vi "H2O_DIAL_NCAR_4CH_v4.08.vi"() -> ()   [LabVIEW 2012]
uses:
  C:/Users/H2ODial/Desktop/Shared Telescope WV DIAL Code/Libraries and VIs/PowerMeterCommands.dll
  Libraries and VIs/PowerMeterCommands.dll
  <vilib>/DAQmx/write.llb/DAQmx Write (Digital 1D Bool NChan 1Samp 1Line).vi
  <vilib>/DAQmx/miscellaneous.llb/DAQmx Fill In Error Info.vi
  <vilib>/Analysis/baseanly.llb/Mean (DBL).vi
  AMCS_Data.vi
  Libraries and VIs/Scalar_Data.vi
  <vilib>/Analysis/NI_AALBase.lvlib
  Libraries and VIs/Scalar_Data_2.vi
  Libraries and VIs/Scalar_Data_4.vi
  Libraries and VIs/Scalar_Data_3.vi
  Libraries and VIs/CLDevIFace.dll
panel:
  out "FileHour":i32=20
  out "L_Count":i32=53610
  out "sigma_off_total":dbl[](array[numeric])=[5.237977287539916e-25, 5.210394736135076e-25, 5.182925586949714e-25, 5.155569869487791e-25, 5.128327607320838e-25, 5.101198818125548e-25, 5.074183513766137e-25, 5.047281700299452e-25, 5.020493378072102e-25, 4.993818541757595e-25, 4.967257180403445e-25, 4.940809277499799e-25, 4.914474811031665e-25, 4.888253753539835e-25, 4.862146072166262e-25, 4.836151728727555e-25, 4.810270679757114e-25, 4.7845028765711135e-25, 4.7588482653375005e-25, 4.733306787104272e-25, 4.707878377890851e-25, 4.682562968723741e-25, 4.657360485698113e-25, 4.632270850042273e-25, 4.607293978174461e-25, 4.582429781742665e-25, 4.557678167708119e-25, 4.533039038377526e-25, 4.508512291468661e-25, 4.484097820168311e-25, 4.459795513173839e-25, 4.435605254768827e-25, 4.411526924848054e-25, 4.387560398991586e-25, 4.363705548510036e-25, 4.339962240489646e-25, 4.3163303378483935e-25, 4.292809699388025e-25, 4.269400179831349e-25, 4.246101629883972e-25, 4.222913896270031e-25, 4.199836821781227e-25, 4.176870245324587e-25, 4.154014001969199e-25, 4.1312679229794556e-25, 4.10863183586778e-25, 4.0861055644288118e-25, 4.0636889287851403e-25, 4.041381745427012e-25, 4.019183827248936e-25, 3.997094983583401e-25, 3.9751150202537046e-25, 3.953243739588023e-25, 3.9314809404746634e-25, 3.9098264183856214e-25, 3.888279965410497e-25, 3.8668413702954256e-25, 3.845510418470829e-25, 3.8242868920787765e-25, 3.8031705700147897e-25, 3.782161227940215e-25, 3.761258638329626e-25, 3.74046257048381e-25, 3.7197727905642295e-25, 3.69918906161745e-25, 3.678711143600706e-25, 3.6583387934050425e-25, 3.638071764885887e-25, 3.617909808876586e-25, 3.59785267321608e-25, 3.577900102772319e-25, 3.558051839461918e-25, 3.538307622269321e-25, 3.5186671872697243e-25, 3.4991302676454615e-25, 3.479696593706232e-25, 3.460365892905833e-25, 3.441137889863693e-25, 3.422012306375155e-25, 3.4029888614344406e-25, 3.384067271245277e-25, 3.3652472492411824e-25, 3.346528506092826e-25, 3.3279107497319426e-25, 3.309393685355381e-25, 3.2909770154454064e-25, 3.272660439778772e-25, 3.2544436554389533e-25, 3.2363263568278233e-25, 3.2183082356811116e-25, 3.2003889810704124e-25, 3.1825682794209234e-25, 3.1648458145178674e-25, 3.1472212675167257e-25, 3.1296943169518588e-25, 3.1122646387407036e-25, 3.094931906200432e-25, 3.0776957900440946e-25, 3.060555958395204e-25, 3.043512076792759e-25, 3.026563808190885e-25, 3.009710812972571e-25, 2.9929527489462136e-25, 2.976289271354231e-25, 2.9597200328732653e-25, 2.9432446836195626e-25, 2.9268628711468796e-25, 2.910574240452457e-25, 2.8943784339725194e-25, 2.8782750915848116e-25, 2.862263850606443e-25, 2.8463443457918976e-25, 2.830516209331176e-25, 2.814779070844048e-25, 2.799132557377377e-25, 2.783576293398477e-25, 2.768109900787332e-25, 2.7527329988309794e-25, 2.7374452042136163e-25, 2.7222461310065917e-25, 2.7071353906571954e-25, 2.6921125919761984e-25, 2.677177341122853e-25, 2.662329241593387e-25, 2.647567894198339e-25, 2.632892897051999e-25, 2.618303845545271e-25, 2.60380033233239e-25, 2.589381947301631e-25, 2.575048277552024e-25, 2.5607989073700278e-25, 2.546633418200283e-25, 2.532551388614268e-25, 2.5185523942817305e-25, 2.5046360079339746e-25, 2.4908017993263377e-25, 2.477049335209051e-25, 2.4633781792772914e-25, 2.4497878921362335e-25, 2.4362780312554467e-25, 2.4228481509187937e-25, 2.4094978021817806e-25, 2.3962265328170672e-25, 2.3830338872635978e-25, 2.3699194065693153e-25, 2.356882628338278e-25, 2.3439230866617374e-25, 2.3310403120653215e-25, 2.318233831442806e-25, 2.305503167989909e-25, 2.29284784112487e-25, 2.280267366433339e-25, 2.267761255593697e-25, 2.2553290162907755e-25, 2.242970152141067e-25, 2.2306841626327338e-25, 2.21847054301743e-25, 2.206328784250053e-25, 2.1942583728887336e-25, 2.182258791026811e-25, 2.1703295161891593e-25, 2.1584700212551692e-25, 2.1466797743708636e-25, 2.1349582388520993e-25, 2.1233048731028347e-25, 2.11171913052587e-25, 2.1002004594155447e-25, 2.0887483028986794e-25, 2.077362098819431e-25, 2.0660412796644763e-25, 2.0547852724613812e-25, 2.0435934987176713e-25, 2.0324653743177702e-25, 2.0214003094407255e-25, 2.0103977084918826e-25, 1.9994569700219043e-25, 1.9885774866543093e-25, 1.977758645016903e-25, 1.9669998256711833e-25, 1.9563004030651965e-25, 1.9456597454736256e-25, 1.9350772149357237e-25, 1.9245521672543692e-25, 1.9140839518990637e-25, 1.9036719120338527e-25, 1.893315384469969e-25, 1.883013699654113e-25, 1.8727661816903515e-25, 1.8625721483087474e-25, 1.8524309109152708e-25, 1.842341774622776e-25, 1.8323040382575362e-25, 1.8223169944561692e-25, 1.812379929715831e-25, 1.8024921244357534e-25, 1.7926528530972796e-25, 1.7828613842771046e-25, 1.7731169808504013e-25, 1.763418900060532e-25, 1.753766393760346e-25, 1.7441587084910652e-25, 1.7345950857732995e-25, 1.7250747622294322e-25, 1.7155969698576046e-25, 1.7061609363195063e-25, 1.6967658851005867e-25, 1.6874110359226843e-25, 1.6780956049685245e-25, 1.6688188052514317e-25, 1.659579846970255e-25, 1.65037793787203e-25, 1.6412122836350012e-25, 1.6320820883466068e-25, 1.6229865548899808e-25, 1.6139248854231656e-25, 1.604896281851196e-25, 1.5958999464323058e-25, 1.5869350821540768e-25, 1.5780008933988883e-25, 1.5690965865250916e-25, 1.5602213703998908e-25, 1.551374457088728e-25, 1.5425550624278814e-25, 1.533762406758044e-25, 1.5249957155722975e-25, 1.5162542201789217e-25, 1.5075371585159662e-25, 1.498843775813426e-25, 1.490173325365196e-25, 1.4815250692768405e-25, 1.4728982792886032e-25, 1.4642922375724935e-25, 1.4557062374752215e-25, 1.4471395844199516e-25, 1.4385915966670965e-25, 1.4300616061440924e-25, 1.4215489593499951e-25, 1.413053018080556e-25, 1.4045731604317913e-25, 1.396108781452575e-25, 1.3876592941232874e-25, 1.3792241301169086e-25, 1.3708027406484068e-25, 1.3623945973169855e-25, 1.353999192808714e-25, 1.3456160418411176e-25, 1.3372446818099923e-25, 1.3288846735970857e-25, 1.3205356022789798e-25, 1.312197077893849e-25, 1.3038687360747626e-25, 1.295550238736152e-25, 1.2872412747034491e-25, 1.2789415602527627e-25, 1.2706508397867747e-25, 1.2623688862167277e-25, 1.2540955015928698e-25, 1.2458305174038967e-25, 1.2375737951859152e-25, 1.229325226582947e-25, 1.2210847339251814e-25, 1.2128522703422863e-25, 1.2046278200669743e-25, 1.196411398536186e-25, 1.1882030524688986e-25, 1.1800028600144816e-25, 1.1718109306926895e-25, 1.163627405308368e-25, 1.15545245599885e-25, 1.1472862858176296e-25, 1.1391291287321645e-25, 1.1309812492832123e-25, 1.1228429421236803e-25, 1.1147145318495405e-25, 1.106596372364196e-25, 1.0984888464412128e-25, 1.0903923652647968e-25]
  out "sigma_on_total":dbl[](array[numeric])=[2.0666817520319192e-23, 2.0593109014659378e-23, 2.051872195703395e-23, 2.044367039943362e-23, 2.0367968427579014e-23, 2.0291630153667858e-23, 2.0214669713004497e-23, 2.013710125383857e-23, 2.0058938935289517e-23, 1.9980196920012705e-23, 1.9900889367712726e-23, 1.982103043065158e-23, 1.974063424772205e-23, 1.9659714939377124e-23, 1.9578286601133224e-23, 1.9496363299838326e-23, 1.94139590669971e-23, 1.9331087894484655e-23, 1.9247763730742107e-23, 1.9164000472908787e-23, 1.9079811965513556e-23, 1.8995211993589887e-23, 1.891021427856131e-23, 1.8824832474616412e-23, 1.8739080164441743e-23, 1.8652970853194722e-23, 1.856651796748594e-23, 1.847973484883867e-23, 1.8392634751030097e-23, 1.8305230836795774e-23, 1.8217536172790674e-23, 1.8129563728772394e-23, 1.804132637094709e-23, 1.7952836861392256e-23, 1.7864107854248313e-23, 1.7775151892040785e-23, 1.7685981403601007e-23, 1.7596608701730099e-23, 1.750704597915161e-23, 1.741730530788138e-23, 1.732739863541907e-23, 1.7237337782890177e-23, 1.7147134443297577e-23, 1.7056800179881565e-23, 1.6966346422793058e-23, 1.6875784468765622e-23, 1.6785125478376762e-23, 1.669438047521509e-23, 1.6603560344433225e-23, 1.6512675831053983e-23, 1.6421737538036553e-23, 1.6330755927613498e-23, 1.6239741316742248e-23, 1.6148703879339332e-23, 1.60576536436924e-23, 1.596660049173217e-23, 1.5875554159429494e-23, 1.5784524235547823e-23, 1.569352016050113e-23, 1.5602551228033537e-23, 1.5511626581860282e-23, 1.5420755218867996e-23, 1.5329945986273844e-23, 1.523920758294004e-23, 1.5148548559068197e-23, 1.505797731630872e-23, 1.4967502107612878e-23, 1.4877131038805498e-23, 1.4786872066923908e-23, 1.4696733001603334e-23, 1.4606721505852176e-23, 1.4516845096236347e-23, 1.4427111143132646e-23, 1.4337526872006215e-23, 1.4248099363455505e-23, 1.415883555427735e-23, 1.4069742237945813e-23, 1.3980826066400498e-23, 1.3892093549366116e-23, 1.3803551056859226e-23, 1.371520481892078e-23, 1.36270609278781e-23, 1.3539125337562842e-23, 1.3451403866865457e-23, 1.3363902198427942e-23, 1.32766258816433e-23, 1.3189580332947156e-23, 1.3102770837058438e-23, 1.301620254824897e-23, 1.2929880492812047e-23, 1.2843809568021667e-23, 1.2757994545539253e-23, 1.2672440071893687e-23, 1.2587150670157126e-23, 1.2502130741345343e-23, 1.241738456470468e-23, 1.2332916301710505e-23, 1.224872999440041e-23, 1.2164829569109985e-23, 1.2081218837654899e-23, 1.1997901497162132e-23, 1.1914881134062081e-23, 1.1832161223390686e-23, 1.1749745131680931e-23, 1.1667636117668732e-23, 1.1585837334629664e-23, 1.1504351830839475e-23, 1.1423182552440761e-23, 1.1342332343652275e-23, 1.1261803949102824e-23, 1.1181600015104835e-23, 1.1101723091192649e-23, 1.1022175631912938e-23, 1.0942959997845036e-23, 1.086407845764062e-23, 1.0785533189291783e-23, 1.070732628140394e-23, 1.0629459735209997e-23, 1.0551935465825773e-23, 1.0474755303750616e-23, 1.0397920996360129e-23, 1.0321434209390468e-23, 1.0245296528176247e-23, 1.0169509459831485e-23, 1.0094074433518565e-23, 1.0018992803312205e-23, 9.944265848224308e-24, 9.869894775025579e-24, 9.795880718494269e-24, 9.72222474305659e-24, 9.648927844628867e-24, 9.575990951759402e-24, 9.50341492676679e-24, 9.431200567532366e-24, 9.359348608388352e-24, 9.287859721227397e-24, 9.216734517894411e-24, 9.14597355017344e-24, 9.075577311930703e-24, 9.005546240155555e-24, 8.935880715787577e-24, 8.86658106558043e-24, 8.797647562896506e-24, 8.729080429115388e-24, 8.660879834613277e-24, 8.593045900337285e-24, 8.525578698151898e-24, 8.458478252785328e-24, 8.391744542743954e-24, 8.325377501414138e-24, 8.259377017376947e-24, 8.193742936655974e-24, 8.128475063566239e-24, 8.063573160991183e-24, 7.99903695161361e-24, 7.934866120048426e-24, 7.87106031214778e-24, 7.807619137288812e-24, 7.744542168412114e-24, 7.681828943883436e-24, 7.619478967515311e-24, 7.557491710029518e-24, 7.495866609952388e-24, 7.434603074147054e-24, 7.373700479036967e-24, 7.313158171455071e-24, 7.252975468799607e-24, 7.193151661058425e-24, 7.133686010591324e-24, 7.074577753436494e-24, 7.015826099592955e-24, 6.95743023461463e-24, 6.89938931969699e-24, 6.841702492422132e-24, 6.784368867806759e-24, 6.727387538848196e-24, 6.67075757722047e-24, 6.61447803395679e-24, 6.558547939965e-24, 6.502966306993674e-24, 6.447732128116975e-24, 6.392844378064806e-24, 6.33830201474097e-24, 6.28410397847858e-24, 6.23024919382799e-24, 6.1767365695383454e-24, 6.123564999129965e-24, 6.070733361880125e-24, 6.0182405226492204e-24, 5.966085332987157e-24, 5.914266631645723e-24, 5.8627832445313994e-24, 5.811633985898412e-24, 5.7608176585519654e-24, 5.710333053788294e-24, 5.66017895307138e-24, 5.610354127145003e-24, 5.560857337543025e-24, 5.5116873361021744e-24, 5.4628428664272046e-24, 5.4143226631411985e-24, 5.3661254534434446e-24, 5.318249956485201e-24, 5.27069488426681e-24, 5.223458942376564e-24, 5.176540829250344e-24, 5.129939237757062e-24, 5.083652854692084e-24, 5.037680361483587e-24, 4.99202043452124e-24, 4.946671745361136e-24, 4.9016329609288464e-24, 4.8569027442871215e-24, 4.812479754472342e-24, 4.768362646904479e-24, 4.724550073562594e-24, 4.6810406839229e-24, 4.637833124122778e-24, 4.594926037999457e-24, 4.552318067336052e-24, 4.510007851680585e-24, 4.467994029014724e-24, 4.426275235567218e-24, 4.384850106461307e-24, 4.3437172757252515e-24, 4.302875376308277e-24, 4.262323040796395e-24, 4.222058901208864e-24, 4.182081589298348e-24, 4.142389736646627e-24, 4.102981975046665e-24, 4.063856936678659e-24, 4.0250132539999516e-24, 3.986449560294931e-24, 3.948164489555187e-24, 3.910156676643546e-24, 3.872424757723072e-24, 3.834967369951946e-24, 3.797783152259275e-24, 3.760870744768346e-24, 3.724228789468588e-24, 3.687855930080657e-24, 3.651750812271991e-24, 3.615912083862758e-24, 3.580338394607038e-24, 3.545028396812783e-24, 3.509980745031705e-24, 3.475194096334501e-24, 3.440667110332911e-24, 3.40639844943986e-24, 3.3723867788033646e-24, 3.33863076647876e-24, 3.305129083516007e-24, 3.271880403891816e-24, 3.238883404898292e-24, 3.2061367668408557e-24, 3.173639173491545e-24, 3.1413893117883693e-24, 3.1093858724187726e-24, 3.0776275491566985e-24, 3.0461130395819077e-24, 3.0148410447789974e-24, 2.983810269608433e-24, 2.9530194226199734e-24, 2.9224672160398477e-24, 2.8921523660272985e-24, 2.8620735925846947e-24, 2.8322296195392698e-24, 2.8026191749155588e-24, 2.773240990450988e-24, 2.744093802094081e-24, 2.7151763499066755e-24, 2.6864873778481257e-24, 2.6580256342491748e-24, 2.6297898714658192e-24, 2.601778846035958e-24, 2.5739913188856307e-24]
  out "background start":u32=269
  in  "Tab Control 2":enum32{"WV ND far", "WV ND near"}(tab)
  out "Water Vapor Number Density":dbl[][](graph)=[[1.726093583785998, 1.5693328403021882, 1.492935828673154, 1.447945915792696, 1.4070653390472017, 1.3254550070570101, 1.2804967879324003, 1.2804658654967171, 1.1579952104203475, 0.9405002139474755, 0.8165160638391011, 0.7588336527077482, 0.7354590874335223, 0.7949133332346723, 0.934908558804581, 1.2546910246889589, 1.7625302263189773, 2.0654043072611956, 1.7505301065732377, 1.188350440813126, 0.9885074031875984, 1.101505088269768, 1.2336330855194724, 1.3310674253591945, 1.505107272437263, 1.8254736972087702, 2.225603030680858, 2.067084599300453, 0.8832035531037339, 0.09437092170191938, 0.5395557458682886, 1.2140813710589395, 1.531090454107329, 1.5864605833339975, 1.5242315918950318, 1.3208543677687434, 1.1426796573454, 1.0502932702090415, 1.053417044203025, 1.1120228404679369, 0.8980388027038368, 0.8252375109823104, 0.7459206585905861, 0.6947605707599939, 0.5975172515547873, 0.4760902556721864, 0.4151454819859171, 0.39114402110892216, 0.37598278988553024, 0.34134053721693014, 0.29078994347279413, 0.27415101735234926, 0.3077369235432359, 0.3546026534730858, 0.46199415649911274, 0.5308578319039414, 0.5880944648414834, 0.8235212196286621, 1.2285880343893505, 2.882707728529924, 21.655039035254283, -1.2950791268227064, -15.65393062619791, -8.993125447341491, -5.175372303539384, -3.3856480323932954, -6.29508550326919, -7.154473265737363, -6.483534196194922, -9.265253216386386, -27.54820579914408, -4.723304671265731, 12.404282083102887, 2.1871104315302006, -2.728312257847411, -2.37955818251216, -0.8921430715770072, 0.0602736205824744, -0.33680772359773153, -1.5016597305177382, -3.146854610737365, 5.147107349586582, 2.5981969564643483, 1.927078112036158, -0.2019670065149347, -2.7680462725589408, -0.8640403008156559, -0.3802637288627016, -0.30703778771168194, 3.78203982209544, 6.186195002061386, -1.7005858912590297, -4.265240893190755, -3.1735701916943326, 0.5020833614372952, 3.237847342695031, 3.4070293883563316, 2.220676402431187, -0.36304323573622177, -2.50058383327132, -4.668332258495944, -6.411554489859993, -3.6540172117701606, 1.1929008673292896, 6.604569777453038, 9.439096094131198, -0.37592110290192393, -1.1973823785952542, -1.48647731353954, -4.840730889441363, -3.3418602691261685, -0.6598739403508244, 0.669104742362441, -0.6893546278444684, -10.4814271416847, -11.440111754869928, -0.3632022671713595, 0.6227468083328052, 13.218505806822774, 8.015075479380561, 4.061945777588537, -0.04892863519373536, -6.238185623258318, 18.53116155726855, 15.923168701202894, -3.9495930624327413, -5.7591651615962505, -2.835335920357439, -15.615692769445864, -8.050161480731097, -6.2988354876816945, 3.427472591088481, 9.602428466947865, -24.99205539862618, -21.730434892627393, 2.0254153667718473, 5.319236625213819, -4.231429520416637, 5.960092104774531, 9.175230031410537, 5.788798488819853, 1.2095983409811533, -4.077619187880176, 2.2911716100459993, 8.947839474381412, 1.5428868263761497, 1.1797809535068915, 6.502768356706267, -5.016648532788809, -8.952003568032467, -0.620404792879008, 24.678168336180246, 56.15693255842815, 15.239179864782777, 11.41921009773234, 9.58559110034771, -1.8378094145353232, -8.922747471661737, -10.47837694939924, 0.3826205789632058, 18.765420881082978, -27.679590849047152, -97.04153207449242, -10.013514694974337, 6.267103457434482, 5.2850126899119845, 14.69530339344026, 2.3301310125680486, 22.67928054652624, -4.859966072588231, -27.611523100524643, -5.388011297923277, 42.80888421591542, -10.55670454003978, -29.387589282014147, -13.771657285473296, -10.230767774708267, -15.406236525942628, -17.934779899787376, 7.866413980735036, -16.61338646328196, -33.72812563272742, -31.126096535992467, -6.559728776164742, 47.49568241841293, 13.927413516339834, -1.9103285022235699, 30.194286473319444, 21.421181182090656, 8.458291065822397, 64.4520154677842, 51.90400411679242, 36.48500116306378, 20.23053272363266, -21.8380131234608, 9.733997218213648, 17.755970175135474, 24.978768220528003, -16.798275313105552, -40.83054382894082, -72.77210575173487, -23.204625740736503, -12.922468776734748, 10.063889955334702, -12.711982906467439, -20.40456545648094, -13.878406439439372, -29.749691947295048, -4.076124591492557, 29.788213178427508, 6.248079314213002, -20.245927416281017, -13.548384416231665, -13.091969559034965, -12.979461901579612, -27.404428517975767, -28.82133765520021, -34.93474155125817, -17.456376797105253, -21.723899533014873, 8.609611112888343, 31.6981010680414, 21.03013721810904, -20.578242782300084, 33.02437661787703, 0.05405579004919296, 0.5355916211190656, 36.99850340913583, 14.120107902899404, 19.11249102647391, -23.861285040548577, -37.522374332023944, -28.734364047495777, 24.270546317192423, -42.885420861437105, 7.644261246136678, -10.35463621262086, -4.297514158130115, 7.187709131614377, -4.734831899416053, 48.535485170482076, 109.9250199786216, 19.771496935630168, -21.29480194803723, 7.10371336563834, -7.3594100417697, 28.30301499602303, -6.173312274600606, -48.473804438854806, -44.552722047320536, -16.388748920234434, -52.98268299759962, 35.83782137376554, 16.24116595319644, 9.54744614996322, 28.184236323160842, 21.73885851975668, 13.761566677706107, 58.90182142368742, 82.80959093536396, 97.24340862705938, -19.983802413261767, -110.5470598503176, -45.4894502592988, -12.240067151016795, -53.090407850417165, -6.950497574763418, -78.83310574737847, 10.93122749802334, -11.422884686238413, -159.94669283010876, -73.71618130213747, 9.079012315082618, -28.203429472131308, -56.05728304279368, -26.34758679382537, 0.0, 0.0, 0.0, 0.0]]
  out "Water Vapor Number Density 2":dbl[][](graph)=[[nan, nan, nan, nan, nan, nan, nan, nan, nan, nan, nan, nan, nan, nan, nan, nan, nan, nan, nan, nan, nan, nan, nan, nan, nan, nan, nan, nan, nan, nan, nan, nan, nan, nan, nan, nan, nan, nan, nan, nan, nan, nan, nan, nan, nan, nan, nan, nan, nan, nan, nan, nan, nan, nan, nan, nan, nan, nan, nan, nan, nan, nan, nan, nan, nan, nan, nan, nan, nan, nan, nan, nan, nan, nan, nan, nan, nan, nan, nan, nan, nan, nan, nan, nan, nan, nan, nan, nan, nan, nan, nan, nan, nan, nan, nan, nan, nan, nan, nan, nan, nan, nan, nan, nan, nan, nan, nan, nan, nan, nan, nan, nan, nan, nan, nan, nan, nan, nan, nan, nan, nan, nan, nan, nan, nan, nan, nan, nan, nan, nan, nan, nan, nan, nan, nan, nan, nan, nan, nan, nan, nan, nan, nan, nan, nan, nan, nan, nan, nan, nan, nan, nan, nan, nan, nan, nan, nan, nan, nan, nan, nan, nan, nan, nan, nan, nan, nan, nan, nan, nan, nan, nan, nan, nan, nan, nan, nan, nan, nan, nan, nan, nan, nan, nan, nan, nan, nan, nan, nan, nan, nan, nan, nan, nan, nan, nan, nan, nan, nan, nan, nan, nan, nan, nan, nan, nan, nan, nan, nan, nan, nan, nan, nan, nan, nan, nan, nan, nan, nan, nan, nan, nan, nan, nan, nan, nan, nan, nan, nan, nan, nan, nan, nan, nan, nan, nan, nan, nan, nan, nan, nan, nan, nan, nan, nan, nan, nan, nan, nan, nan, nan, nan, nan, nan, nan, nan, nan, nan, nan, nan, nan, nan, nan, nan, nan, nan, nan, nan, nan, nan, nan, nan, nan, nan, nan, nan, 0.0, 0.0, 0.0, 0.0]] caption="Water Vapor Number Density"
  out "RingBuffer offline near":dbl[][](array[numeric])
  out "RingBuffer aerosol near":dbl[][](array[numeric])
  in  "?":T1(tab)
  out "NRB":dbl[][](graph)=[[0.00038821040544486485, 0.0028581072475373126, 0.009664054878145745, 0.0218937455043181, 0.041585081911817263, 0.07907105171256666, 0.1517956195167564, 0.26417801899826343, 0.4035088182229872, 0.5650687115263837, 0.7608077401440904, 1.0057587682792892, 1.2933461609750239, 1.5966324534478469, 1.8616436253029935, 2.051331796764738, 2.160120670777728, 2.2276009194819837, 2.3041185987927006, 2.3534797914467314, 2.4144079717154505, 2.5498196394788026, 2.6670946659124346, 2.7292203147350245, 2.8081805686949957, 2.85157014135836, 2.8104801837455016, 2.52779119302893, 1.896358445357234, 1.4744417690314884, 1.9842591872797726, 3.185501611912857, 3.9632337336496595, 3.867773398872155, 3.446687058785667, 3.1391414455490154, 2.967862705818635, 2.835829374555156, 2.61630220135343, 2.2701613602887263, 1.9304871996773967, 1.7247991727133216, 1.6336047893811358, 1.5809857912833423, 1.4964246235970382, 1.3753026836922766, 1.2068633615280102, 0.9758258849560736, 0.7472068994762533, 0.5990670480551521, 0.5531735761691717, 0.5643122449388852, 0.6046034091465748, 0.6816394574095734, 0.7768790871537363, 0.8963666224831853, 1.0673032706932424, 1.1963682953128685, 1.113329958933323, 0.8104505672194267, 0.4712408220023341, 0.23636168910826832, 0.11093337571666789, 0.045649279610657616, 0.013827815106420362, 0.000595543364686196, -0.004059439261428629, -0.002311182614261961, 0.0011883714622039875, -0.0071350992474156815, -0.013583214093101, -0.009986650833171679, -0.009129851870763993, -0.007802145173723816, -0.007450071158263493, -0.005784710331142982, -0.004246214811760087, -0.0036513842538617087, -0.007639759654127067, -0.009499909569249076, -0.008196050807191971, -0.004014404234963711, -0.0025144302656745997, -0.006602038304925129, -0.006737511480302444, -0.010236280891107273, -0.018639054498064318, -0.013631519426649653, -0.00435649140769087, -0.007934433790837766, -0.008838747504431614, -0.009538302637566698, -0.0025601741269936887, -0.0008145882550386953, -0.006378604787752585, -0.006369112164930518, -0.010839258183081239, -0.006275890418726249, -0.0014874755507115693, -0.009137146169405736, -0.012711182042689725, -0.013910133853955842, -0.017011569135408258, -0.012799263424370013, -0.011249036980201734, -0.009491427382456405, -0.0003733679388180713, -0.007329445907503577, -0.008732421530258959, -0.010562733558625092, -0.017129887166000557, -0.013428203058959441, -0.007903693902916552, -0.0071477038674852365, -0.01108866845659684, -0.003265799105280196, 0.0011847288805150722, 0.00037549107141904574, -0.008054862709676584, -0.003856137038819446, -0.0002938238582222133, -0.008979477671617945, -0.013823588439693935, -0.01684551058225059, -0.021282526470720726, -0.015053701873621683, -0.002498437111966955, -0.007161630455462848, -0.009100247718271013, 0.004854268428875897, -0.005079795143177093, -0.016466890516066177, -0.005735284286529295, -0.005652942916379182, -0.007623473296299922, -0.023801251769537502, -0.01903270232093059, -0.0044428719473701955, -0.009535919044250532, -0.010042365596353318, -0.0005860062665582348, -0.001163403080465544, -0.007078999820003343, -0.0045125020394603645, -0.013409503799712511, -0.009517978818285977, -0.003415066647501558, -0.016579995519609127, -0.02926505443225014, -0.02697842152514472, -0.02926957498007797, -0.028861691487481075, -0.021902935753967165, -0.018174655782106284, -0.0031188766495679264, -0.007585198059561486, -0.016571020297115692, -0.021635854085040027, -0.029441021440962507, -0.019217103588233597, 0.0017556718697036378, 0.012229072279566435, -0.0002832635082702486, -0.003491584031915878, -0.003022079844493582, -0.028893566916345426, -0.026881714889429913, 0.0045667551264583755, 0.01850339913989443, 0.005310498553660611, -0.009572465171618721, -0.014322953367776099, 0.005030331004590102, 0.018285288530946343, 0.003322697023046563, 0.010062997059378718, -0.0016111136822627265, -0.01782335625220735, -0.01621577106262897, 0.0008737367648647722, 0.006328165945234042, -0.005754217184822082, 0.005733693099793122, -0.0006794413321474801, -0.0073406170620529555, -0.02141406486532235, -0.007280889001977234, 0.003723861056545976, -0.00161295411575233, 0.006407127430732478, -0.01731893407410713, -0.009062562045596382, 0.022963886135369878, 0.005027499489036191, -0.03653239986567297, -0.030162663971345347, -0.03667720121889417, -0.06790332618629877, -0.05716805413017849, -0.012467452431889361, 0.0029897995541221982, 0.012232140362994913, 0.003695696789507197, -0.0008351733955177691, 0.01892372231648461, 0.017245790039927242, -0.0370021118681977, -0.04902663445060557, -0.0014244986405373553, -0.006416390139489504, -0.00452319036422678, -0.020491087142077, -0.0006259625245654467, 0.017749631746947835, 0.0057399871570086676, 0.022764711172768803, 0.013968583721646131, -0.01049104015112462, 0.0006918038827279306, 0.010866731057858372, 0.033632981827137316, 0.04104733648520129, -0.0038048271117926127, -0.026023118468938237, 0.022002518883890095, 0.02556201173658669, -0.012829349484035735, 0.012649468345009815, 0.0009208650264830834, -0.022791436909489662, 0.008132040402759338, 0.05411197756684636, 0.04044899497686315, 0.002850213426684236, 0.013091767075097282, 0.029795377253195882, 0.0039805495316438755, -0.03097616920580153, -0.025505557706854635, 0.015280377374667527, 0.010126247818250977, -0.0274353172351386, -0.018589921266945548, -0.0023149273070895648, -7.528853128950785e-05, 0.008842912384514965, 0.03282895809715373, 0.01631604739672833, -0.012714802365824892, -0.01634474961766888, 0.0034769443788520075, -0.011230881393592969, 0.014571969435003957, 0.04908038439702908, -0.0021205563998292513, -0.0296739970695606, -0.03632646142994246, -0.04203632491958742, -0.02890117919329823, -0.03505984551379594, -0.016533107970480992, 0.02294574713598894, 0.008155264467048293, 0.013025488006695554, 0.018189171644197748, 0.05293991300397336, 0.08776686908236478, 0.039324200183096444, 0.020330781454769957, 0.022996810288827076, 0.000598754452566444, 0.009186959650062287, 0.013928727554680512, -0.02081063470678285, -0.01764294218755887, 0.055800776768044166, 0.0003849606095558099, 0.0, 0.0, 0.0]] caption="Water Vapor Number Density"
  out "NRB 2":dbl[][](graph) caption="Water Vapor Number Density"
  out "raw counts":dbl[][](graph)=[[1536.2, 3282.2, 5113.2, 6210.2, 6925.2, 8279.2, 12949.2, 18948.2, 23829.2, 24652.2, 24962.2, 28639.2, 33198.2, 34593.2, 33862.2, 32369.2, 30712.2, 29082.2, 28407.2, 25961.2, 24539.2, 22891.2, 20854.2, 20529.2, 19585.2, 17579.2, 16297.2, 14803.2, 11842.2, 8095.2, 8579.2, 12848.2, 17861.2, 19781.2, 17962.2, 15565.2, 13449.2, 11386.2, 9483.2, 8628.2, 7467.2, 6371.2, 5698.2, 5186.2, 4852.2, 4632.2, 3935.2, 2882.2, 2145.2, 1587.2, 1262.2, 972.2, 851.2, 1090.2, 1417.2, 1521.2, 1385.2, 1105.2, 658.2, 279.2, 133.2, 60.19999999999999, 72.19999999999999, 44.19999999999999, 8.199999999999989, -1.8000000000000114, -3.8000000000000114, -21.80000000000001, -12.800000000000011, -29.80000000000001, -16.80000000000001, -23.80000000000001, -59.80000000000001, -20.80000000000001, -39.80000000000001, -63.80000000000001, -14.800000000000011, -41.80000000000001, -40.80000000000001, -23.80000000000001, -26.80000000000001, -28.80000000000001, 6.199999999999989, -32.80000000000001, -55.80000000000001, -52.80000000000001, -34.80000000000001, -60.80000000000001, -48.80000000000001, -21.80000000000001, -17.80000000000001, -2.8000000000000114, -24.80000000000001, -20.80000000000001, -22.80000000000001, 4.199999999999989, -3.8000000000000114, -53.80000000000001, 8.199999999999989, -24.80000000000001, -20.80000000000001, 4.199999999999989, 8.199999999999989, -18.80000000000001, -10.800000000000011, -31.80000000000001, -38.80000000000001, -31.80000000000001, -21.80000000000001, 3.1999999999999886, -36.80000000000001, -38.80000000000001, -46.80000000000001, -81.80000000000001, -7.800000000000011, -16.80000000000001, 22.19999999999999, 6.199999999999989, -8.800000000000011, -24.80000000000001, -0.8000000000000114, -4.800000000000011, -6.800000000000011, -6.800000000000011, -18.80000000000001, -18.80000000000001, -5.800000000000011, 15.199999999999989, -27.80000000000001, 13.199999999999989, -71.80000000000001, -32.80000000000001, -40.80000000000001, -33.80000000000001, -2.8000000000000114, -18.80000000000001, -3.8000000000000114, -57.80000000000001, 1.1999999999999886, -21.80000000000001, -40.80000000000001, -8.800000000000011, -13.800000000000011, -25.80000000000001, -52.80000000000001, -42.80000000000001, 6.199999999999989, 13.199999999999989, -30.80000000000001, 17.19999999999999, -41.80000000000001, -1.8000000000000114, -29.80000000000001, -53.80000000000001, -16.80000000000001, -21.80000000000001, -14.800000000000011, 21.19999999999999, 11.199999999999989, -45.80000000000001, -66.80000000000001, -7.800000000000011, -7.800000000000011, -5.800000000000011, -45.80000000000001, 4.199999999999989, -20.80000000000001, -60.80000000000001, -37.80000000000001, -18.80000000000001, -60.80000000000001, -17.80000000000001, -42.80000000000001, -12.800000000000011, -42.80000000000001, 23.19999999999999, -3.8000000000000114, 6.199999999999989, -14.800000000000011, -49.80000000000001, -41.80000000000001, -45.80000000000001, -7.800000000000011, -28.80000000000001, 33.19999999999999, -24.80000000000001, -37.80000000000001, 36.19999999999999, -14.800000000000011, -18.80000000000001, -3.8000000000000114, 5.199999999999989, -24.80000000000001, -1.8000000000000114, -1.8000000000000114, -3.8000000000000114, 18.19999999999999, -34.80000000000001, -29.80000000000001, -8.800000000000011, 15.199999999999989, -48.80000000000001, -10.800000000000011, -39.80000000000001, 28.19999999999999, -21.80000000000001, -59.80000000000001, -23.80000000000001, -1.8000000000000114, 9.199999999999989, -23.80000000000001, -21.80000000000001, -28.80000000000001, -0.8000000000000114, -16.80000000000001, -21.80000000000001, 25.19999999999999, 13.199999999999989, -26.80000000000001, -7.800000000000011, 14.199999999999989, -14.800000000000011, -31.80000000000001, 9.199999999999989, -30.80000000000001, -18.80000000000001, -19.80000000000001, 6.199999999999989, -37.80000000000001, -9.800000000000011, -3.8000000000000114, 2.1999999999999886, -7.800000000000011, -41.80000000000001, 6.199999999999989, -22.80000000000001, -34.80000000000001, -9.800000000000011, -26.80000000000001, 39.19999999999999, -11.800000000000011, -19.80000000000001, -11.800000000000011, -0.8000000000000114, -34.80000000000001, -7.800000000000011, -20.80000000000001, -35.80000000000001, -35.80000000000001, -10.800000000000011, 4.199999999999989, -42.80000000000001, -40.80000000000001, 10.199999999999989, -34.80000000000001, -75.80000000000001, -52.80000000000001, -31.80000000000001, -32.80000000000001, 35.19999999999999, -27.80000000000001, -29.80000000000001, -17.80000000000001, -12.800000000000011, -22.80000000000001, -21.80000000000001, -24.80000000000001, -3.8000000000000114, -0.8000000000000114, 29.19999999999999, 43.19999999999999, -34.80000000000001, -36.80000000000001, -37.80000000000001, -13.800000000000011, 14.199999999999989, 28.19999999999999, 16.19999999999999, -7.800000000000011, 0.0]] caption="Water Vapor Number Density"
  out "raw counts near":dbl[][](graph) caption="Water Vapor Number Density"
  out "Aerosol Smoothed 2":dbl[](array[numeric])
  out "Off-Line Smoothed 2":dbl[](array[numeric])
  out "Off-Line Bin Readings 2":dbl[](array[numeric])
  out "On-Line Smoothed 2":dbl[](array[numeric])
  out "On-Line Bin Readings 2":dbl[](array[numeric])
  in  "stop":bool
  in  "Reset Average":bool=TRUE
  in  "Save Data?":bool=TRUE
  in  "Collect Data?":bool=TRUE
  in  "ILX Address":i32=6 min=0 step=1
  in  "Lambda On DBR Current":dbl=170.6899999999991
  in  "Lambda Off DBR Current":dbl=172.7499999999999
  in  "Tab Control":T2(tab)=enum."g/m^3"
  out "Water Vapor Number Density  2":cluster{"Y":dbl[], "Y":dbl[]}[](graph)=[{"Y"=array[276 elements], "Y"=array[280 elements]}, {"Y"=[nan, nan, nan, nan, nan, nan, nan, nan, nan, nan, nan, nan, nan, nan, nan, nan, nan, nan, nan, nan, nan, nan, nan, nan, nan, nan, nan, nan, nan, nan, nan, nan, nan, nan, nan, nan, nan, nan, nan, nan, nan, nan, nan, nan, nan, nan, nan, nan, nan, nan, nan, nan, nan, nan, nan, nan, nan, nan, nan, nan, nan, nan, nan, nan, nan, nan, nan, nan, nan, nan, nan, nan, nan, nan, nan, nan, nan, nan, nan, nan, nan, nan, nan, nan, nan, nan, nan, nan, nan, nan, nan, nan, nan, nan, nan, nan, nan, nan, nan, nan, nan, nan, nan, nan, nan, nan, nan, nan, nan, nan, nan, nan, nan, nan, nan, nan, nan, nan, nan, nan, nan, nan, nan, nan, nan, nan, nan, nan, nan, nan, nan, nan, nan, nan, nan, nan, nan, nan, nan, nan, nan, nan, nan, nan, nan, nan, nan, nan, nan, nan, nan, nan, nan, nan, nan, nan, nan, nan, nan, nan, nan, nan, nan, nan, nan, nan, nan, nan, nan, nan, nan, nan, nan, nan, nan, nan, nan, nan, nan, nan, nan, nan, nan, nan, nan, nan, nan, nan, nan, nan, nan, nan, nan, nan, nan, nan, nan, nan, nan, nan, nan, nan, nan, nan, nan, nan, nan, nan, nan, nan, nan, nan, nan, nan, nan, nan, nan, nan, nan, nan, nan, nan, nan, nan, nan, nan, nan, nan, nan, nan, nan, nan, nan, nan, nan, nan, nan, nan, nan, nan, nan, nan, nan, nan, nan, nan, nan, nan, nan, nan, nan, nan, nan, nan, nan, nan, nan, nan, nan, nan, nan, nan, nan, nan, nan, nan, nan, nan, nan, nan, nan, nan, nan, nan, nan, nan], "Y"=array[280 elements]}]
  out "Absolute Humidity":cluster{"Y":dbl[], "Y":dbl[]}[](graph)=[{"Y"=array[276 elements], "Y"=array[280 elements]}, {"Y"=[nan, nan, nan, nan, nan, nan, nan, nan, nan, nan, nan, nan, nan, nan, nan, nan, nan, nan, nan, nan, nan, nan, nan, nan, nan, nan, nan, nan, nan, nan, nan, nan, nan, nan, nan, nan, nan, nan, nan, nan, nan, nan, nan, nan, nan, nan, nan, nan, nan, nan, nan, nan, nan, nan, nan, nan, nan, nan, nan, nan, nan, nan, nan, nan, nan, nan, nan, nan, nan, nan, nan, nan, nan, nan, nan, nan, nan, nan, nan, nan, nan, nan, nan, nan, nan, nan, nan, nan, nan, nan, nan, nan, nan, nan, nan, nan, nan, nan, nan, nan, nan, nan, nan, nan, nan, nan, nan, nan, nan, nan, nan, nan, nan, nan, nan, nan, nan, nan, nan, nan, nan, nan, nan, nan, nan, nan, nan, nan, nan, nan, nan, nan, nan, nan, nan, nan, nan, nan, nan, nan, nan, nan, nan, nan, nan, nan, nan, nan, nan, nan, nan, nan, nan, nan, nan, nan, nan, nan, nan, nan, nan, nan, nan, nan, nan, nan, nan, nan, nan, nan, nan, nan, nan, nan, nan, nan, nan, nan, nan, nan, nan, nan, nan, nan, nan, nan, nan, nan, nan, nan, nan, nan, nan, nan, nan, nan, nan, nan, nan, nan, nan, nan, nan, nan, nan, nan, nan, nan, nan, nan, nan, nan, nan, nan, nan, nan, nan, nan, nan, nan, nan, nan, nan, nan, nan, nan, nan, nan, nan, nan, nan, nan, nan, nan, nan, nan, nan, nan, nan, nan, nan, nan, nan, nan, nan, nan, nan, nan, nan, nan, nan, nan, nan, nan, nan, nan, nan, nan, nan, nan, nan, nan, nan, nan, nan, nan, nan, nan, nan, nan, nan, nan, nan, nan, nan, nan], "Y"=array[280 elements]}]
  out "NRB plot":cluster{"Y":dbl[], "Y":dbl[]}[](graph)
  in  "background length":i32=10
  out "Correction":cluster{"Y":dbl[], "Y":dbl[]}[](graph)=[{"Y"=array[277 elements], "Y"=array[280 elements]}, {"Y"=[1.0, 1.0, 1.0, 1.0, 1.0, 1.0, 1.0, 1.0, 1.0, 1.0, 1.0, 1.0, 1.0, 1.0, 1.0, 1.0, 1.0, 1.0, 1.0, 1.0, 1.0, 1.0, 1.0, 1.0, 1.0, 1.0, 1.0, 1.0, 1.0, 1.0, 1.0, 1.0, 1.0, 1.0, 1.0, 1.0, 1.0, 1.0, 1.0, 1.0, 1.0, 1.0, 1.0, 1.0, 1.0, 1.0, 1.0, 1.0, 1.0, 1.0, 1.0, 1.0, 1.0, 1.0, 1.0, 1.0, 1.0, 1.0, 1.0, 1.0, 1.0, 1.0, 1.0, 1.0, 1.0, 1.0, 1.0, 1.0, 1.0, 1.0, 1.0, 1.0, 1.0, 1.0, 1.0, 1.0, 1.0, 1.0, 1.0, 1.0, 1.0, 1.0, 1.0, 1.0, 1.0, 1.0, 1.0, 1.0, 1.0, 1.0, 1.0, 1.0, 1.0, 1.0, 1.0, 1.0, 1.0, 1.0, 1.0, 1.0, 1.0, 1.0, 1.0, 1.0, 1.0, 1.0, 1.0, 1.0, 1.0, 1.0, 1.0, 1.0, 1.0, 1.0, 1.0, 1.0, 1.0, 1.0, 1.0, 1.0, 1.0, 1.0, 1.0, 1.0, 1.0, 1.0, 1.0, 1.0, 1.0, 1.0, 1.0, 1.0, 1.0, 1.0, 1.0, 1.0, 1.0, 1.0, 1.0, 1.0, 1.0, 1.0, 1.0, 1.0, 1.0, 1.0, 1.0, 1.0, 1.0, 1.0, 1.0, 1.0, 1.0, 1.0, 1.0, 1.0, 1.0, 1.0, 1.0, 1.0, 1.0, 1.0, 1.0, 1.0, 1.0, 1.0, 1.0, 1.0, 1.0, 1.0, 1.0, 1.0, 1.0, 1.0, 1.0, 1.0, 1.0, 1.0, 1.0, 1.0, 1.0, 1.0, 1.0, 1.0, 1.0, 1.0, 1.0, 1.0, 1.0, 1.0, 1.0, 1.0, 1.0, 1.0, 1.0, 1.0, 1.0, 1.0, 1.0, 1.0, 1.0, 1.0, 1.0, 1.0, 1.0, 1.0, 1.0, 1.0, 1.0, 1.0, 1.0, 1.0, 1.0, 1.0, 1.0, 1.0, 1.0, 1.0, 1.0, 1.0, 1.0, 1.0, 1.0, 1.0, 1.0, 1.0, 1.0, 1.0, 1.0, 1.0, 1.0, 1.0, 1.0, 1.0, 1.0, 1.0, 1.0, 1.0, 1.0, 1.0, 1.0, 1.0, 1.0, 1.0, 1.0, 1.0, 1.0, 1.0, 1.0, 1.0, 1.0, 1.0, 1.0, 1.0, 1.0, 1.0, 1.0, 1.0, 1.0, 1.0, 1.0, 1.0, 1.0, 1.0, 1.0, 1.0, 1.0, 1.0, 1.0, 1.0, 1.0, 1.0, 1.0, 1.0, 1.0, 1.0, 1.0], "Y"=array[280 elements]}]
  in  "dead time":dbl=3.7e-08
  out "Optical Depth":cluster{"Y":dbl[], "Y":dbl[]}[](graph) caption="XY Graph"
  out "RingBuffer offline far":dbl[][](array[numeric])
  out "RingBuffer aerosol far":dbl[][](array[numeric])
  in  "Weather":T3(tab)=enum."Relative Humidity"
  out "Temperature (C)":dbl(graph)=22.891788766788764
  out "Pressure (mb)":dbl(graph)=837.2115384615385
  out "Relative Humdity (%)":dbl(graph)=49.224664224664224
  out "Pulse Energy (Micro Joule)":T4(graph)={"Online Pulse Energy"=4.572061428571429, "Pulse Energy Offline"=4.567985714285714}
  out "?":cluster{"mean":dbl, "mean":dbl}(graph)={"mean"=92360.0, "mean"=0.0}
  out "Index":i32=223
  out "Aerosol Smoothed":dbl[](array[numeric])=[2032.2433333333333, 3693.6266666666666, 5475.243333333334, 6900.326666666668, 8296.510000000002, 10742.943333333333, 14671.710000000001, 18866.12666666667, 22127.309999999998, 24557.376666666663, 26775.259999999995, 29101.209999999995, 31240.44333333333, 32763.793333333328, 33151.54333333332, 32357.17666666666, 30677.859999999993, 28743.57666666666, 27098.176666666666, 25379.19333333333, 23928.976666666666, 23181.326666666668, 22350.243333333332, 21216.643333333333, 20284.293333333335, 19220.793333333335, 17785.026666666665, 15202.576666666664, 11005.543333333333, 8178.760000000001, 10147.626666666667, 14726.426666666666, 16914.043333333335, 15709.06, 13460.043333333333, 11750.81, 10614.476666666666, 9687.343333333334, 8561.410000000002, 7141.4433333333345, 5839.293333333333, 5003.893333333333, 4537.71, 4204.926666666666, 3816.4266666666667, 3368.1766666666667, 2842.56, 2214.126666666666, 1634.0266666666666, 1261.71, 1120.9933333333333, 1100.1766666666667, 1134.3766666666666, 1231.0933333333332, 1351.3266666666668, 1502.2766666666666, 1723.6766666666665, 1864.0933333333332, 1678.7433333333333, 1186.0266666666666, 669.7766666666666, 326.0266666666667, 148.39333333333335, 59.21, 17.39333333333333, 0.726666666666667, -4.806666666666667, -2.6566666666666663, 1.326666666666667, -7.739999999999999, -14.323333333333332, -10.239999999999998, -9.106666666666666, -7.573333333333333, -7.039999999999999, -5.323333333333332, -3.8066666666666666, -3.1899999999999995, -6.506666666666666, -7.89, -6.64, -3.173333333333333, -1.9399999999999995, -4.973333333333333, -4.956666666666667, -7.3566666666666665, -13.09, -9.356666666666666, -2.923333333333333, -5.206666666666666, -5.673333333333333, -5.99, -1.573333333333333, -0.48999999999999955, -3.7566666666666664, -3.673333333333333, -6.123333333333333, -3.4733333333333327, -0.8066666666666662, -4.8566666666666665, -6.623333333333333, -7.106666666666666, -8.523333333333333, -6.289999999999999, -5.423333333333333, -4.49, -0.1733333333333329, -3.3399999999999994, -3.9066666666666663, -4.64, -7.39, -5.6899999999999995, -3.2899999999999996, -2.923333333333333, -4.456666666666666, -1.2899999999999996, 0.4600000000000004, 0.1433333333333337, -3.023333333333333, -1.423333333333333, -0.10666666666666624, -3.206666666666666, -4.8566666666666665, -5.823333333333333, -7.24, -5.04, -0.8233333333333329, -2.323333333333333, -2.9066666666666663, 1.5266666666666668, -1.5733333333333333, -5.023333333333333, -1.723333333333333, -1.673333333333333, -2.2233333333333327, -6.84, -5.39, -1.2399999999999995, -2.623333333333333, -2.7233333333333327, -0.1566666666666663, -0.3066666666666662, -1.8399999999999996, -1.1566666666666663, -3.3899999999999997, -2.373333333333333, -0.8399999999999996, -4.0233333333333325, -7.006666666666666, -6.373333333333333, -6.823333333333332, -6.64, -4.973333333333333, -4.073333333333333, -0.6899999999999995, -1.656666666666666, -3.573333333333333, -4.6066666666666665, -6.1899999999999995, -3.9899999999999998, 0.3600000000000003, 2.476666666666667, -0.0566666666666662, -0.6899999999999996, -0.5899999999999997, -5.573333333333333, -5.123333333333333, 0.8600000000000004, 3.443333333333334, 0.976666666666667, -1.7399999999999998, -2.573333333333333, 0.8933333333333338, 3.2100000000000004, 0.5766666666666671, 1.726666666666667, -0.273333333333333, -2.9899999999999993, -2.6899999999999995, 0.14333333333333376, 1.026666666666667, -0.9233333333333329, 0.9100000000000004, -0.10666666666666624, -1.1399999999999995, -3.2899999999999996, -1.1066666666666665, 0.5600000000000003, -0.23999999999999955, 0.9433333333333338, -2.523333333333333, -1.3066666666666662, 3.2766666666666673, 0.7100000000000004, -5.1066666666666665, -4.173333333333333, -5.0233333333333325, -9.206666666666667, -7.673333333333333, -1.6566666666666663, 0.39333333333333376, 1.5933333333333337, 0.476666666666667, -0.10666666666666647, 2.3933333333333335, 2.1600000000000006, -4.589999999999999, -6.0233333333333325, -0.17333333333333295, -0.773333333333333, -0.5399999999999996, -2.423333333333333, -0.0733333333333328, 2.0600000000000005, 0.6600000000000004, 2.5933333333333337, 1.576666666666667, -1.173333333333333, 0.0766666666666671, 1.1933333333333338, 3.66, 4.426666666666667, -0.4066666666666663, -2.756666666666666, 2.31, 2.66, -1.323333333333333, 1.2933333333333337, 0.09333333333333371, -2.2899999999999996, 0.8100000000000005, 5.343333333333334, 3.9600000000000004, 0.27666666666666706, 1.2600000000000002, 2.8433333333333337, 0.37666666666666704, -2.9066666666666663, -2.373333333333333, 1.4100000000000004, 0.9266666666666671, -2.4899999999999998, -1.673333333333333, -0.2066666666666663, -0.006666666666666293, 0.7766666666666671, 2.8600000000000003, 1.4100000000000006, -1.0899999999999996, -1.3899999999999997, 0.29333333333333367, -0.9399999999999995, 1.2100000000000004, 4.043333333333334, -0.17333333333333295, -2.4066666666666663, -2.923333333333333, -3.3566666666666665, -2.2899999999999996, -2.7566666666666664, -1.2899999999999998, 1.776666666666667, 0.626666666666667, 0.9933333333333336, 1.376666666666667, 3.9766666666666675, 6.543333333333334, 2.91, 1.4933333333333336, 1.676666666666667, 0.04333333333333371, 0.6600000000000004, 0.9933333333333337, -1.4733333333333332, -1.2399999999999998, 3.8933333333333335, 0.02666666666666684]
  out "Off-Line  Bin Readings":dbl[](array[numeric])=[1998.0, 3744.0, 5575.0, 6672.0, 7387.0, 8741.0, 13411.0, 19410.0, 24291.0, 25114.0, 25424.0, 29101.0, 33660.0, 35055.0, 34324.0, 32831.0, 31174.0, 29544.0, 28869.0, 26423.0, 25001.0, 23353.0, 21316.0, 20991.0, 20047.0, 18041.0, 16759.0, 15265.0, 12304.0, 8557.0, 9041.0, 13310.0, 18323.0, 20243.0, 18424.0, 16027.0, 13911.0, 11848.0, 9945.0, 9090.0, 7929.0, 6833.0, 6160.0, 5648.0, 5314.0, 5094.0, 4397.0, 3344.0, 2607.0, 2049.0, 1724.0, 1434.0, 1313.0, 1552.0, 1879.0, 1983.0, 1847.0, 1567.0, 1120.0, 741.0, 595.0, 522.0, 534.0, 506.0, 470.0, 460.0, 458.0, 440.0, 449.0, 432.0, 445.0, 438.0, 402.0, 441.0, 422.0, 398.0, 447.0, 420.0, 421.0, 438.0, 435.0, 433.0, 468.0, 429.0, 406.0, 409.0, 427.0, 401.0, 413.0, 440.0, 444.0, 459.0, 437.0, 441.0, 439.0, 466.0, 458.0, 408.0, 470.0, 437.0, 441.0, 466.0, 470.0, 443.0, 451.0, 430.0, 423.0, 430.0, 440.0, 465.0, 425.0, 423.0, 415.0, 380.0, 454.0, 445.0, 484.0, 468.0, 453.0, 437.0, 461.0, 457.0, 455.0, 455.0, 443.0, 443.0, 456.0, 477.0, 434.0, 475.0, 390.0, 429.0, 421.0, 428.0, 459.0, 443.0, 458.0, 404.0, 463.0, 440.0, 421.0, 453.0, 448.0, 436.0, 409.0, 419.0, 468.0, 475.0, 431.0, 479.0, 420.0, 460.0, 432.0, 408.0, 445.0, 440.0, 447.0, 483.0, 473.0, 416.0, 395.0, 454.0, 454.0, 456.0, 416.0, 466.0, 441.0, 401.0, 424.0, 443.0, 401.0, 444.0, 419.0, 449.0, 419.0, 485.0, 458.0, 468.0, 447.0, 412.0, 420.0, 416.0, 454.0, 433.0, 495.0, 437.0, 424.0, 498.0, 447.0, 443.0, 458.0, 467.0, 437.0, 460.0, 460.0, 458.0, 480.0, 427.0, 432.0, 453.0, 477.0, 413.0, 451.0, 422.0, 490.0, 440.0, 402.0, 438.0, 460.0, 471.0, 438.0, 440.0, 433.0, 461.0, 445.0, 440.0, 487.0, 475.0, 435.0, 454.0, 476.0, 447.0, 430.0, 471.0, 431.0, 443.0, 442.0, 468.0, 424.0, 452.0, 458.0, 464.0, 454.0, 420.0, 468.0, 439.0, 427.0, 452.0, 435.0, 501.0, 450.0, 442.0, 450.0, 461.0, 427.0, 454.0, 441.0, 426.0, 426.0, 451.0, 466.0, 419.0, 421.0, 472.0, 427.0, 386.0, 409.0, 430.0, 429.0, 497.0, 434.0, 432.0, 444.0, 449.0, 439.0, 440.0, 437.0, 458.0, 461.0, 491.0, 505.0, 427.0, 425.0, 424.0, 448.0, 476.0, 490.0, 478.0, 454.0]
  out "Off-Line Smoothed":dbl[](array[numeric])=[1774.0638888888886, 2759.9888888888895, 3742.380555555557, 4620.87777777778, 5481.713888888891, 6608.194444444443, 8249.824999999995, 10225.033333333327, 12141.319444444434, 14214.611111111102, 17107.011111111107, 21053.188888888886, 25479.483333333323, 29462.90277777778, 32277.230555555565, 33703.15555555556, 33768.99722222223, 32081.90277777779, 28804.75555555556, 25609.93888888888, 24150.713888888873, 23988.202777777762, 23836.286111111098, 23395.447222222218, 22714.922222222216, 21673.788888888885, 20065.147222222215, 17133.09166666666, 12905.680555555551, 10232.030555555553, 11455.022222222218, 14167.174999999996, 14892.638888888883, 13627.563888888883, 11818.41666666666, 9976.42222222222, 8209.752777777778, 6803.591666666667, 5814.583333333334, 5065.3277777777785, 4416.53888888889, 3807.0222222222237, 3239.4777777777795, 2732.694444444446, 2283.5138888888896, 1951.7444444444452, 1765.4555555555562, 1658.4694444444442, 1574.5666666666662, 1547.6249999999993, 1611.341666666666, 1731.7611111111105, 1871.3861111111105, 2031.0611111111111, 2195.636111111112, 2309.233333333334, 2327.166666666667, 2219.2666666666673, 1990.5694444444453, 1654.6944444444448, 1251.286111111111, 851.7249999999999, 521.175, 290.18055555555566, 145.77222222222224, 66.94166666666665, 26.849999999999994, 6.56388888888889, 0.7361111111111129, -3.8499999999999965, -8.108333333333327, -8.43055555555555, -7.43055555555555, -6.95833333333333, -6.872222222222222, -6.105555555555555, -6.0249999999999995, -6.58333333333333, -5.963888888888885, -4.708333333333331, -5.819444444444441, -7.202777777777774, -6.158333333333331, -6.474999999999996, -7.424999999999996, -5.638888888888887, -3.6194444444444427, -5.522222222222219, -7.830555555555549, -6.09444444444444, -4.958333333333332, -5.352777777777776, -3.463888888888887, -3.924999999999999, -5.830555555555556, -5.858333333333333, -7.81944444444444, -6.08055555555555, -3.6249999999999982, -5.027777777777775, -4.99722222222222, -5.1916666666666655, -6.802777777777775, -7.144444444444442, -5.463888888888889, -4.352777777777776, -4.374999999999998, -3.9833333333333316, -4.524999999999998, -4.994444444444442, -4.02222222222222, -3.82222222222222, -4.066666666666665, -4.47222222222222, -3.302777777777776, -2.9055555555555537, -2.7472222222222205, -1.9194444444444425, -3.830555555555554, -5.063888888888886, -3.2194444444444423, -3.9972222222222213, -5.0249999999999995, -3.9083333333333314, -3.944444444444443, -3.777777777777776, -3.9527777777777757, -4.0027777777777755, -1.6499999999999981, -2.0555555555555536, -4.166666666666664, -2.4333333333333313, -2.899999999999998, -4.894444444444442, -2.891666666666665, -2.3805555555555538, -2.2083333333333317, -2.3972222222222204, -4.033333333333331, -2.6694444444444425, -1.8083333333333313, -3.5555555555555536, -4.47222222222222, -2.627777777777776, -4.644444444444441, -6.036111111111108, -4.1388888888888875, -4.78611111111111, -3.6972222222222206, -2.024999999999998, -2.9722222222222205, -3.674999999999998, -4.055555555555554, -4.002777777777776, -2.7333333333333316, -2.477777777777776, -3.3805555555555538, -4.413888888888887, -5.077777777777776, -4.469444444444442, -2.97222222222222, -2.9527777777777757, -3.549999999999998, -2.5972222222222205, -1.7861111111111092, -3.74722222222222, -3.758333333333331, -0.6499999999999981, 0.03333333333333521, -2.858333333333331, -4.019444444444442, -3.7333333333333307, -3.5944444444444423, -2.1111111111111094, -1.7333333333333316, -1.4194444444444425, -1.6194444444444427, -2.6833333333333313, -3.7444444444444422, -0.6722222222222201, 0.8194444444444464, -3.0833333333333313, -3.213888888888887, -0.29999999999999805, -1.4083333333333314, -2.424999999999998, -0.29444444444444257, -0.12222222222222029, 0.2944444444444464, -0.6138888888888869, -3.161111111111109, -1.2666666666666648, -0.46388888888888696, -1.9361111111111091, -2.716666666666665, -3.366666666666665, -4.269444444444443, -3.627777777777776, -2.7805555555555537, -1.8944444444444424, -0.963888888888887, -1.6833333333333313, -3.713888888888888, -3.6416666666666657, -1.3083333333333313, 0.23611111111111305, -0.288888888888887, -2.0944444444444423, -2.652777777777776, -2.186111111111109, -1.824999999999998, -3.7444444444444427, -2.049999999999998, 0.8305555555555575, -0.48611111111110916, -1.0416666666666647, 0.5500000000000018, 0.23888888888889076, -0.2666666666666647, -0.5527777777777759, -0.5583333333333315, -0.688888888888887, -0.7277777777777759, -0.8083333333333315, -1.1249999999999982, -0.8722222222222203, -0.877777777777776, -1.3861111111111093, -1.5444444444444425, -0.4583333333333314, -0.6694444444444425, -0.48888888888888693, 0.7305555555555575, 0.5500000000000019, 0.8666666666666686, 1.2944444444444463, -0.20833333333333143, 0.38611111111111307, -0.33611111111110925, -1.377777777777776, -0.7361111111111093, -1.3194444444444424, -0.3083333333333314, 1.061111111111113, 1.1194444444444462, 1.1888888888888909, 2.1666666666666687, 2.8222222222222237, 0.44166666666666854, -1.1611111111111092, -0.9722222222222203, -0.3944444444444425, 1.1277777777777795, 1.0500000000000018, 0.09166666666666856, -0.06111111111110923, -0.3416666666666648, -1.7333333333333314, -1.1861111111111091, -0.7583333333333314, -0.638888888888887, -0.7249999999999981, -2.9166666666666647, -1.8055555555555538, 1.1777777777777796, 2.2527777777777795, 2.533333333333335, 1.511111111111113, 0.08611111111111303, -0.1749999999999981, -0.6722222222222203, -0.4194444444444425, 0.4722222222222241, 0.13888888888889078, 0.7472222222222241, 1.9833333333333352, 0.03611111111111298]
  out "On-Line  Smoothed":dbl[](array[numeric])=[1682.1116666666662, 2475.3311111111107, 3197.483888888889, 3771.214444444444, 4282.942222222222, 4946.675555555556, 5928.397777777777, 7076.133888888888, 8089.895, 9123.811666666668, 10651.153333333335, 12791.753333333336, 15129.006111111114, 17132.328333333335, 18370.003333333334, 18724.050555555557, 18219.17, 16595.33388888889, 14063.856111111114, 11789.956111111114, 10686.395, 10332.70888888889, 9982.222777777779, 9480.32277777778, 8886.350555555557, 8163.164444444446, 7229.356111111112, 5842.467222222222, 4121.503333333333, 3120.817222222222, 3488.4144444444446, 4299.336666666666, 4407.208888888888, 3878.317222222222, 3226.492222222222, 2612.692222222222, 2070.0172222222222, 1663.7033333333334, 1382.092222222222, 1173.5727777777777, 994.7672222222221, 833.5505555555555, 696.183888888889, 580.5727777777778, 478.0588888888889, 398.5866666666666, 354.4783333333333, 329.2894444444444, 310.2838888888889, 301.3838888888889, 312.76722222222224, 336.9338888888889, 362.97277777777776, 391.9144444444445, 419.31166666666667, 434.28944444444437, 435.81166666666655, 412.81999999999994, 364.8088888888889, 296.6672222222222, 218.2311111111111, 146.5672222222222, 88.27555555555554, 46.39500000000001, 21.08666666666667, 6.6144444444444455, 0.04222222222222266, -1.5633333333333328, -3.9383333333333326, -4.774444444444444, -4.310555555555555, -3.0188888888888883, -4.8633333333333315, -5.171666666666665, -4.038333333333332, -4.477222222222221, -3.977222222222222, -4.432777777777778, -2.2494444444444444, -3.588333333333329, -5.402222222222218, -4.30222222222222, -4.816111111111109, -4.724444444444444, -4.699444444444444, -5.516111111111112, -4.416111111111112, -1.3855555555555554, -1.860555555555555, -3.1799999999999997, -4.655000000000001, -5.385555555555556, -3.1438888888888883, -3.0522222222222215, -3.9161111111111104, -2.799444444444444, -2.9688888888888885, -2.1827777777777775, -1.9577777777777774, -4.663333333333332, -4.191111111111109, -2.874444444444444, -3.3216666666666663, -3.7077777777777774, -3.8549999999999995, -3.2188888888888885, -3.7688888888888883, -4.366111111111111, -4.58, -3.7466666666666666, -1.1272222222222221, -0.4577777777777773, -2.1299999999999994, -2.829999999999999, -2.913333333333333, -4.560555555555554, -3.9244444444444437, -2.255, -3.399444444444444, -4.193888888888888, -4.777222222222221, -3.1133333333333333, -2.902222222222222, -2.3216666666666663, -0.49111111111111067, -1.7299999999999995, -2.9577777777777774, -4.538333333333332, -3.518888888888888, -0.11888888888888849, -0.5994444444444441, -3.166111111111111, -3.682777777777777, -4.252222222222222, -3.4299999999999997, -3.357777777777777, -3.871666666666666, -1.6688888888888886, -2.2105555555555547, -5.066111111111111, -5.196666666666665, -3.5411111111111104, -2.8438888888888885, -4.007777777777777, -2.5799999999999996, -2.6216666666666666, -3.3605555555555555, -2.924444444444444, -3.4772222222222218, -2.7522222222222217, -2.64111111111111, -2.993888888888888, -2.2799999999999994, -2.6855555555555553, -2.796666666666667, -3.1966666666666663, -2.963333333333333, -0.1633333333333329, -0.007777777777777328, -0.974444444444444, -0.6716666666666663, -0.7549999999999996, -2.2688888888888887, -4.235555555555555, -5.085555555555555, -4.113333333333332, -0.4077777777777776, 0.5172222222222225, -2.024444444444444, -1.9716666666666662, -0.5355555555555551, -0.6161111111111107, 0.5311111111111114, 2.556111111111112, 0.46166666666666734, -2.3883333333333328, -3.0133333333333328, -3.6022222222222218, -2.6077777777777778, -1.2466666666666661, -1.9938888888888884, -2.110555555555555, -1.4299999999999995, -1.4827777777777773, -2.1855555555555553, -1.9716666666666662, -2.3661111111111106, -3.3411111111111107, -3.505, -2.0911111111111107, -0.1272222222222218, -0.2855555555555551, -0.2716666666666662, 0.6838888888888894, 0.6922222222222227, -1.391111111111111, -0.1438888888888885, 1.0422222222222228, -1.2966666666666662, -1.0327777777777774, -0.25499999999999956, -0.17999999999999955, 0.5088888888888894, -0.1799999999999995, -1.1716666666666662, -2.032777777777777, -2.774444444444444, -3.5605555555555553, -3.288333333333333, -0.5827777777777773, -1.3077777777777775, -2.038333333333333, -0.8799999999999997, -0.4299999999999996, 0.5894444444444449, -0.9577777777777772, -2.7994444444444437, -1.5133333333333328, -0.8077777777777773, 0.400555555555556, -0.9883333333333331, -2.4355555555555553, -2.271666666666666, -4.4272222222222215, -4.407777777777778, -3.474444444444444, -2.507777777777777, -1.1633333333333329, -1.2716666666666663, -1.274444444444444, -0.16888888888888848, -1.635555555555555, -2.121666666666666, -0.31888888888888844, -1.3855555555555552, -1.5799999999999996, -2.132777777777777, -2.7938888888888886, -1.4688888888888885, -0.9911111111111107, -2.3077777777777775, -2.8438888888888885, -1.5244444444444438, -0.8855555555555552, -1.285555555555555, -1.9799999999999993, -1.6216666666666661, -0.06888888888888844, -0.6272222222222218, -2.474444444444444, -1.9438888888888886, -1.135555555555555, -1.235555555555555, -1.1911111111111108, 1.0200000000000005, 0.7922222222222226, -0.5855555555555554, 0.7200000000000004, -0.34666666666666623, -0.7688888888888885, 0.8227777777777782, 0.5727777777777782, 1.2755555555555562, 1.1477777777777785, -0.8605555555555551, -0.6911111111111106, -0.06888888888888844, 1.4311111111111117, 2.378333333333334, 1.075555555555556, -1.3605555555555549, -2.7411111111111106, -0.29944444444444396, 1.9783333333333337, -0.3911111111111105, -1.107777777777777, 0.5894444444444449]
  out "On-Line Bin Readings":dbl[](array[numeric])=[2055.0, 3379.0, 4978.0, 5667.0, 6154.0, 6843.0, 9602.0, 13217.0, 15478.0, 15468.0, 16495.0, 18458.0, 19963.0, 20115.0, 19570.0, 17992.0, 16507.0, 15054.0, 13926.0, 12004.0, 11142.0, 10025.0, 8666.0, 7984.0, 7294.0, 6482.0, 6162.0, 5658.0, 4477.0, 2881.0, 2735.0, 4049.0, 5541.0, 6238.0, 5396.0, 4639.0, 3941.0, 3129.0, 2750.0, 2443.0, 2187.0, 1797.0, 1646.0, 1492.0, 1512.0, 1383.0, 1301.0, 1053.0, 974.0, 740.0, 648.0, 599.0, 597.0, 650.0, 724.0, 692.0, 649.0, 645.0, 569.0, 458.0, 441.0, 438.0, 433.0, 446.0, 411.0, 432.0, 431.0, 430.0, 404.0, 395.0, 417.0, 426.0, 415.0, 418.0, 442.0, 398.0, 434.0, 424.0, 447.0, 432.0, 417.0, 397.0, 392.0, 414.0, 446.0, 424.0, 401.0, 400.0, 398.0, 428.0, 433.0, 405.0, 436.0, 429.0, 411.0, 407.0, 423.0, 416.0, 437.0, 408.0, 443.0, 423.0, 431.0, 446.0, 429.0, 404.0, 461.0, 458.0, 426.0, 452.0, 426.0, 405.0, 419.0, 463.0, 449.0, 483.0, 422.0, 456.0, 419.0, 420.0, 385.0, 416.0, 418.0, 403.0, 454.0, 443.0, 437.0, 403.0, 434.0, 468.0, 465.0, 414.0, 414.0, 429.0, 439.0, 397.0, 445.0, 443.0, 416.0, 420.0, 434.0, 440.0, 453.0, 442.0, 416.0, 420.0, 393.0, 422.0, 434.0, 442.0, 392.0, 402.0, 422.0, 455.0, 434.0, 448.0, 451.0, 454.0, 436.0, 417.0, 391.0, 388.0, 424.0, 447.0, 412.0, 408.0, 395.0, 416.0, 423.0, 428.0, 436.0, 434.0, 416.0, 414.0, 425.0, 409.0, 433.0, 480.0, 454.0, 418.0, 418.0, 443.0, 404.0, 419.0, 415.0, 428.0, 473.0, 417.0, 429.0, 426.0, 385.0, 440.0, 401.0, 437.0, 451.0, 455.0, 440.0, 436.0, 413.0, 464.0, 439.0, 438.0, 453.0, 444.0, 445.0, 459.0, 402.0, 431.0, 427.0, 433.0, 420.0, 433.0, 436.0, 412.0, 394.0, 427.0, 433.0, 423.0, 418.0, 414.0, 465.0, 450.0, 399.0, 394.0, 439.0, 423.0, 426.0, 446.0, 451.0, 372.0, 420.0, 418.0, 437.0, 416.0, 481.0, 418.0, 447.0, 421.0, 459.0, 418.0, 389.0, 425.0, 436.0, 384.0, 453.0, 455.0, 431.0, 429.0, 402.0, 407.0, 421.0, 432.0, 434.0, 431.0, 416.0, 452.0, 431.0, 423.0, 465.0, 435.0, 445.0, 437.0, 427.0, 438.0, 419.0, 440.0, 421.0, 460.0, 436.0, 434.0, 427.0, 425.0, 458.0, 400.0, 416.0, 424.0, 400.0, 420.0, 411.0]
  out "Range Corrected Altitude Array":dbl[](array[numeric])=[5625.0, 22500.0, 50625.0, 90000.0, 140625.0, 202500.0, 275625.0, 360000.0, 455625.0, 562500.0, 680625.0, 810000.0, 950625.0, 1102500.0, 1265625.0, 1440000.0, 1625625.0, 1822500.0, 2030625.0, 2250000.0, 2480625.0, 2722500.0, 2975625.0, 3240000.0, 3515625.0, 3802500.0, 4100625.0, 4410000.0, 4730625.0, 5062500.0, 5405625.0, 5760000.0, 6125625.0, 6502500.0, 6890625.0, 7290000.0, 7700625.0, 8122500.0, 8555625.0, 9000000.0, 9455625.0, 9922500.0, 10400625.0, 10890000.0, 11390625.0, 11902500.0, 12425625.0, 12960000.0, 13505625.0, 14062500.0, 14630625.0, 15210000.0, 15800625.0, 16402500.0, 17015625.0, 17640000.0, 18275625.0, 18922500.0, 19580625.0, 20250000.0, 20930625.0, 21622500.0, 22325625.0, 23040000.0, 23765625.0, 24502500.0, 25250625.0, 26010000.0, 26780625.0, 27562500.0, 28355625.0, 29160000.0, 29975625.0, 30802500.0, 31640625.0, 32490000.0, 33350625.0, 34222500.0, 35105625.0, 36000000.0, 36905625.0, 37822500.0, 38750625.0, 39690000.0, 40640625.0, 41602500.0, 42575625.0, 43560000.0, 44555625.0, 45562500.0, 46580625.0, 47610000.0, 48650625.0, 49702500.0, 50765625.0, 51840000.0, 52925625.0, 54022500.0, 55130625.0, 56250000.0, 57380625.0, 58522500.0, 59675625.0, 60840000.0, 62015625.0, 63202500.0, 64400625.0, 65610000.0, 66830625.0, 68062500.0, 69305625.0, 70560000.0, 71825625.0, 73102500.0, 74390625.0, 75690000.0, 77000625.0, 78322500.0, 79655625.0, 81000000.0, 82355625.0, 83722500.0, 85100625.0, 86490000.0, 87890625.0, 89302500.0, 90725625.0, 92160000.0, 93605625.0, 95062500.0, 96530625.0, 98010000.0, 99500625.0, 101002500.0, 102515625.0, 104040000.0, 105575625.0, 107122500.0, 108680625.0, 110250000.0, 111830625.0, 113422500.0, 115025625.0, 116640000.0, 118265625.0, 119902500.0, 121550625.0, 123210000.0, 124880625.0, 126562500.0, 128255625.0, 129960000.0, 131675625.0, 133402500.0, 135140625.0, 136890000.0, 138650625.0, 140422500.0, 142205625.0, 144000000.0, 145805625.0, 147622500.0, 149450625.0, 151290000.0, 153140625.0, 155002500.0, 156875625.0, 158760000.0, 160655625.0, 162562500.0, 164480625.0, 166410000.0, 168350625.0, 170302500.0, 172265625.0, 174240000.0, 176225625.0, 178222500.0, 180230625.0, 182250000.0, 184280625.0, 186322500.0, 188375625.0, 190440000.0, 192515625.0, 194602500.0, 196700625.0, 198810000.0, 200930625.0, 203062500.0, 205205625.0, 207360000.0, 209525625.0, 211702500.0, 213890625.0, 216090000.0, 218300625.0, 220522500.0, 222755625.0, 225000000.0, 227255625.0, 229522500.0, 231800625.0, 234090000.0, 236390625.0, 238702500.0, 241025625.0, 243360000.0, 245705625.0, 248062500.0, 250430625.0, 252810000.0, 255200625.0, 257602500.0, 260015625.0, 262440000.0, 264875625.0, 267322500.0, 269780625.0, 272250000.0, 274730625.0, 277222500.0, 279725625.0, 282240000.0, 284765625.0, 287302500.0, 289850625.0, 292410000.0, 294980625.0, 297562500.0, 300155625.0, 302760000.0, 305375625.0, 308002500.0, 310640625.0, 313290000.0, 315950625.0, 318622500.0, 321305625.0, 324000000.0, 326705625.0, 329422500.0, 332150625.0, 334890000.0, 337640625.0, 340402500.0, 343175625.0, 345960000.0, 348755625.0, 351562500.0, 354380625.0, 357210000.0, 360050625.0, 362902500.0, 365765625.0, 368640000.0, 371525625.0, 374422500.0, 377330625.0, 380250000.0, 383180625.0, 386122500.0, 389075625.0, 392040000.0, 395015625.0, 398002500.0, 401000625.0, 404010000.0, 407030625.0, 410062500.0, 413105625.0, 416160000.0, 419225625.0, 422302500.0, 425390625.0, 428490000.0, 431600625.0, 434722500.0, 437855625.0, 441000000.0]
  out "Altitude Array (km)":dbl[](array[numeric])=[0.075, 0.15, 0.22499999999999998, 0.3, 0.375, 0.45, 0.5249999999999999, 0.6, 0.6749999999999999, 0.7499999999999999, 0.825, 0.8999999999999999, 0.9749999999999999, 1.05, 1.125, 1.2, 1.275, 1.3499999999999999, 1.4249999999999998, 1.5, 1.575, 1.65, 1.7249999999999999, 1.7999999999999998, 1.8749999999999998, 1.95, 2.025, 2.1, 2.1750000000000003, 2.25, 2.325, 2.4, 2.475, 2.5500000000000003, 2.625, 2.7, 2.775, 2.85, 2.9250000000000003, 3.0, 3.075, 3.15, 3.225, 3.3000000000000003, 3.375, 3.45, 3.525, 3.6, 3.675, 3.75, 3.825, 3.9, 3.975, 4.05, 4.125, 4.2, 4.275, 4.35, 4.425, 4.5, 4.575, 4.65, 4.725, 4.8, 4.875, 4.95, 5.025, 5.1, 5.175, 5.25, 5.325, 5.4, 5.475, 5.55, 5.625, 5.7, 5.775, 5.85, 5.925, 6.0, 6.075, 6.15, 6.225, 6.3, 6.375, 6.45, 6.525, 6.6, 6.675, 6.75, 6.825, 6.9, 6.975, 7.05, 7.125, 7.2, 7.2749999999999995, 7.35, 7.425, 7.5, 7.575, 7.6499999999999995, 7.725, 7.8, 7.875, 7.95, 8.024999999999999, 8.1, 8.174999999999999, 8.249999999999998, 8.325, 8.399999999999999, 8.475, 8.549999999999999, 8.624999999999998, 8.7, 8.774999999999999, 8.85, 8.924999999999999, 8.999999999999998, 9.075, 9.149999999999999, 9.225, 9.299999999999999, 9.374999999999998, 9.45, 9.524999999999999, 9.6, 9.674999999999999, 9.749999999999998, 9.825, 9.899999999999999, 9.975, 10.049999999999999, 10.124999999999998, 10.2, 10.274999999999999, 10.35, 10.424999999999999, 10.499999999999998, 10.575, 10.649999999999999, 10.725, 10.799999999999999, 10.874999999999998, 10.95, 11.024999999999999, 11.1, 11.174999999999999, 11.249999999999998, 11.325, 11.399999999999999, 11.475, 11.549999999999999, 11.624999999999998, 11.7, 11.774999999999999, 11.85, 11.924999999999999, 11.999999999999998, 12.075, 12.149999999999999, 12.225, 12.299999999999999, 12.374999999999998, 12.45, 12.524999999999999, 12.6, 12.674999999999999, 12.749999999999998, 12.825, 12.899999999999999, 12.975, 13.049999999999999, 13.124999999999998, 13.2, 13.274999999999999, 13.35, 13.424999999999999, 13.499999999999998, 13.575, 13.649999999999999, 13.725, 13.799999999999999, 13.874999999999998, 13.95, 14.024999999999999, 14.1, 14.174999999999999, 14.249999999999998, 14.325, 14.399999999999999, 14.474999999999998, 14.549999999999999, 14.624999999999998, 14.7, 14.774999999999999, 14.849999999999998, 14.924999999999999, 14.999999999999998, 15.075, 15.149999999999999, 15.224999999999998, 15.299999999999999, 15.374999999999998, 15.45, 15.524999999999999, 15.599999999999998, 15.674999999999999, 15.749999999999998, 15.825, 15.899999999999999, 15.974999999999998, 16.05, 16.125, 16.2, 16.275, 16.349999999999998, 16.424999999999997, 16.5, 16.575, 16.65, 16.724999999999998, 16.799999999999997, 16.875, 16.95, 17.025, 17.099999999999998, 17.174999999999997, 17.25, 17.325, 17.4, 17.474999999999998, 17.549999999999997, 17.625, 17.7, 17.775, 17.849999999999998, 17.924999999999997, 18.0, 18.075, 18.15, 18.224999999999998, 18.299999999999997, 18.375, 18.45, 18.525, 18.599999999999998, 18.674999999999997, 18.75, 18.825, 18.9, 18.974999999999998, 19.049999999999997, 19.125, 19.2, 19.275, 19.349999999999998, 19.424999999999997, 19.5, 19.575, 19.65, 19.724999999999998, 19.799999999999997, 19.875, 19.95, 20.025, 20.099999999999998, 20.174999999999997, 20.25, 20.325, 20.4, 20.474999999999998, 20.549999999999997, 20.625, 20.7, 20.775, 20.849999999999998, 20.924999999999997, 21.0]
  out "Offline Pulse Energy":dbl=4.587235714285714
  out "Online Pulse Energy":dbl=4.572061428571429
  in  "Instrument Control":T5(tab)=enum."Wavemeter"
  in  "ILX Address On":dbl=1.0 min=0.0 step=1.0
  in  "ILX Address Off":dbl=2.0 min=0.0 step=1.0
  in  "OnLineLD":dbl=169.7
  in  "OffLineLD":dbl=172.62
  in  "Pulse B Polarity":enum32{"Low", "High"}(ring)=enum."High"
  in  "Pulse A Delay(ns)":u32=1040 min=80 max=327600
  in  "Pulse B Delay(ns)":u32=170000 min=80 max=327600 step=1
  in  "Accumulation Delay(ns)":u32=10 min=10 max=1270 step=1
  in  "Sync Pulse Polarity":enum32{"Low", "High"}(ring)=enum."High"
  in  "Pulse A Polarity":enum32{"Low", "High"}(ring)=enum."High"
  in  "Number of Bins":u32=280 min=2 max=4095 step=1
  in  "Number of Accumulates":u32=10000 min=1 max=32767 step=1
  in  "Time Resolution Per Bin(ns)":u32=500 min=5 max=1063 step=1
  out "AMCS_Profile":i32=69514
  in  "Lambda On Set (nm)":dbl=828.198 format="%.5f"
  out "Lambda On Read (nm)":dbl=828.197984591025 format="%.5f"
  out "Lambda Off Read (nm)":dbl=828.2976619556888 format="%.5f"
  in  "Lambda Off Set (nm)":dbl=828.29765 format="%#.5f"
  in  "Bristol In":i32=5
  out "Bristol Out":i32
  out "WL_Difference":dbl=-1.5408974945785303e-05 format="%#_3e"
  out "WL Difference off":dbl=1.1955688819398347e-05 format="%#_3e"
  out "Wavelength Lock Online":bool=TRUE
  out "Wavelength Lock Offline":bool=TRUE
  in  "calculate absorption cross sections":bool
  in  "Online_Tol":dbl=5e-05 format="%#_15g"
  in  "Cancel online":bool
  in  "Offline_Tol":dbl=5e-05 format="%#_15g"
  in  "Cancel Offline":bool
  in  "Smoothing Range":dbl=150.0
  in  "Total DIAL Integration Time (Minutes)":i32=3
  in  "Data Reads (number of loops)":i32=1
  in  "Total Aerosol Integration Time (Minutes)":dbl=0.5
  in  "Scalar Wait Time":u32
  out "Smoothed Bins":dbl=2.0
  in  "NewportIn":string
  in  "logging":bool
  out "Newport Device Key":string="1918-R 15120"
  in  "SampleSize":i32=2
  out "NewportRef":refnum<k24>
  in  "Switch Comm Port":refnum<visa-resource-name>="COM3"
  out "FF_On_Ref":refnum<file>
  out "FF_On_Ptr":i64=1228656 format="%.2p"
  out "FF_Off_Ref":refnum<file>
  out "FF_Off_Ptr":i64=1228656 format="%.2p"
  out "NF_On_Ref":refnum<file>
  out "NF_On_Ptr":i64=1228656 format="%.2p"
  out "NF_Off_Ref":refnum<file>
  out "NF_Off_Ptr":i64=1228656 format="%.2p"
  out "DataOpen":bool=TRUE
  out "File Path_Far Field (out)":string="C:\\Users\\H2ODial\\Desktop\\SharedTeleWVData\\160819FF\\20"
  out "File Path_Near Field (out)":string="C:\\Users\\H2ODial\\Desktop\\SharedTeleWVData\\160819NF\\20"
  in  "Data File DIR (in)":string="C:\\Users\\H2ODial\\Desktop\\SharedTeleWVData\\"
  out "TRHP":T6={"Temp C"=22.891788766788764, "RelH %"=49.224664224664224, "Press hPa"=837.2115384615385, "AbH g/m^3"=10.11904761904762}
  in  "WS visa":refnum<visa-resource-name>="LuftWS"
  in  "WS_On/Off":bool=TRUE
  in  "bins":u32=280 min=2 max=4095 step=1
  out "y offset":u32=10
  in  "ns scale":u32=500
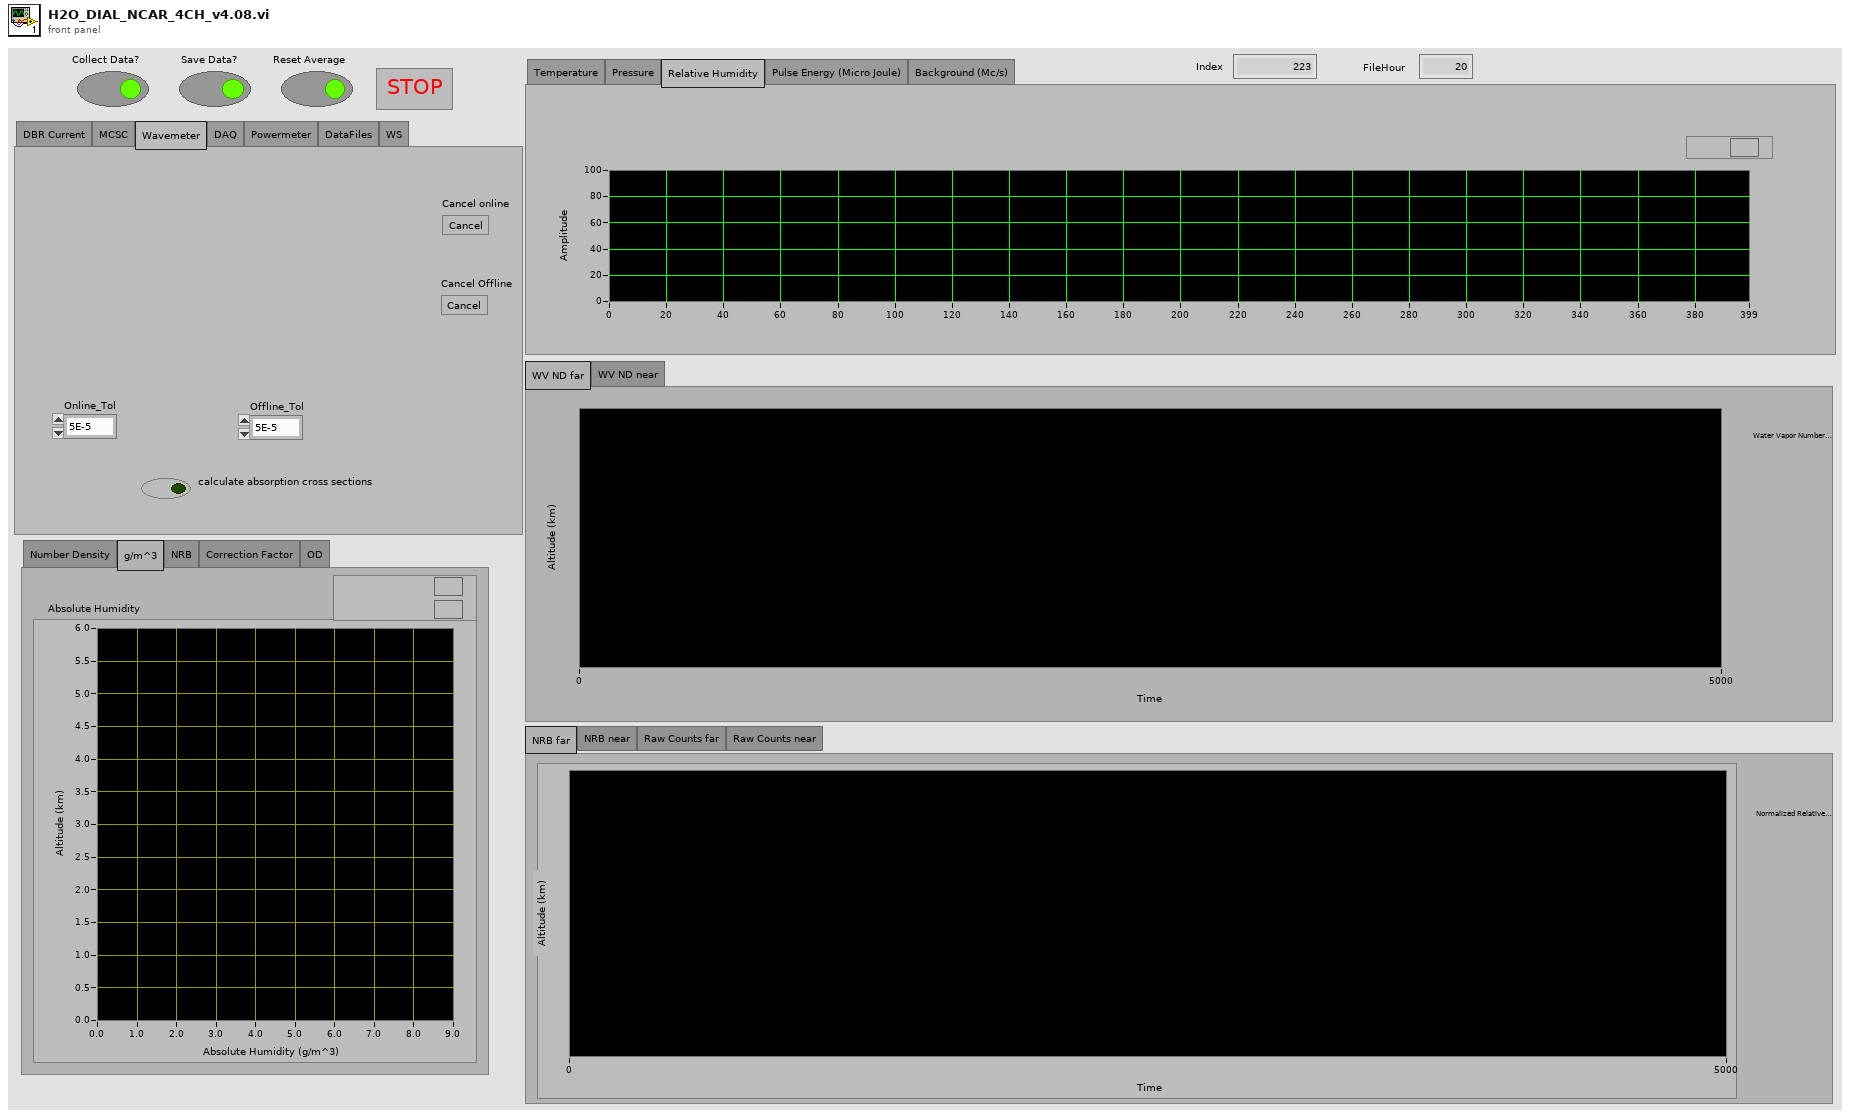
[diagram p1: front panel]
types:
  T1 = enum32{"NRB far", "NRB near", "Raw Counts far", "Raw Counts near"}
  T2 = enum32{"Number Density", "g/m^3", "NRB", "Correction Factor", "OD"}
  T3 = enum32{"Temperature", "Pressure", "Relative Humidity", "Pulse Energy (Micro Joule)", "Background (Mc/s)"}
  T4 = cluster{"Online Pulse Energy":dbl, "Pulse Energy Offline":dbl}
  T5 = enum32{"DBR Current", "MCSC", "Wavemeter", "DAQ", "Powermeter", "DataFiles", "WS"}
  T6 = cluster{"Temp C":dbl, "RelH %":dbl, "Press hPa":dbl, "AbH g/m^3":dbl}
  T7 = enum16{"Initialize ILX", "Set ON T", "Set Off T", "Set ON I", "Set Off I", "Set On Lim", "Set Off Lim", "Read ILX", "TEC ON/OFF", "LASER ON/OFF", "Status?", "ILX OFF"}
  T8 = enum16{"open", "replace", "create", "open or create", "replace or create", "replace or create with confirmation"}
  T9 = cluster{"Temp":dbl, "RelH":dbl, "Press":dbl, "AbH":dbl}
  T10 = typedef "LVDateTimeRec.ctl" = cluster{"fractional second":dbl, "second":i32, "minute":i32, "hour":i32, "day of month":i32, "month":i32, "year":i32, "day of week":i32, "day of year":i32, "DST":i32}
  T11 = cluster{"Online Pulse Energy":dbl, "Offline Pulse Energy":dbl}
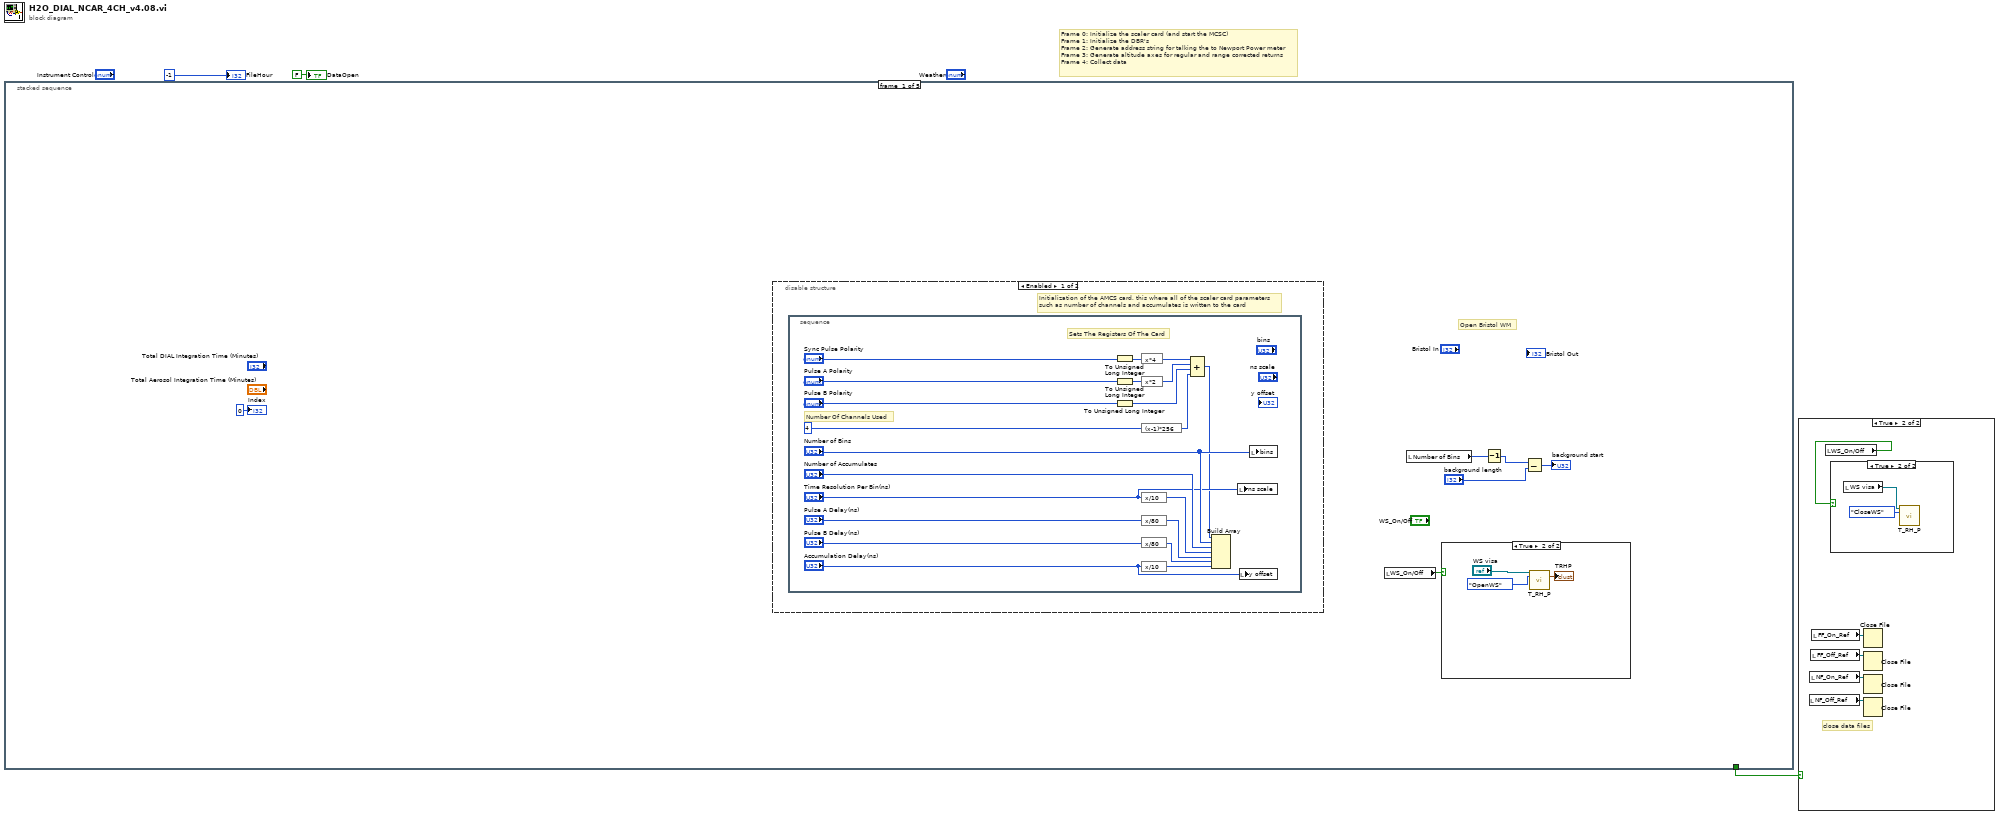
[diagram p0: block diagram]
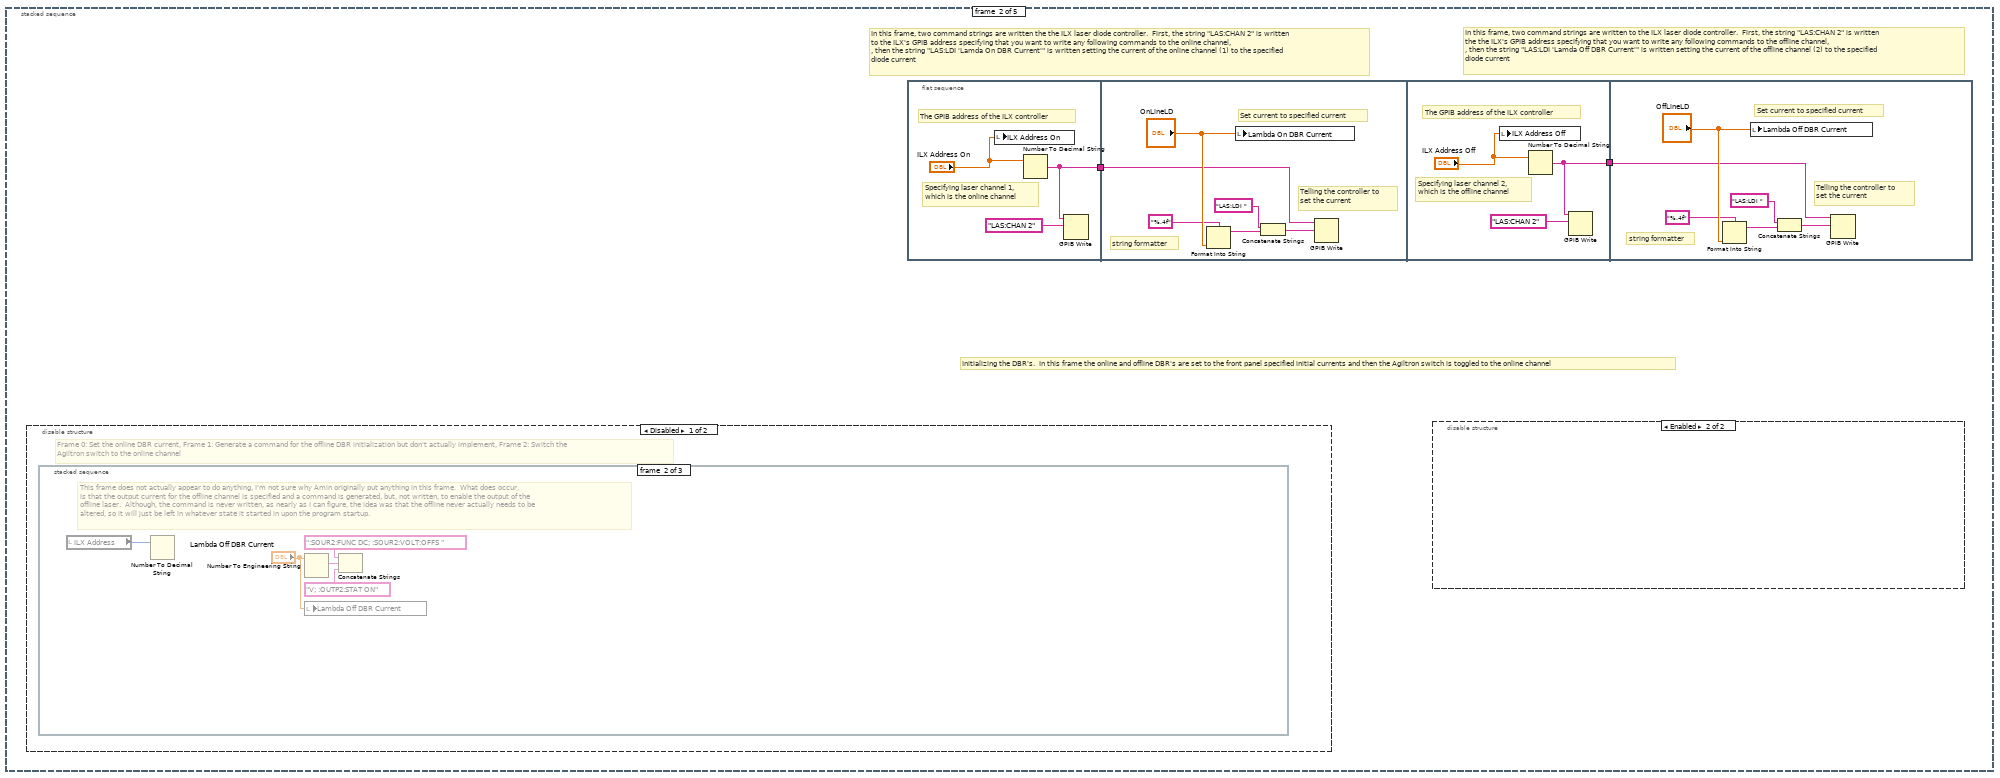
[diagram p6: hidden frame]
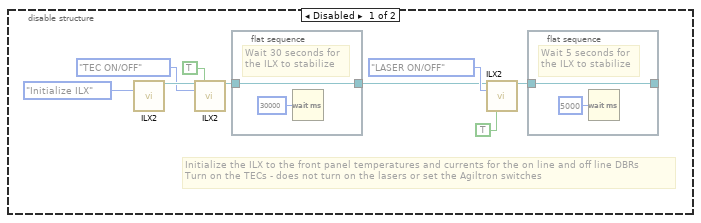
[diagram p7: hidden frame]
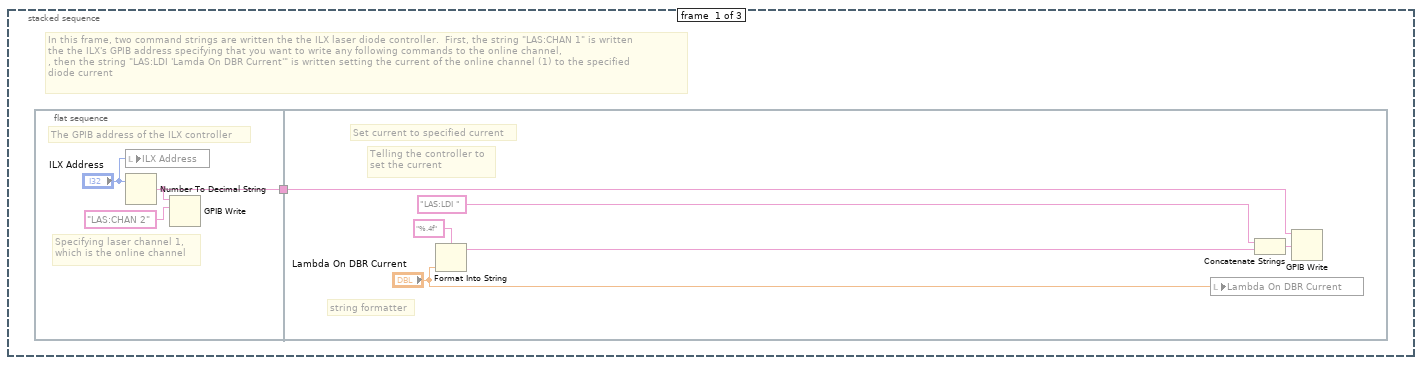
[diagram p8: hidden frame]
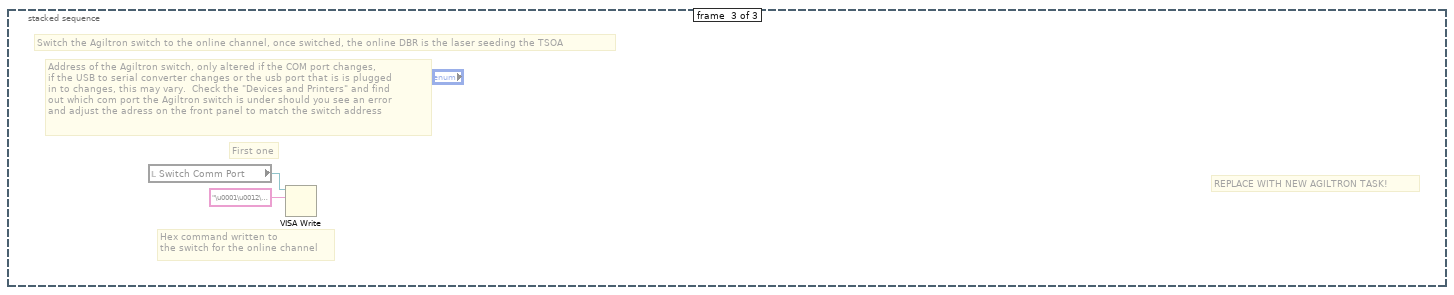
[diagram p9: hidden frame]
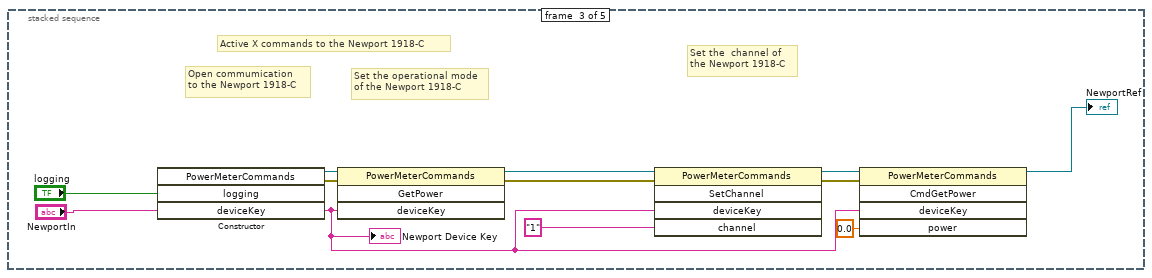
[diagram p11: hidden frame]
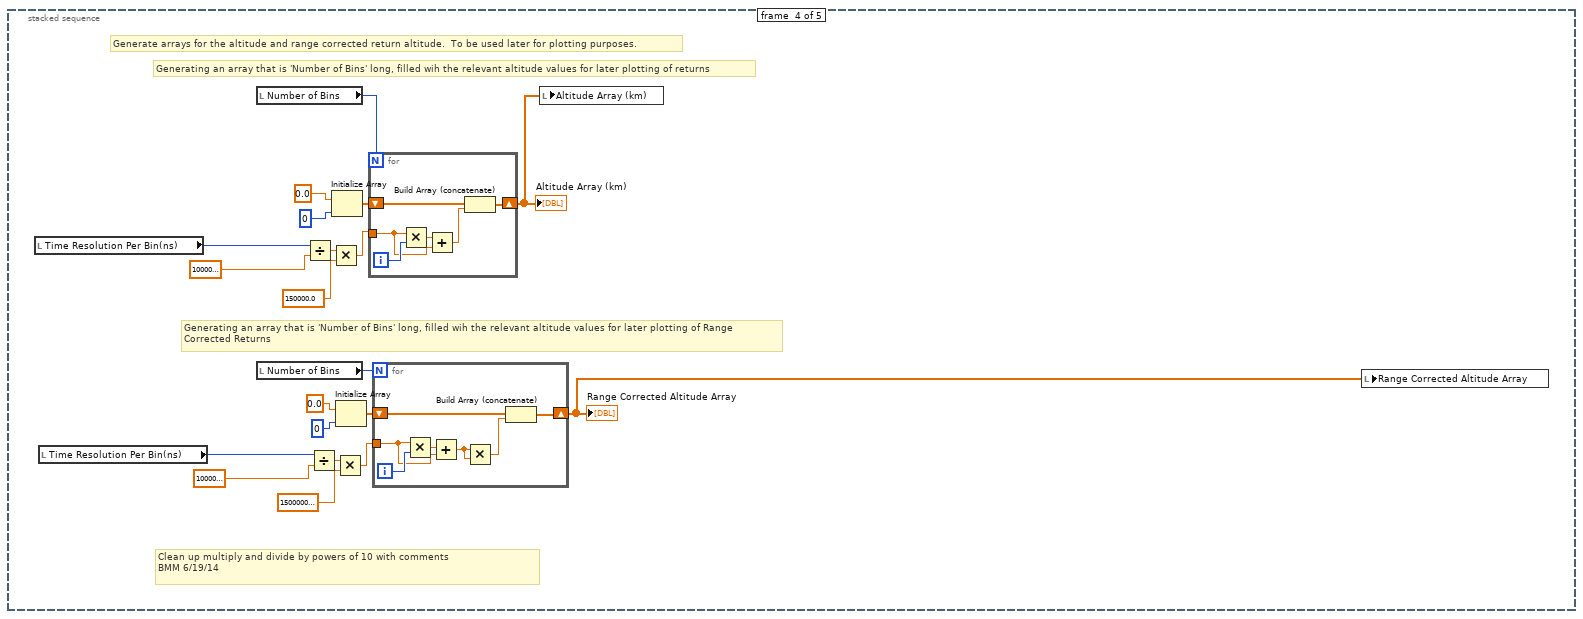
[diagram p12: hidden frame]
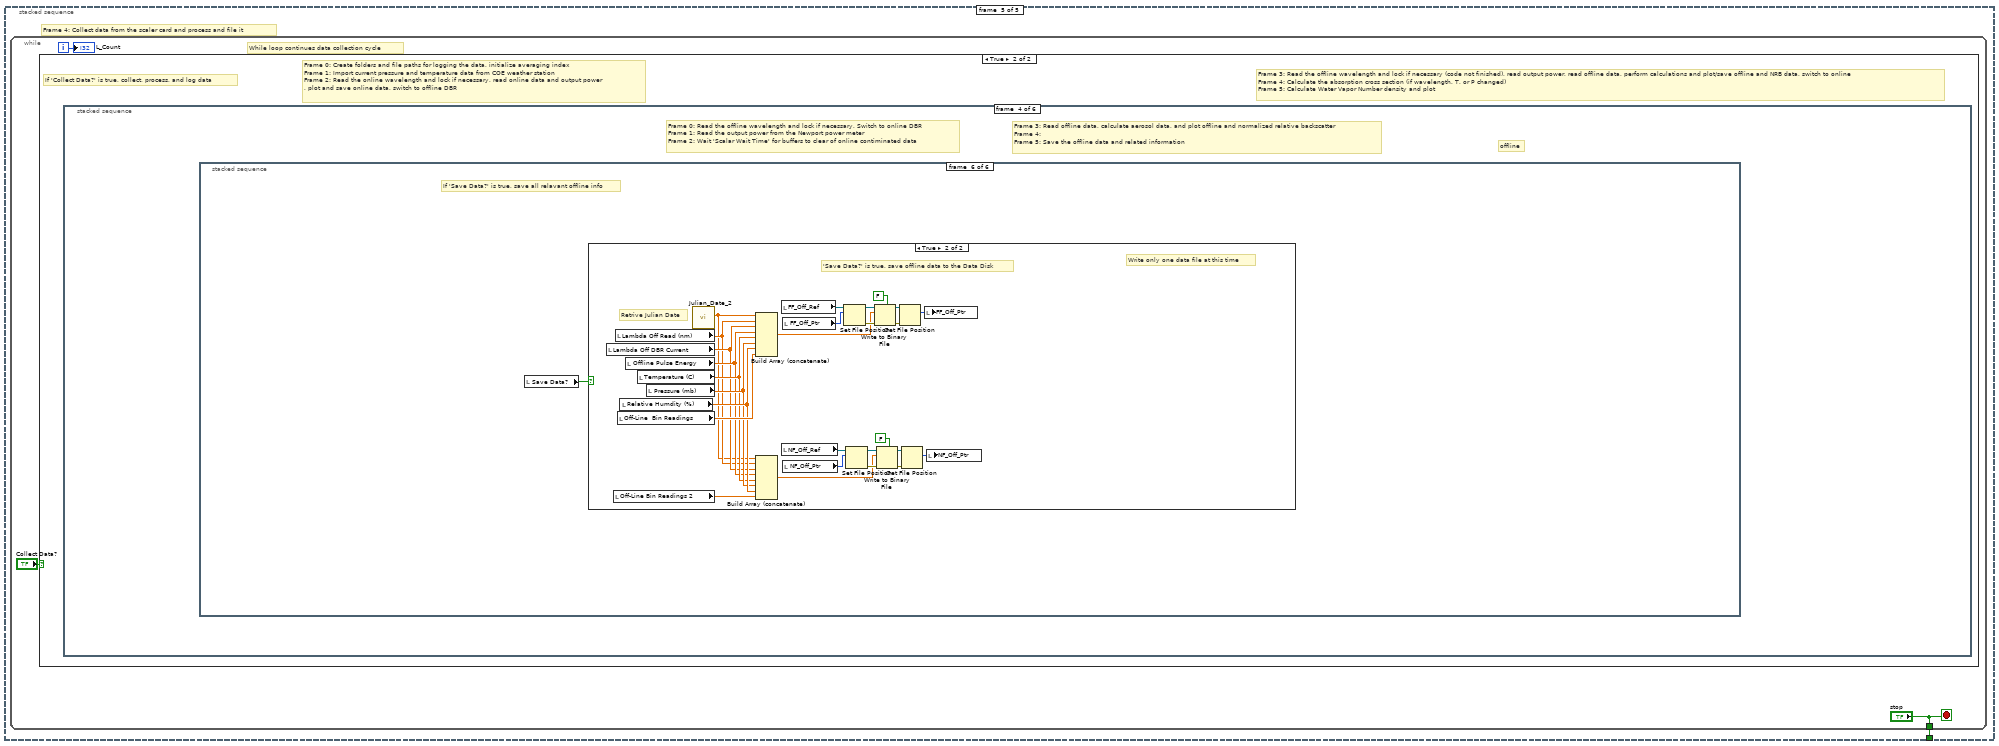
[diagram p13: hidden frame]
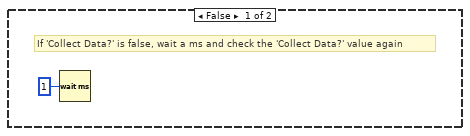
[diagram p14: hidden frame]
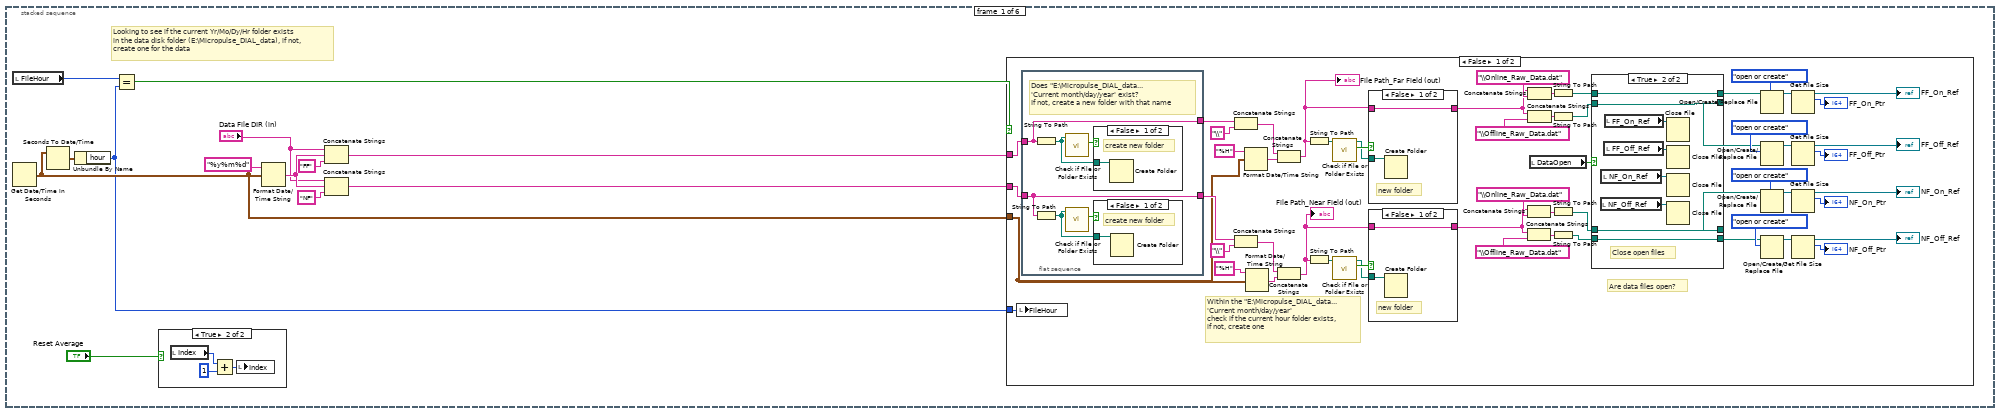
[diagram p15: hidden frame]
diagram:
  # "Frame 0: Initialize the scaler card (and start the MCSC)\nFrame 1: Initialize the DBR's\nFrame 2: Generate address string for talking the to Newport Power meter\nFrame 3: Generate altitude axes for regular and range corrected returns\nFrame 4: Collect data"
  n1 = stacked-sequence {
    tunnel: [_ _ _ _ w129] -> w3
    frame #0 {
      # "Open Bristol WM"
      n2 = disable-structure shown="Enabled" {
        frame Enabled {
          # "Initialization of the AMCS card, this where all of the scaler card parameters\nsuch as number of channels and accumulates is written to the card"
          n3 = stacked-sequence {
            frame #0 {
              # "Sets The Registers Of The Card"
              # "Number Of Channels Used"
              n4 = To Unsigned Long Integer(number="Sync Pulse Polarity") -> (unsigned 32bit integer=w13:u32)
              n5 = To Unsigned Long Integer(number="Pulse A Polarity") -> (unsigned 32bit integer=w17:u32)
              n6 = To Unsigned Long Integer(number="Pulse B Polarity") -> (unsigned 32bit integer=w15:u32)
              n7 = expression code="x*4"(w13) -> (w22:u32)
              n8 = expression code="x*2"(w17) -> (w21:u32)
              n9 = expression code="(x-1)*256"(u32 4 ("Number of Channels Used")) -> (w20:u32)
              n10 = expression code="x/10"("Time Resolution Per Bin(ns)") -> (w24:u32)
              n11 = expression code="x/80"("Pulse A Delay(ns)") -> (w31:u32)
              n12 = expression code="x/80"("Pulse B Delay(ns)") -> (w33:u32)
              n13 = expression code="x/10"("Accumulation Delay(ns)") -> (w32:u32)
              n14 = Compound Arithmetic op=ADD(w22, w21, w15, w20) -> (w19:u32)
              n15 = Build Array(w19, "Number of Bins", "Number of Accumulates", w24, w31, w33, w32) -> ()  [unwired: 1 out]
              n16 = local write "ns scale"("Time Resolution Per Bin(ns)") -> ()
              n17 = local write "y offset"("Accumulation Delay(ns)") -> ()
              n18 = local write "bins"("Number of Bins") -> ()
            }
          }
        }
        frame Disabled {
        }
      }
      n19 = local read "WS_On/Off"() -> (w4:bool)
      n20 = local read "Number of Bins"() -> (w8:u32)
      n21 = case shown="True" w4 {
        frame False {
        }
        frame True {
          n22 = call "T_RH_P.vi"("VISA in"="WS visa", "WS_Commands"=enum16{"OpenWS", "ReadTRHP", "CloseWS"}."OpenWS") -> ("TRHP"=→"TRHP":T9)  [unwired: 11 in, 2 out]
        }
      }
      n23 = Decrement(x=w8) -> (x-1=w7:u32)
      n24 = Subtract(x=w7, y="background length") -> (x-y=→"background start":u32)
      "Index" <- 0 ("Index")
    }
    frame #1 {
      # "In this frame, two command strings are written to the ILX laser diode controller.  First, the string \"LAS:CHAN 2\" is written\nthe the ILX's GPIB address specifying that you want to write any following commands to the offline channel,\n, then the string \"LAS:LDI 'Lamda Off DBR Current'\" is written setting the current of the offline channel (2) to the specified \ndiode current"
      # "In this frame, two command strings are written the the ILX laser diode controller.  First, the string \"LAS:CHAN 2\" is written\nto the ILX's GPIB address specifying that you want to write any following commands to the online channel,\n, then the string \"LAS:LDI 'Lamda On DBR Current'\" is written setting the current of the online channel (1) to the specified \ndiode current"
      # "Initializing the DBR's.  In this frame the online and offline DBR's are set to the front panel specified initial currents and then the Agiltron switch is toggled to the online channel"
      n25 = disable-structure shown="Disabled" {
        frame Disabled {
          # "Frame 0: Set the online DBR current, Frame 1: Generate a command for the offline DBR initialization but don't actually implement, Frame 2: Switch the \nAgiltron switch to the online channel"
          n26 = stacked-sequence {
            frame #0 {
              # "In this frame, two command strings are written the the ILX laser diode controller.  First, the string \"LAS:CHAN 1\" is written\nthe the ILX's GPIB address specifying that you want to write any following commands to the online channel,\n, then the string \"LAS:LDI 'Lamda On DBR Current'\" is written setting the current of the online channel (1) to the specified \ndiode current"
              n27 = flat-sequence {
                tunnel: [w69] -> w67
                tunnel: w67 -> [w71]
                frame #0 {
                  # "The GPIB address of the ILX controller"
                  # "Specifying laser channel 1,\nwhich is the online channel"
                  n28 = local write "ILX Address"("ILX Address") -> ()
                  n29 = Number To Decimal String(number="ILX Address") -> (decimal integer string=w69:string)  [unwired: 1 in]
                  n30 = GPIB Write(0:w69, 1:"LAS:CHAN 2") -> ()  [unwired: 3 in, 2 out]
                }
                frame #1 {
                  # "Telling the controller to\nset the current"
                  # "string formatter"
                  # "Set current to specified current"
                  n31 = Format Into String(format string="%.4f" ("Format String"), "Lambda On DBR Current") -> (resulting string=w74:string)  [unwired: 2 in, 1 out]
                  n32 = local write "Lambda On DBR Current"("Lambda On DBR Current") -> ()
                  n33 = Concatenate Strings("LAS:LDI ", w74) -> (w75:string)
                  n34 = GPIB Write(0:w71, 1:w75) -> ()  [unwired: 3 in, 2 out]
                }
              }
            }
            frame #1 {
              # "This frame does not actually appear to do anything, I'm not sure why Amin originally put anything in this frame.  What does occur, \nis that the output current for the offline channel is specified and a command is generated, but, not written, to enable the output of the\noffline laser.  Although, the command is never written, as nearly as I can figure, the idea was that the offline never actually needs to be \naltered, so it will just be left in whatever state it started in upon the program startup."
              n35 = local read "ILX Address"() -> (w77:i32)
              n36 = Number To Decimal String(number=w77) -> ()  [unwired: 1 in, 1 out]
              n37 = Number To Engineering String(4:"Lambda Off DBR Current") -> (0:w81:string)  [unwired: 3 in]
              n38 = local write "Lambda Off DBR Current"("Lambda Off DBR Current") -> ()
              n39 = Concatenate Strings(":SOUR2:FUNC DC; :SOUR2:VOLT:OFFS ", w81, "V; :OUTP2:STAT ON") -> ()  [unwired: 1 out]
            }
            frame #2 {
              # "REPLACE WITH NEW AGILTRON TASK!"
              # "First one"
              # "Address of the Agiltron switch, only altered if the COM port changes,\nif the USB to serial converter changes or the usb port that is is plugged\nin to changes, this may vary.  Check the \"Devices and Printers\" and find \nout which com port the Agiltron switch is under should you see an error \nand adjust the adress on the front panel to match the switch address"
              # "Hex command written to \nthe switch for the online channel"
              # "Switch the Agiltron switch to the online channel, once switched, the online DBR is the laser seeding the TSOA"
              n40 = local read "Switch Comm Port"() -> (w82:refnum<visa-resource-name>)
              n41 = VISA Write(VISA resource name=w82, write buffer="\u0001\u0012\u0000\u0002") -> ()  [unwired: 1 in, 3 out]
            }
          }
        }
        frame Enabled {
        }
      }
      n42 = flat-sequence {
        tunnel: [w37] -> w35
        tunnel: w35 -> [w39]
        tunnel: [w45] -> w34
        tunnel: w34 -> [w48]
        frame #0 {
          # "The GPIB address of the ILX controller"
          # "Specifying laser channel 1,\nwhich is the online channel"
          n43 = local write "ILX Address On"("ILX Address On") -> ()
          n44 = Number To Decimal String(number="ILX Address On") -> (decimal integer string=w37:string)  [unwired: 1 in]
          n45 = GPIB Write(0:w37, 1:"LAS:CHAN 2") -> ()  [unwired: 3 in, 2 out]
        }
        frame #1 {
          # "Telling the controller to\nset the current"
          # "string formatter"
          # "Set current to specified current"
          n46 = Format Into String(format string="%.4f" ("Format String"), "OnLineLD") -> (resulting string=w42:string)  [unwired: 2 in, 1 out]
          n47 = local write "Lambda On DBR Current"("OnLineLD") -> ()
          n48 = Concatenate Strings("LAS:LDI ", w42) -> (w43:string)
          n49 = GPIB Write(0:w39, 1:w43) -> ()  [unwired: 3 in, 2 out]
        }
        frame #2 {
          # "The GPIB address of the ILX controller"
          # "Specifying laser channel 2,\nwhich is the offline channel"
          n50 = local write "ILX Address Off"("ILX Address Off") -> ()
          n51 = Number To Decimal String(number="ILX Address Off") -> (decimal integer string=w45:string)  [unwired: 1 in]
          n52 = GPIB Write(0:w45, 1:"LAS:CHAN 2") -> ()  [unwired: 3 in, 2 out]
        }
        frame #3 {
          # "Telling the controller to\nset the current"
          # "string formatter"
          # "Set current to specified current"
          n53 = Format Into String(format string="%.4f" ("Format String"), "OffLineLD") -> (resulting string=w51:string)  [unwired: 2 in, 1 out]
          n54 = local write "Lambda Off DBR Current"("OffLineLD") -> ()
          n55 = Concatenate Strings("LAS:LDI ", w51) -> (w52:string)
          n56 = GPIB Write(0:w48, 1:w52) -> ()  [unwired: 3 in, 2 out]
        }
      }
      n57 = disable-structure shown="Enabled" {
        frame Disabled {
          # "Initialize the ILX to the front panel temperatures and currents for the on line and off line DBRs\nTurn on the TECs - does not turn on the lasers or set the Agiltron switches"
          n58 = call "ILX2.vi"("ILX Command"=T7."Initialize ILX") -> ("Device Out"=w61:refnum<visa-resource-name>)  [unwired: 10 in, 4 out]
          n59 = call "ILX2.vi"("Device In"=w61, "TEC Control"=TRUE, "ILX Command"=T7."TEC ON/OFF") -> ("Device Out"=w58:refnum<visa-resource-name>)  [unwired: 8 in, 4 out]
          n60 = flat-sequence {
            tunnel: w58 -> [w65]
            tunnel: [w65] -> w55
            frame #0 {
              # "Wait 30 seconds for\nthe ILX to stabilize"
              n61 = Wait (ms)(milliseconds to wait=u32 30000) -> ()  [unwired: 1 out]
            }
          }
          n62 = call "ILX2.vi"("Device In"=w55, "ILX Command"=T7."LASER ON/OFF", "Laser Control"=TRUE ("TEC Control")) -> ("Device Out"=w54:refnum<visa-resource-name>)  [unwired: 8 in, 4 out]
          n63 = flat-sequence {
            tunnel: w54 -> [w63]
            tunnel: [w63] -> _
            frame #0 {
              # "Wait 5 seconds for\nthe ILX to stabilize"
              n64 = Wait (ms)(milliseconds to wait=u32 5000) -> ()  [unwired: 1 out]
            }
          }
        }
        frame Enabled {
        }
      }
    }
    frame #2 {
      # "Active X commands to the Newport 1918-C"
      # "Set the  channel of\nthe Newport 1918-C"
      # "Set the operational mode\nof the Newport 1918-C"
      # "Open commumication\nto the Newport 1918-C"
      n65 = constructor class="PowerMeterCommands"("logging"="logging", "deviceKey"="NewportIn") -> (reference out=w95:refnum<k24>, error out=w92:errorcluster, "deviceKey"=w87:string)  [unwired: 3 in, 2 out]
      "Newport Device Key" <- w87
      n66 = invoke class="PowerMeterCommands" method="GetPower"(reference=w95, error in=w92, "deviceKey"=w87) -> (reference out=w94:refnum<k24>, error out=w91:errorcluster)  [unwired: 1 in, 2 out]
      n67 = invoke class="PowerMeterCommands" method="SetChannel"(reference=w94, error in=w91, "deviceKey"=w87, "channel"="1") -> (reference out=w88:refnum<k24>, error out=w90:errorcluster)  [unwired: 1 in, 3 out]
      n68 = invoke class="PowerMeterCommands" method="CmdGetPower"(reference=w88, error in=w90, "deviceKey"=w87, "power"=sgl 0.0) -> (reference out=→"NewportRef":refnum<k24>)  [unwired: 1 in, 4 out]
    }
    frame #3 {
      # "Clean up multiply and divide by powers of 10 with comments\nBMM 6/19/14"
      # "Generating an array that is 'Number of Bins' long, filled wih the relevant altitude values for later plotting of Range \nCorrected Returns"
      # "Generating an array that is 'Number of Bins' long, filled wih the relevant altitude values for later plotting of returns"
      # "Generate arrays for the altitude and range corrected return altitude.  To be used later for plotting purposes."
      n69 = local read "Time Resolution Per Bin(ns)"() -> (w108:u32)
      n70 = local read "Time Resolution Per Bin(ns)"() -> (w98:u32)
      n71 = local read "Number of Bins"() -> (w111:u32)
      n72 = local read "Number of Bins"() -> (w101:u32)
      n73 = Divide(x=w108, y=1000000000.0) -> (x/y=w106:dbl)
      n74 = Divide(x=w98, y=1000000000.0) -> (x/y=w96:dbl)
      n75 = Multiply(x=w106, y=150000.0) -> (x*y=w109:dbl)
      n76 = Initialize Array(0.0, 0) -> (w114:dbl[])
      n77 = Multiply(x=w96, y=150000000.0) -> (x*y=w99:dbl)
      n78 = Initialize Array(0.0, 0) -> (w104:dbl[])
      n79 = for {
        N: w111 -> [_]
        shift-right: [w127] -> w112
        shift-left: w114 -> [w128]
        tunnel: w109 -> [w124]
        i -> [w126]
        n80 = Multiply(x=w124, y=w126) -> (x*y=w125:dbl)
        n81 = Add(x=w125, y=w124) -> (x+y=w123:dbl)
        n82 = Build Array (concatenate)(w128, w123) -> (w127:dbl[])
      }
      "Altitude Array (km)" <- w112
      n83 = for {
        N: w101 -> [_]
        shift-right: [w121] -> w102
        shift-left: w104 -> [w122]
        tunnel: w99 -> [w117]
        i -> [w120]
        n84 = Multiply(x=w117, y=w120) -> (x*y=w118:dbl)
        n85 = Add(x=w118, y=w117) -> (x+y=w116:dbl)
        n86 = Multiply(x=w116, y=w116) -> (x*y=w119:dbl)
        n87 = Build Array (concatenate)(w122, w119) -> (w121:dbl[])
      }
      "Range Corrected Altitude Array" <- w102
      n88 = local write "Altitude Array (km)"(w112) -> ()
      n89 = local write "Range Corrected Altitude Array"(w102) -> ()
    }
    frame #4 {
      # "Frame 4: Collect data from the scaler card and process and file it"
      n90 = while {
        tunnel: ["stop"] -> w129
        i -> [w130]
        stop <- "stop" stop-if-true
        # "While loop continues data collection cycle"
        n91 = case shown="True" "Collect Data?" {
          frame False {
            # "If 'Collect Data?' is false, wait a ms and check the 'Collect Data?' value again"
            n92 = Wait (ms)(milliseconds to wait=u32 1) -> ()  [unwired: 1 out]
          }
          frame True {
            # "Frame 3: Read the offline wavelength and lock if necessary (code not finished), read output power, read offline data, perform calculations and plot/save offline and NRB data, switch to online\nFrame 4: Calculate the absorption cross section (if wavelength, T, or P changed)\nFrame 5: Calculate Water Vapor Number density and plot"
            # "Frame 0: Create folders and file paths for logging the data, initialize averaging index\nFrame 1: Import current pressure and temperature data from COE weather station\nFrame 2: Read the online wavelength and lock if necessary, read online data and output power\n, plot and save online data, switch to offline DBR"
            # "If 'Collect Data?' is true, collect, process, and log data"
            n93 = stacked-sequence {
              frame #0 {
                # "Looking to see if the current Yr/Mo/Dy/Hr folder exists\nin the data disk folder (E:\\Micropulse_DIAL_data), if not,\ncreate one for the data"
                n94 = local read "FileHour"() -> (w143:i32)
                n95 = Get Date/Time In Seconds() -> (seconds since 1Jan1904=w135:timestamp)
                n96 = Seconds To Date/Time(time stamp (now)=w135) -> (date time rec=w145:T10)  [unwired: 1 in]
                n97 = Unbundle By Name(w145) -> ("hour"=w134:i32)
                n98 = Equal?(x=w143, y=w134) -> (x = y?=w144:bool)
                n99 = case shown="True" "Reset Average" {
                  frame False {
                    n100 = local write "Index"(0 ("Index")) -> ()
                  }
                  frame True {
                    n101 = local read "Index"() -> (w233:i32)
                    n102 = Add(x=w233, y=1) -> (x+y=w232:i32)
                    n103 = local write "Index"(w232) -> ()
                  }
                }
                n104 = Format Date/Time String(time format string (%c)="%y%m%d", seconds (now)=w135) -> (date/time string=w139:string)  [unwired: 1 in]
                n105 = Concatenate Strings("Data File DIR (in)", w139, "FF" ("string")) -> (w141:string)
                n106 = Concatenate Strings("Data File DIR (in)", w139, "NF" ("string")) -> (w136:string)
                n107 = case shown="False" w144 {
                  tunnel: w141 -> [w203 _]
                  tunnel: w136 -> [w202 _]
                  tunnel: w135 -> [w189 _]
                  tunnel: w134 -> [w165 _]
                  frame False {
                    # "Are data files open?"
                    # "Within the \"E:\\Micropulse_DIAL_data...\n'Current month/day/year' \ncheck if the current hour folder exists,\nif not, create one"
                    n108 = local write "FileHour"(w165) -> ()
                    n109 = flat-sequence {
                      tunnel: [w223] -> w190
                      tunnel: w203 -> [w222]
                      tunnel: w202 -> [w223]
                      tunnel: [w222] -> w191
                      frame #0 {
                        # "Does \"E:\\Micropulse_DIAL_data...\n'Current month/day/year' exist?\nIf not, create a new folder with that name"
                        n110 = String To Path(string=w222) -> (path=w227:path)
                        n111 = String To Path(string=w223) -> (path=w225:path)
                        n112 = call <vilib>:"Check if File or Folder Exists.vi"("path"=w227) -> ("file or folder exists?"=w226:bool)  [unwired: 8 in, 2 out]
                        n113 = call <vilib>:"Check if File or Folder Exists.vi"("path"=w225) -> ("file or folder exists?"=w224:bool)  [unwired: 8 in, 2 out]
                        n114 = case shown="False" w226 {
                          tunnel: w227 -> [w229 _]
                          frame False {
                            # "create new folder"
                            n115 = Create Folder(path (use dialog)=w229) -> ()  [unwired: 2 in, 3 out]
                          }
                          frame True {
                            # "Folder exists\ndo nothing"
                          }
                        }
                        n116 = case shown="False" w224 {
                          tunnel: w225 -> [w228 _]
                          frame False {
                            # "create new folder"
                            n117 = Create Folder(path (use dialog)=w228) -> ()  [unwired: 2 in, 3 out]
                          }
                          frame True {
                            # "Folder exists\ndo nothing"
                          }
                        }
                      }
                    }
                    n118 = Concatenate Strings(w191, "\\" ("string")) -> (w198:string)
                    n119 = Concatenate Strings(w190, "\\" ("string")) -> (w193:string)
                    n120 = Format Date/Time String(time format string (%c)="%H", seconds (now)=w189) -> (date/time string=w201:string)  [unwired: 1 in]
                    n121 = Format Date/Time String(time format string (%c)="%H", seconds (now)=w189) -> (date/time string=w196:string)  [unwired: 1 in]
                    n122 = Concatenate Strings(w198, w201) -> (w161:string)
                    "File Path_Far Field (out)" <- w161
                    n123 = Concatenate Strings(w193, w196) -> (w162:string)
                    "File Path_Near Field (out)" <- w162
                    n124 = String To Path(string=w161) -> (path=w199:path)
                    n125 = String To Path(string=w162) -> (path=w194:path)
                    n126 = call <vilib>:"Check if File or Folder Exists.vi"("path"=w199) -> ("file or folder exists?"=w188:bool, "dup path"=w186:path)  [unwired: 8 in, 1 out]
                    n127 = call <vilib>:"Check if File or Folder Exists.vi"("path"=w194) -> ("file or folder exists?"=w187:bool, "dup path"=w185:path)  [unwired: 8 in, 1 out]
                    n128 = case shown="False" w188 {
                      tunnel: w186 -> [w220 _]
                      tunnel: w161 -> [w219 w221]
                      tunnel: [w219 w221] -> w159
                      frame False {
                        # "new folder"
                        n129 = Create Folder(path (use dialog)=w220) -> ()  [unwired: 2 in, 3 out]
                      }
                      frame True {
                        # "Folder exists\ndo nothing"
                      }
                    }
                    n130 = case shown="False" w187 {
                      tunnel: w185 -> [w217 _]
                      tunnel: w162 -> [w216 w218]
                      tunnel: [w216 w218] -> w160
                      frame False {
                        # "new folder"
                        n131 = Create Folder(path (use dialog)=w217) -> ()  [unwired: 2 in, 3 out]
                      }
                      frame True {
                        # "Folder exists\ndo nothing"
                      }
                    }
                    n132 = Concatenate Strings(w160, "\\Online_Raw_Data.dat" ("string")) -> (w179:string)
                    n133 = Concatenate Strings(w160, "\\Offline_Raw_Data.dat" ("string")) -> (w178:string)
                    n134 = Concatenate Strings(w159, "\\Online_Raw_Data.dat" ("string")) -> (w184:string)
                    n135 = Concatenate Strings(w159, "\\Offline_Raw_Data.dat" ("string")) -> (w183:string)
                    n136 = local read "DataOpen"() -> (w176:bool)
                    n137 = String To Path(string=w184) -> (path=w175:path)
                    n138 = String To Path(string=w183) -> (path=w174:path)
                    n139 = String To Path(string=w179) -> (path=w173:path)
                    n140 = String To Path(string=w178) -> (path=w172:path)
                    n141 = case shown="True" w176 {
                      tunnel: w175 -> [w207 w211]
                      tunnel: [w207 w211] -> w169
                      tunnel: w174 -> [w206 w210]
                      tunnel: [w206 w210] -> w168
                      tunnel: w173 -> [w205 w209]
                      tunnel: [w205 w209] -> w167
                      tunnel: [w204 w208] -> w166
                      tunnel: w172 -> [w204 w208]
                      frame False {
                        # "No files open\ndo nothing"
                      }
                      frame True {
                        # "Close open files"
                        n142 = local read "NF_Off_Ref"() -> (w213:refnum<file>)
                        n143 = local read "NF_On_Ref"() -> (w212:refnum<file>)
                        n144 = local read "FF_Off_Ref"() -> (w215:refnum<file>)
                        n145 = local read "FF_On_Ref"() -> (w214:refnum<file>)
                        n146 = Close File(refnum=w214) -> ()  [unwired: 1 in, 2 out]
                        n147 = Close File(refnum=w215) -> ()  [unwired: 1 in, 2 out]
                        n148 = Close File(refnum=w212) -> ()  [unwired: 1 in, 2 out]
                        n149 = Close File(refnum=w213) -> ()  [unwired: 1 in, 2 out]
                      }
                    }
                    n150 = Open/Create/Replace File(file path (use dialog)=w169, operation (0:open)=T8."open or create") -> (refnum out=w155:refnum<file>)  [unwired: 4 in, 2 out]
                    n151 = Open/Create/Replace File(file path (use dialog)=w168, operation (0:open)=T8."open or create") -> (refnum out=w156:refnum<file>)  [unwired: 4 in, 2 out]
                    n152 = Open/Create/Replace File(file path (use dialog)=w167, operation (0:open)=T8."open or create") -> (refnum out=w157:refnum<file>)  [unwired: 4 in, 2 out]
                    n153 = Open/Create/Replace File(file path (use dialog)=w166, operation (0:open)=T8."open or create") -> (refnum out=w158:refnum<file>)  [unwired: 4 in, 2 out]
                    n154 = Get File Size(file=w155) -> (refnum out=→"FF_On_Ref":refnum<file>, size (in bytes)=→"FF_On_Ptr":i64)  [unwired: 1 in, 1 out]
                    n155 = Get File Size(file=w156) -> (refnum out=→"FF_Off_Ref":refnum<file>, size (in bytes)=→"FF_Off_Ptr":i64)  [unwired: 1 in, 1 out]
                    n156 = Get File Size(file=w157) -> (refnum out=→"NF_On_Ref":refnum<file>, size (in bytes)=→"NF_On_Ptr":i64)  [unwired: 1 in, 1 out]
                    n157 = Get File Size(file=w158) -> (refnum out=→"NF_Off_Ref":refnum<file>, size (in bytes)=→"NF_Off_Ptr":i64)  [unwired: 1 in, 1 out]
                  }
                  frame True {
                    # "Don't need to do anything!"
                  }
                }
              }
              frame #1 {
                # "Writing and plotting retrieved\nweather parameters"
                # "Matlab script goes online and retrieves most recent press, temp, and relative humidity data \nfrom the weather station on the roof of Cobleigh"
                # "Importing the current weather conditions from the COE weather station"
                n158 = disable-structure shown="Disabled" {
                  frame Disabled {
                    n159 = script code="%try\n%s=urlread('http://www.coe.montana.edu/ee/weather/mostCurrentCSV.php');\n%amin=textscan(s,'%s %s %s %s %s %s %s %s %s %s %s %s %s');\n%data=amin{1}{2};\n%[test remain]=strtok(data,',');\n%remain=str2num(remain);\n%press=remain(3)./1000;\n%temp=remain(5);\n%RH=remain(7);\n%catch\npress=.850;\ntemp=20;\nRH=40;\n%end"() -> ()  [unwired: 1 in, 4 out]
                  }
                  frame Enabled {
                  }
                }
                n160 = local read "WS_On/Off"() -> (w234:bool)
                n161 = case shown="True" w234 {
                  frame False {
                  }
                  frame True {
                    n162 = local read "WS visa"() -> (w239:refnum<visa-resource-name>)
                    n163 = call "T_RH_P.vi"("VISA in"=w239, "WS_Commands"=enum16{"OpenWS", "ReadTRHP", "CloseWS"}."ReadTRHP") -> ("TRHP"=w235:T9)  [unwired: 11 in, 2 out]
                    n164 = local write "TRHP"(w235) -> ()
                    n165 = Unbundle By Name(w235) -> ("Temp"=→"Temperature (C)":dbl, "RelH"=→"Relative Humdity (%)":dbl, "Press"=→"Pressure (mb)":dbl)
                  }
                }
              }
              frame #2 {
                # "Frame 3: Read, process, and plot online data\nFrame 4:\nFrame 5: Write the data to the folders from Frame 0 of outter sequence"
                # "Frame 0: Read the online wavelength and adjust to locking tolerance if out of range, Switch to offline DBR\nFrame 1: Read the output power from the Newport meter, calculate and plot the output pulse energy\nFrame 2: Wait 'Scalar Wait Time' for buffer to clear other wavelength data"
                # "Online"
                n166 = stacked-sequence {
                  frame #0 {
                    # "Read the online wavelength and continue adjusting the online DBR if outside the wavelength tolerance\nuntil it is within tolerance"
                    n167 = while {
                      i -> [w244]
                      stop <- w241 stop-if-true
                      # "Frame 2: Decrement DBR current if above tolerance\nFrame 3: Increment DBR current if below tolerance"
                      # "Frame 0: Read the current wavelength from the wavemeter\nFrame 1: Calculate the difference between desired and actual wavelength"
                      # "Continue reading and adjusting online DBR current until within locking tolerance"
                      n168 = local read "ILX Address On"() -> (w245:dbl)
                      n169 = stacked-sequence {
                        tunnel: w245 -> [_ _ _ w270 w289]
                        tunnel: w244 -> [w247 _ _ _ _]
                        tunnel: [_ _ w260 _ _] -> w242
                        frame #0 {
                          n170 = Equal To 0?(x=w247) -> (x = 0?=w246:bool)
                          n171 = case shown="True" w246 {
                            frame False {
                            }
                            frame True {
                              # "Set the TSOA switch to\namplify the ABSORBING\nwavelength"
                              n172 = Build Array(FALSE ("Boolean")) -> (w248:bool[])
                              n173 = call-poly <vilib>:"DAQmx Write.vi"("task/channels in"=refnum<k21> "BristolWM", "data"=w248) -> ()  [unwired: 11 in, 3 out]
                            }
                          }
                        }
                        frame #1 {
                          # "Reading the wavelength from the wavemeter"
                          n174 = flat-sequence {
                            tunnel: [w253] -> w252
                            tunnel: w252 -> [w256]
                            tunnel: [w255] -> w251
                            tunnel: w251 -> [w259]
                            frame #0 {
                              n175 = local read "Bristol In"() -> (w254:i32)
                              n176 = dll-call lib="C:/Users/H2ODial/Desktop/Shared Telescope WV DIAL Code/Libraries and VIs/CLDevIface.dll" fn="CLOpenUSBSerialDevice"("commPort"=w254) -> ("return type"=w253:i32)  [unwired: 4 in, 2 out]
                            }
                            frame #1 {
                              n177 = dll-call lib="C:/Users/H2ODial/Desktop/Shared Telescope WV DIAL Code/Libraries and VIs/CLDevIface.dll" fn="CLGetLambdaReading"("devHandle"=w256) -> ("return type"=→"Lambda On Read (nm)":dbl, "devHandle"=w255:i32)  [unwired: 3 in, 2 out]
                            }
                            frame #2 {
                              n178 = dll-call lib="C:/Users/H2ODial/Desktop/Shared Telescope WV DIAL Code/Libraries and VIs/CLDevIface.dll" fn="CLCloseDevice"("commPort"=w259) -> ("return type"=w258:i32)  [unwired: 4 in, 2 out]
                              n179 = local write "Bristol Out"(w258) -> ()
                            }
                          }
                        }
                        frame #2 {
                          # "If WL difference is within tolerance, stop looping, and illuminate 'Wavelength Lock Online' indicator"
                          # "Calculating the difference between the actual and desired online wavelength"
                          n180 = local read "Lambda On Read (nm)"() -> (w268:dbl)
                          n181 = local read "Online_Tol"() -> (w265:dbl)
                          n182 = Multiply(x=-1.0, y=w265) -> (x*y=w266:dbl)
                          n183 = Subtract(x=w268, y="Lambda On Set (nm)") -> (x-y=w261:dbl)
                          "WL_Difference" <- w261
                          n184 = Greater?(x=w261, y=w266) -> (0:w262:bool)
                          n185 = Less?(x=w261, y=w265) -> (x < y?=w263:bool)
                          n186 = And(x=w262, y=w263) -> (x .and. y?=w260:bool)
                          "Wavelength Lock Online" <- w260
                        }
                        frame #3 {
                          # "If the wavelength difference is greater that 0.0002 nm, decrement the \nDBR current by 0.01 mA"
                          n187 = local read "WL_Difference"() -> (w272:dbl)
                          n188 = Greater Or Equal?(x=w272, y="Online_Tol") -> (x >= y?=w271:bool)
                          n189 = case shown="True" w271 {
                            tunnel: w270 -> [_ w273]
                            frame False {
                              # "Wavelength difference is not greater than 0.0002 nm, do nothing"
                            }
                            frame True {
                              n190 = stacked-sequence {
                                tunnel: w273 -> [w274 w277]
                                frame #0 {
                                # "Specifying laser channel 1,\nwhich is the online channel"
                                n191 = Number To Decimal String(number=w274) -> (decimal integer string=w275:string)  [unwired: 1 in]
                                n192 = GPIB Write(0:w275, 1:"LAS:CHAN 2") -> ()  [unwired: 3 in, 2 out]
                                }
                                frame #1 {
                                # "issuing the command"
                                # "Generating a command string\nto decrement the current"
                                # "WL difference is greater than 0.0002 nm,\ndecrement the DBR current by 0.01 mA"
                                n193 = local read "Lambda On DBR Current"() -> (w284:dbl)
                                n194 = Subtract(x=w284, y=0.01) -> (x-y=w278:dbl)
                                n195 = local write "Lambda On DBR Current"(w278) -> ()
                                n196 = Format Into String(format string="%.4f" ("Format String"), w278) -> (resulting string=w281:string)  [unwired: 2 in, 1 out]
                                n197 = Concatenate Strings("LAS:LDI ", w281) -> (w280:string)
                                n198 = Number To Decimal String(number=w277) -> (decimal integer string=w279:string)  [unwired: 1 in]
                                n199 = GPIB Write(0:w279, 1:w280) -> ()  [unwired: 3 in, 2 out]
                                }
                              }
                            }
                          }
                        }
                        frame #4 {
                          # "If WL difference is < 0.0002 nm, increment the DBR current"
                          n200 = local read "Online_Tol"() -> (w287:dbl)
                          n201 = local read "WL_Difference"() -> (w291:dbl)
                          n202 = Multiply(x=-1.0, y=w287) -> (x*y=w286:dbl)
                          n203 = Less Or Equal?(x=w291, y=w286) -> (x <= y?=w290:bool)
                          n204 = case shown="True" w290 {
                            tunnel: w289 -> [_ w292]
                            frame False {
                              # "WL difference is no <= to -0.0002 nm, do nothing"
                            }
                            frame True {
                              n205 = stacked-sequence {
                                tunnel: w292 -> [w294 w296]
                                frame #0 {
                                # "Specifying laser channel 1,\nwhich is the online channel"
                                n206 = Number To Decimal String(number=w294) -> (decimal integer string=w293:string)  [unwired: 1 in]
                                n207 = GPIB Write(0:w293, 1:"LAS:CHAN 2") -> ()  [unwired: 3 in, 2 out]
                                }
                                frame #1 {
                                # "issuing the command"
                                # "Generating a command \nstring to increment the current"
                                # "WL difference is < -0.0002,\nincrement the DBR current by 0.01 mA"
                                n208 = local read "Lambda On DBR Current"() -> (w303:dbl)
                                n209 = Add(x=w303, y=0.01) -> (x+y=w298:dbl)
                                n210 = local write "Lambda On DBR Current"(w298) -> ()
                                n211 = Format Into String(format string="%.4f" ("Format String"), w298) -> (resulting string=w300:string)  [unwired: 2 in, 1 out]
                                n212 = Concatenate Strings("LAS:LDI ", w300) -> (w299:string)
                                n213 = Number To Decimal String(number=w296) -> (decimal integer string=w297:string)  [unwired: 1 in]
                                n214 = GPIB Write(0:w297, 1:w299) -> ()  [unwired: 3 in, 2 out]
                                }
                              }
                            }
                          }
                        }
                      }
                      n215 = Or(x=w242, y="Cancel online") -> (x .or. y?=w241:bool)
                    }
                  }
                  frame #1 {
                    # "Converting to pulse energy, assumes 5 percent pickoff"
                    # "Reading the Newport Power meter"
                    # "Reading the output power of the laser transmitter from the Newport power meter, once read, convert to corresponding pulse energy and plot"
                    n216 = local read "Newport Device Key"() -> (w309:string)
                    n217 = local read "NewportRef"() -> (w305:refnum<k24>)
                    n218 = disable-structure shown="Disabled" {
                      frame Disabled {
                        # "Plotting the online and offling pulse energies"
                        n219 = local read "Online Pulse Energy"() -> (w320:dbl)
                        n220 = local read "Offline Pulse Energy"() -> (w319:dbl)
                        n221 = Bundle("Online Pulse Energy"=w320, "Offline Pulse Energy"=w319) -> (→"Pulse Energy (Micro Joule)":T11)  [unwired: 1 in]
                      }
                      frame Enabled {
                      }
                    }
                    n222 = Number To Decimal String(number="SampleSize") -> (decimal integer string=w307:string)  [unwired: 1 in]
                    n223 = invoke class="PowerMeterCommands" method="PerformDAQ"(reference=w305, "deviceKey"=w309, "interval"="1", "sampleSize"=w307) -> ("PerformDAQ"=w310:dbl[])  [unwired: 2 in, 5 out]
                    n224 = call-poly <vilib>:"Mean.vi"("X"=w310) -> ("mean"=w308:dbl)  [unwired: 1 out]
                    n225 = Multiply(x=w308, y=1000.0) -> (x*y=w316:dbl)
                    n226 = Divide(x=w316, y=0.05) -> (x/y=w314:dbl)
                    n227 = Divide(x=w314, y=7.0) -> (x/y=→"Online Pulse Energy":dbl)
                  }
                  frame #2 {
                    # "Wait 'Scalar Wait Time' for the next available batch of scalar card data"
                    n228 = local read "AMCS_Profile"() -> (w321:i32)
                    n229 = disable-structure shown="Disabled" {
                      frame Disabled {
                        # "Waiting 'Scalar Wait Time'"
                        n230 = Wait (ms)(milliseconds to wait="Scalar Wait Time") -> ()  [unwired: 1 out]
                      }
                      frame Enabled {
                      }
                    }
                    n231 = while {
                      tunnel: [w328] -> w322
                      tunnel: [w324] -> _
                      tunnel: w321 -> [w324]
                      stop <- w326 stop-if-true
                      n232 = global read "AMCS_Data.vi" "AMCS_Profile"() -> (w328:i32)
                      n233 = Wait (ms)(milliseconds to wait=u32 10) -> ()  [unwired: 1 out]
                      n234 = Equal?(x=w328, y=w324) -> (x = y?=w327:bool)
                      n235 = case shown="False" w327 {
                        tunnel: [TRUE FALSE] -> w326
                        frame False {
                        }
                        frame True {
                        }
                      }
                    }
                    "AMCS_Profile" <- w322
                  }
                  frame #3 {
                    # "convert time per range bin to meters\nand calculate smoothed bins using\nsmoothing range"
                    # "Plotting online cross section and smoothed online data"
                    # "Calculate the bin by bin mean of the data"
                    # "Collect 'Integration Period (Seconds)' number\nof scalar data"
                    # "Reading, processing, and plotting the online data"
                    n236 = local read "Data Reads (number of loops)"() -> (w356:i32)
                    n237 = for {
                      N: w356 -> [_]
                      tunnel: [w377] -> w368 mode=indexing
                      tunnel: [w376] -> w331 mode=indexing
                      # "Scalar Data is retrieved from Global \nVariable that scaler.vi is writing to,"
                      n238 = global read "AMCS_Data.vi" "AMCS_Data"() -> (w380:u16[][])
                      n239 = disable-structure shown="Disabled" {
                        frame Disabled {
                          n240 = global read "Scalar_Data_3.vi" "Scalar Data 3"() -> ()  [unwired: 1 out]
                          n241 = global read "Scalar_Data.vi" "Scalar Data"() -> ()  [unwired: 1 out]
                        }
                        frame Enabled {
                        }
                      }
                      n242 = Index Array(array=w380, index (row) #1=0 ("index (row)"), index (row) #2=2 ("index (row)")) -> (element #1=w377:u16[], element #2=w376:u16[])  [unwired: 2 in]
                    }
                    n243 = Transpose 2D Array(2D array=w368) -> (transposed array=w372:u16[][])
                    n244 = Transpose 2D Array(2D array=w331) -> (transposed array=w354:u16[][])
                    n245 = for {
                      tunnel: w372 -> [w382] mode=indexing
                      tunnel: [w381] -> w373 mode=indexing
                      n246 = call-poly <vilib>:"Mean.vi"("X"=w382) -> ("mean"=w381:dbl)  [unwired: 1 out]
                    }
                    n247 = for {
                      tunnel: w354 -> [w375] mode=indexing
                      tunnel: [w374] -> w355 mode=indexing
                      n248 = call-poly <vilib>:"Mean.vi"("X"=w375) -> ("mean"=w374:dbl)  [unwired: 1 out]
                    }
                    n249 = local read "bins"() -> (w348:u32)
                    n250 = Array Subset(array=w373, index=1 ("dimension size"), length=w348) -> (w360:dbl[])
                    n251 = Array Subset(array=w355, index=1 ("dimension size"), length=w348) -> (w352:dbl[])
                    n252 = local read "background length"() -> (w338:i32)
                    n253 = local read "background start"() -> (w339:u32)
                    n254 = Array Size(array=w360) -> (size(s)=w357:i32)
                    n255 = Array Size(array=w352) -> (size(s)=w349:i32)
                    n256 = Initialize Array(1.0 ("element"), w357) -> (w359:dbl[])
                    n257 = Initialize Array(1.0 ("element"), w349) -> (w351:dbl[])
                    n258 = Multiply(x=w360, y=w359) -> (x*y=w361:dbl[])
                    "On-Line Bin Readings" <- w361
                    n259 = Multiply(x=w352, y=w351) -> (x*y=w342:dbl[])
                    "On-Line Bin Readings 2" <- w342
                    n260 = local read "Total DIAL Integration Time (Minutes)"() -> (w364:i32)
                    n261 = local read "Time Resolution Per Bin(ns)"() -> (w334:u32)
                    n262 = Array Subset(array=w361, index=w339, length=w338) -> (w370:dbl[])
                    n263 = Array Subset(array=w342, index=w339, length=w338) -> (w344:dbl[])
                    n264 = call-poly <vilib>:"Mean.vi"("X"=w370) -> ("mean"=w369:dbl)  [unwired: 1 out]
                    n265 = call-poly <vilib>:"Mean.vi"("X"=w344) -> ("mean"=w345:dbl)  [unwired: 1 out]
                    n266 = Divide(x=w364, y=w356) -> (x/y=w362:dbl)
                    n267 = local read "Index"() -> (w343:i32)
                    n268 = Subtract(x=w361, y=w369) -> (x-y=w366:dbl[])
                    n269 = Subtract(x=w342, y=w345) -> (x-y=w346:dbl[])
                    n270 = To Double Precision Float(number=w334) -> (double precision float=w335:dbl)
                    n271 = Multiply(x=w362, y=60.0) -> (x*y=w340:dbl)
                    n272 = Multiply(x=w335, y=0.15) -> (x*y=w337:dbl)
                    n273 = call "Ring Buffer Online Far.vi"("Index"=w343, "Profiles to Average"=w340, "Input Array"=w366) -> ("AvgArray"=w365:dbl[])  [unwired: 7 in, 1 out]
                    n274 = call "Ring Buffer Online Near.vi"("Index"=w343, "Profiles to Average"=w340, "Input Array"=w346) -> ("AvgArray"=w347:dbl[])  [unwired: 7 in, 1 out]
                    n275 = Divide(x="Smoothing Range", y=w337) -> (x/y=w332:dbl)
                    "Smoothed Bins" <- w332
                    n276 = call "Smooth Arrray.vi"("smooth size"=w332, "Raw Array"=w365) -> ("Smoothed Array"=→"On-Line  Smoothed":dbl[])  [unwired: 9 in]
                    n277 = call "Smooth Arrray.vi"("smooth size"=w332, "Raw Array"=w347) -> ("Smoothed Array"=→"On-Line Smoothed 2":dbl[])  [unwired: 9 in]
                    n278 = disable-structure shown="Disabled" {
                      frame Disabled {
                        n279 = script code="format long;\ncounts=sum(Online);\nif counts >=0.5e6\ntime=time;\nelse\ntime=time\nend"() -> ()  [unwired: 3 in, 2 out]
                      }
                      frame Enabled {
                      }
                    }
                  }
                  frame #4 {
                    # "Toggling the Agiltron switch to the offline DBR seed laser"
                    n280 = disable-structure shown="Disabled" {
                      frame Disabled {
                        n281 = flat-sequence {
                          frame #0 {
                            # "Second one"
                            # "Command the switch to switch to position 2\ncorresponding to the offline DBR"
                            # "Hex string command \ncorrespond to offline"
                            n282 = VISA Write(VISA resource name="Switch Comm Port", write buffer="\u0001\u0012\u0000\u0001") -> ()  [unwired: 1 in, 3 out]
                          }
                        }
                      }
                      frame Enabled {
                      }
                    }
                  }
                  frame #5 {
                    # "Save the recently collected online data if 'Save Data?' is true"
                    n283 = case shown="True" "Save Data?" {
                      frame False {
                        # "'Save Data?' is false, do nothing"
                      }
                      frame True {
                        # "'Save Data?' is true, save onfline data to the Data Disk"
                        # "Write only one copy of data at this time"
                        # "Retrieve Julian Date"
                        n284 = local read "Time Resolution Per Bin(ns)"() -> (w391:u32)
                        n285 = local read "Number of Accumulates"() -> (w389:u32)
                        n286 = local read "Number of Bins"() -> (w390:u32)
                        n287 = local read "Lambda On DBR Current"() -> (w413:dbl)
                        n288 = local read "Lambda On Read (nm)"() -> (w414:dbl)
                        n289 = local read "On-Line Bin Readings 2"() -> (w411:dbl[])
                        n290 = local read "On-Line Bin Readings"() -> (w416:dbl[])
                        n291 = local read "Online Pulse Energy"() -> (w412:dbl)
                        n292 = To Double Precision Float(number=w391) -> (double precision float=w386:dbl)
                        n293 = To Double Precision Float(number=w390) -> (double precision float=w387:dbl)
                        n294 = To Double Precision Float(number=w389) -> (double precision float=w388:dbl)
                        n295 = call "Julian_Date_2.vi"() -> ("Julian Date"=w415:dbl)  [unwired: 11 in]
                        n296 = Build Array (concatenate)(w415, w414, w413, w412, w386, w387, w388, w416) -> (w406:dbl[])
                        n297 = Build Array (concatenate)(w415, w414, w413, w412, w386, w387, w388, w411) -> (w396:dbl[])
                        n298 = local write "DataOpen"(TRUE ("DataOpen")) -> ()
                        n299 = local read "NF_On_Ref"() -> (w394:refnum<file>)
                        n300 = local read "FF_On_Ref"() -> (w410:refnum<file>)
                        n301 = local read "NF_On_Ptr"() -> (w395:i64)
                        n302 = local read "FF_On_Ptr"() -> (w409:i64)
                        n303 = Set File Position(offset (in bytes) (0)=w409, refnum=w410) -> (refnum out=w407:refnum<file>, error out=w404:errorcluster)  [unwired: 2 in]
                        n304 = Set File Position(offset (in bytes) (0)=w395, refnum=w394) -> (refnum out=w400:refnum<file>, error out=w398:errorcluster)  [unwired: 2 in]
                        n305 = Write to Binary File(file (use dialog)=w400, data=w396, error in=w398, 5:FALSE ("prepend array or string size? (T)")) -> (refnum out=w399:refnum<file>, error out=w397:errorcluster)  [unwired: 2 in, 1 out]
                        n306 = Write to Binary File(file (use dialog)=w407, data=w406, error in=w404, 5:FALSE ("prepend array or string size? (T)")) -> (refnum out=w405:refnum<file>, error out=w403:errorcluster)  [unwired: 2 in, 1 out]
                        n307 = Get File Position(4:w397, 7:w399) -> (2:w393:i64)  [unwired: 2 out]
                        n308 = Get File Position(4:w403, 7:w405) -> (2:w402:i64)  [unwired: 2 out]
                        n309 = local write "NF_On_Ptr"(w393) -> ()
                        n310 = local write "FF_On_Ptr"(w402) -> ()
                      }
                    }
                  }
                }
              }
              frame #3 {
                # "Frame 3: Read offline data, calculate aerosol data, and plot offline and normalized relative backscatter\nFrame 4:\nFrame 5: Save the offline data and related information"
                # "Frame 0: Read the offline wavelength and lock if necessary, Switch to online DBR\nFrame 1: Read the output power from the Newport power meter\nFrame 2: Wait 'Scalar Wait Time' for buffers to clear of online contiminated data"
                # "offline"
                n311 = stacked-sequence {
                  frame #0 {
                    # "Every 60 data collection cycles, read the offline DBR wavelength, and if outside of wavelength tolerance, adjust DBR current until within tolerance"
                    n312 = local read "L_Count"() -> (w418:i32)
                    n313 = Quotient & Remainder(x=w418, y=60.0) -> (x-y*floor(x/y)=w419:dbl)  [unwired: 1 out]
                    n314 = Equal To 0?(x=w419) -> (x = 0?=w417:bool)
                    n315 = case shown="True" w417 {
                      frame False {
                      }
                      frame True {
                        n316 = while {
                          i -> [w424]
                          stop <- w422 stop-if-true
                          # "If WL difference is within tolerance, stop looping, and illuminate 'Wavelength Lock Offline' indicator"
                          # "Frame 2: Decrement DBR current if above tolerance\nFrame 3: Increment DBR current if below tolerance"
                          # "Frame 0: Read the current wavelength from the wavemeter\nFrame 1: Calculate the difference between desired and actual wavelength"
                          # "Continue reading and adjusting offline DBR current until within locking tolerance"
                          n317 = local read "ILX Address Off"() -> (w425:dbl)
                          n318 = stacked-sequence {
                            tunnel: w425 -> [_ _ _ w455 w471]
                            tunnel: w424 -> [w427 _ _ _ _]
                            tunnel: [_ _ w441 _ _] -> w421
                            frame #0 {
                              n319 = Equal To 0?(x=w427) -> (x = 0?=w426:bool)
                              n320 = case shown="True" w426 {
                                frame False {
                                }
                                frame True {
                                # "Set the TSOA switch to\namplify the non ABSORBING\nwavelength"
                                n321 = Build Array(TRUE ("Boolean")) -> (w429:bool[])
                                n322 = call-poly <vilib>:"DAQmx Write.vi"("task/channels in"=refnum<k21> "BristolWM", "data"=w429) -> ()  [unwired: 11 in, 3 out]
                                n323 = Wait (ms)(milliseconds to wait=u32 3200) -> ()  [unwired: 1 out]
                                }
                              }
                            }
                            frame #1 {
                              # "Reading the wavelength from the wavemeter"
                              n324 = flat-sequence {
                                tunnel: [w434] -> w433
                                tunnel: w433 -> [w437]
                                tunnel: [w436] -> w432
                                tunnel: w432 -> [w440]
                                frame #0 {
                                n325 = local read "Bristol In"() -> (w435:i32)
                                n326 = dll-call lib="C:/Users/H2ODial/Desktop/Shared Telescope WV DIAL Code/Libraries and VIs/CLDevIface.dll" fn="CLOpenUSBSerialDevice"("commPort"=w435) -> ("return type"=w434:i32)  [unwired: 4 in, 2 out]
                                }
                                frame #1 {
                                n327 = dll-call lib="C:/Users/H2ODial/Desktop/Shared Telescope WV DIAL Code/Libraries and VIs/CLDevIface.dll" fn="CLGetLambdaReading"("devHandle"=w437) -> ("return type"=→"Lambda Off Read (nm)":dbl, "devHandle"=w436:i32)  [unwired: 3 in, 2 out]
                                }
                                frame #2 {
                                n328 = dll-call lib="C:/Users/H2ODial/Desktop/Shared Telescope WV DIAL Code/Libraries and VIs/CLDevIface.dll" fn="CLCloseDevice"("commPort"=w440) -> ("return type"=w439:i32)  [unwired: 4 in, 2 out]
                                n329 = local write "Bristol Out"(w439) -> ()
                                }
                              }
                            }
                            frame #2 {
                              # "Calculating the difference between the actual and desired online wavelength"
                              n330 = local read "Offline_Tol"() -> (w443:dbl)
                              n331 = local read "Lambda Off Read (nm)"() -> (w449:dbl)
                              n332 = Multiply(x=-1.0, y=w443) -> (x*y=w442:dbl)
                              n333 = Subtract(x=w449, y="Lambda Off Set (nm)") -> (x-y=w445:dbl)
                              "WL Difference off" <- w445
                              n334 = Greater?(x=w445, y=w442) -> (0:w446:bool)
                              n335 = Less?(x=w445, y=w443) -> (x < y?=w447:bool)
                              n336 = And(x=w446, y=w447) -> (x .and. y?=w441:bool)
                              "Wavelength Lock Offline" <- w441
                              n337 = case shown="True" w441 {
                                frame False {
                                }
                                frame True {
                                # "Set the TSOA switch to\namplify the ABSORBING\nwavelength"
                                n338 = Build Array(FALSE ("Boolean")) -> (w451:bool[])
                                n339 = call-poly <vilib>:"DAQmx Write.vi"("task/channels in"=refnum<k21> "BristolWM", "data"=w451) -> ()  [unwired: 11 in, 3 out]
                                n340 = Wait (ms)(milliseconds to wait=u32 3200) -> ()  [unwired: 1 out]
                                }
                              }
                            }
                            frame #3 {
                              # "If the wavelength difference is greater that 0.0002 nm, decrement the \nDBR current by 0.01 mA"
                              n341 = local read "WL Difference off"() -> (w457:dbl)
                              n342 = Greater Or Equal?(x=w457, y="Offline_Tol") -> (x >= y?=w456:bool)
                              n343 = case shown="True" w456 {
                                tunnel: w455 -> [_ w458]
                                frame False {
                                # "Wavelength difference is not greater than 0.0002 nm, do nothing"
                                }
                                frame True {
                                n344 = stacked-sequence {
                                tunnel: w458 -> [w459 w462]
                                frame #0 {
                                # "Specifying laser channel 1,\nwhich is the online channel"
                                n345 = Number To Decimal String(number=w459) -> (decimal integer string=w460:string)  [unwired: 1 in]
                                n346 = GPIB Write(0:w460, 1:"LAS:CHAN 2") -> ()  [unwired: 3 in, 2 out]
                                }
                                frame #1 {
                                # "issuing the command"
                                # "Generating a command string\nto decrement the current"
                                # "WL difference is greater than 0.0002 nm,\ndecrement the DBR current by 0.01 mA"
                                n347 = local read "Lambda Off DBR Current"() -> (w469:dbl)
                                n348 = Subtract(x=w469, y=0.01) -> (x-y=w463:dbl)
                                n349 = local write "Lambda Off DBR Current"(w463) -> ()
                                n350 = Format Into String(format string="%.4f" ("Format String"), w463) -> (resulting string=w466:string)  [unwired: 2 in, 1 out]
                                n351 = Concatenate Strings("LAS:LDI ", w466) -> (w465:string)
                                n352 = Number To Decimal String(number=w462) -> (decimal integer string=w464:string)  [unwired: 1 in]
                                n353 = GPIB Write(0:w464, 1:w465) -> ()  [unwired: 3 in, 2 out]
                                }
                                }
                                }
                              }
                            }
                            frame #4 {
                              # "If WL difference is < 0.0002 nm, increment the DBR current"
                              n354 = local read "WL Difference off"() -> (w474:dbl)
                              n355 = Less Or Equal?(x=w474, y=-0.0001) -> (x <= y?=w472:bool)
                              n356 = case shown="True" w472 {
                                tunnel: w471 -> [_ w475]
                                frame False {
                                # "WL difference is no <= to -0.0002 nm, do nothing"
                                }
                                frame True {
                                n357 = stacked-sequence {
                                tunnel: w475 -> [w477 w479]
                                frame #0 {
                                # "Specifying laser channel 1,\nwhich is the online channel"
                                n358 = Number To Decimal String(number=w477) -> (decimal integer string=w476:string)  [unwired: 1 in]
                                n359 = GPIB Write(0:w476, 1:"LAS:CHAN 2") -> ()  [unwired: 3 in, 2 out]
                                }
                                frame #1 {
                                # "issuing the command"
                                # "Generating a command \nstring to increment the current"
                                # "WL difference is < -0.0002,\nincrement the DBR current by 0.01 mA"
                                n360 = local read "Lambda Off DBR Current"() -> (w486:dbl)
                                n361 = Add(x=w486, y=0.01) -> (x+y=w481:dbl)
                                n362 = local write "Lambda Off DBR Current"(w481) -> ()
                                n363 = Format Into String(format string="%.4f" ("Format String"), w481) -> (resulting string=w483:string)  [unwired: 2 in, 1 out]
                                n364 = Concatenate Strings("LAS:LDI ", w483) -> (w482:string)
                                n365 = Number To Decimal String(number=w479) -> (decimal integer string=w480:string)  [unwired: 1 in]
                                n366 = GPIB Write(0:w480, 1:w482) -> ()  [unwired: 3 in, 2 out]
                                }
                                }
                                }
                              }
                            }
                          }
                          n367 = Or(x=w421, y="Cancel Offline") -> (x .or. y?=w422:bool)
                        }
                      }
                    }
                  }
                  frame #1 {
                    # "Reading the power meter"
                    # "Updating the pulse energy plot"
                    # "Converting to pulse energy"
                    # "Reading the offline output power, converting to pulse energy,  and updating the Pulse energy plot"
                    n368 = local read "SampleSize"() -> (w490:i32)
                    n369 = local read "Newport Device Key"() -> (w491:string)
                    n370 = local read "Online Pulse Energy"() -> (w497:dbl)
                    n371 = local read "Offline Pulse Energy"() -> (w496:dbl)
                    n372 = local read "NewportRef"() -> (w488:refnum<k24>)
                    n373 = Number To Decimal String(number=w490) -> (decimal integer string=w492:string)  [unwired: 1 in]
                    n374 = invoke class="PowerMeterCommands" method="PerformDAQ"(reference=w488, "deviceKey"=w491, "interval"="1", "sampleSize"=w492) -> ("PerformDAQ"=w493:dbl[])  [unwired: 2 in, 5 out]
                    n375 = Bundle("Online Pulse Energy"=w497, "Offline Pulse Energy"=w496) -> (w495:T11)  [unwired: 1 in]
                    n376 = local write "Pulse Energy (Micro Joule)"(w495) -> ()
                    n377 = call-poly <vilib>:"Mean.vi"("X"=w493) -> ("mean"=w489:dbl)  [unwired: 1 out]
                    n378 = Multiply(x=w489, y=1000.0) -> (x*y=w502:dbl)
                    n379 = Divide(x=w502, y=0.05) -> (x/y=w500:dbl)
                    n380 = Divide(x=w500, y=7.0) -> (x/y=→"Offline Pulse Energy":dbl)
                  }
                  frame #2 {
                    # "Wait 'Scalar Wait Time' for buffers to clear of online contiminated offline data"
                    n381 = disable-structure shown="Disabled" {
                      frame Disabled {
                        # "Wait 'Scalar Wait Time'"
                        n382 = local read "Scalar Wait Time"() -> (w504:u32)
                        n383 = Wait (ms)(milliseconds to wait=w504) -> ()  [unwired: 1 out]
                      }
                      frame Enabled {
                      }
                    }
                  }
                  frame #3 {
                    w538 = 1 ("dimension size")
                    w542 = 1
                    # "Read in latest scalar card data from \n'Scalar Data' global variable that \nscaler.vi is writing to, then wait 1 sec\nfor next batch of data"
                    # "Plotting the normalized relative \nbackscatter"
                    # "Calculating the normalized relative backscatter"
                    # "Calculating/Plotting smoothed data,\ncross sections etc."
                    # "Pick off data with\nout header"
                    # "Calculate mean bin by bin mean"
                    # "Reading in 'Integration Period (Seconds)' of data"
                    # "Read the offline data from the scalar card, perform smoothing, calculate normalized relative backscatter, and plot"
                    # "File path in MATLAB script is of old dial is:\nF:\\Micropulse DIAL\\Micropulse DIAL Matlab\\\nFinal Overlap Function.mat')];"
                    # "Collects Data From Card,\nSends It To The Chart,\nAnd Saves A Copy As A\nFile If Option Selected On\nFront Panel"
                    n384 = for {
                      N: "Data Reads (number of loops)" -> [_]
                      tunnel: [w574] -> w506 mode=indexing
                      tunnel: [w573] -> w505 mode=indexing
                      n385 = global read "AMCS_Data.vi" "AMCS_Data"() -> (w575:u16[][])
                      n386 = disable-structure shown="Disabled" {
                        frame Disabled {
                          n387 = global read "Scalar_Data_4.vi" "Scalar Data 4"() -> ()  [unwired: 1 out]
                          n388 = global read "Scalar_Data_2.vi" "Scalar Data 2"() -> ()  [unwired: 1 out]
                        }
                        frame Enabled {
                        }
                      }
                      n389 = Index Array(array=w575, index (row) #1=1 ("index (row)"), index (row) #2=3 ("index (row)")) -> (element #1=w574:u16[], element #2=w573:u16[])  [unwired: 2 in]
                    }
                    n390 = local read "Total DIAL Integration Time (Minutes)"() -> (w563:i32)
                    n391 = Divide(x=w563, y="Data Reads (number of loops)") -> (x/y=w561:dbl)
                    n392 = local read "Total Aerosol Integration Time (Minutes)"() -> (w565:dbl)
                    n393 = local read "background length"() -> (w510:i32)
                    n394 = Multiply(x=w561, y=60.0) -> (x*y=w548:dbl)
                    n395 = local read "background start"() -> (w511:u32)
                    n396 = Transpose 2D Array(2D array=w506) -> (transposed array=w571:u16[][])
                    n397 = Transpose 2D Array(2D array=w505) -> (transposed array=w554:u16[][])
                    n398 = Divide(x=w565, y="Data Reads (number of loops)") -> (x/y=w566:dbl)
                    n399 = for {
                      tunnel: w571 -> [w581] mode=indexing
                      tunnel: [w580] -> w572 mode=indexing
                      tunnel: w554 -> [w579] mode=indexing
                      tunnel: [w578] -> _ mode=indexing
                      tunnel: [w578] -> w551 mode=indexing
                      n400 = call-poly <vilib>:"Mean.vi"("X"=w581) -> ("mean"=w580:dbl)  [unwired: 1 out]
                      n401 = call-poly <vilib>:"Mean.vi"("X"=w579) -> ("mean"=w578:dbl)  [unwired: 1 out]
                    }
                    n402 = local read "bins"() -> (w539:u32)
                    n403 = Multiply(x=w566, y=60.0) -> (x*y=w529:dbl)
                    n404 = Array Subset(array=w551, index=w538, length=w539) -> (w552:dbl[])
                    "Off-Line Bin Readings 2" <- w552
                    n405 = Array Subset(array=w572, index=w538, length=w539) -> (w550:dbl[])
                    "Off-Line  Bin Readings" <- w550
                    n406 = Array Subset(array=w552, index=w511, length=w510) -> (w553:dbl[])
                    n407 = Array Subset(array=w550, index=w511, length=w510) -> (w570:dbl[])
                    n408 = local read "Smoothed Bins"() -> (w507:dbl)
                    n409 = call-poly <vilib>:"Mean.vi"("X"=w553) -> ("mean"=w517:dbl)  [unwired: 1 out]
                    n410 = call-poly <vilib>:"Mean.vi"("X"=w570) -> ("mean"=w518:dbl)  [unwired: 1 out]
                    n411 = local read "Index"() -> (w528:i32)
                    n412 = Subtract(x=w552, y=w517) -> (x-y=w530:dbl[])
                    n413 = Subtract(x=w550, y=w518) -> (x-y=w546:dbl[])
                    n414 = call "Ring Buffer Offline Far.vi"("Index"=w528, "Profiles to Average"=w548, "Input Array"=w546) -> ("AvgArray"=w568:dbl[], "RingBufferOut"=→"RingBuffer offline far":dbl[][])  [unwired: 7 in]
                    n415 = call "Ring Buffer Aerosol Far.vi"("Index"=w528, "Profiles to Average"=w529, "Input Array"=w546) -> ("AvgArray"=w564:dbl[], "RingBufferOut"=→"RingBuffer aerosol far":dbl[][])  [unwired: 7 in]
                    n416 = call "Ring Buffer Offline Near.vi"("Index"=w528, "Profiles to Average"=w548, "Input Array"=w530) -> ("AvgArray"=w549:dbl[], "RingBufferOut"=→"RingBuffer offline near":dbl[][])  [unwired: 7 in]
                    n417 = call "Ring Buffer Aerosol Near.vi"("Index"=w528, "Profiles to Average"=w529, "Input Array"=w530) -> ("AvgArray"=w526:dbl[], "RingBufferOut"=→"RingBuffer aerosol near":dbl[][])  [unwired: 7 in]
                    n418 = Reshape Array(w546, w538, w539) -> (→"raw counts":dbl[][])
                    n419 = Reshape Array(w530, w538, w539) -> (→"raw counts near":dbl[][])
                    n420 = call "Smooth Arrray.vi"("smooth size"=w507, "Raw Array"=w568) -> ("Smoothed Array"=→"Off-Line Smoothed":dbl[])  [unwired: 9 in]
                    n421 = call "Smooth Arrray.vi"("smooth size"=w507, "Raw Array"=w564) -> ("Smoothed Array"=w537:dbl[])  [unwired: 9 in]
                    "Aerosol Smoothed" <- w537
                    n422 = call "Smooth Arrray.vi"("smooth size"=w507, "Raw Array"=w549) -> ("Smoothed Array"=→"Off-Line Smoothed 2":dbl[])  [unwired: 9 in]
                    n423 = call "Smooth Arrray.vi"("smooth size"=w507, "Raw Array"=w526) -> ("Smoothed Array"=w509:dbl[])  [unwired: 9 in]
                    "Aerosol Smoothed 2" <- w509
                    n424 = local read "Number of Accumulates"() -> (w513:u32)
                    n425 = local read "Temperature (C)"() -> (w560:dbl)
                    n426 = local read "Pressure (mb)"() -> (w559:dbl)
                    n427 = script code="%accum_num=10000;     % scaler card setting number of accumulations\nt_bin = 500e-9                 % scaler card setting time per bin\n%t_d = 37.3e-9;                % APD dead time from spec sheet\n\n% conversion from accumulated counts to count rate  (c/s)\nc_convert = 1./t_bin./accum_num;\nCR_far = p_raw_far.*c_convert;\nCR_near = p_raw_near.*c_convert;\nCR_total_far = (p_raw_far+b_far).*c_convert;\nCR_total_near = (p_raw_near+b_near).*c_convert;\nb_CR_far =b_far.*c_convert;\nb_CR_near =b_near.*c_convert;\n\n% create a range array\nsize_p =  size(p_raw_far,2);\nr = (75:75:size_p*75)./1e3; \n    \n%APD correction factor\n D_far = 1./(1-(t_d*CR_total_far));\n D_near = 1./(1-(t_d*CR_total_near));\n\n %Calculating normalize relative backscatter profile\n nrb_far = CR_far.*D_far.*r.^2./E.*1e-6;\n nrb_near = CR_near.*D_near.*r.^2./E.*1e-6;"("E"=6.0 ("Real"), "temp"=w560, "press"=w559, "p_raw_far"=w537, "b_far"=w518, "b_near"=w517, "p_raw_near"=w509, "accum_num"=w513, "t_d"="dead time") -> ("nrb_far"=w532:cdb[], "D_far"=w523:dbl[], "nrb_near"=w531:cdb[], "D_near"=w522:dbl[], "b_CR_far"=w515:dbl, "b_CR_near"=w514:dbl)  [unwired: 1 in, 1 out]
                    n428 = local read "bins"() -> (w541:u32)
                    n429 = local read "Altitude Array (km)"() -> (w534:dbl[])
                    n430 = Bundle(w515, w514) -> (→"?":cluster{dbl, dbl})  [unwired: 1 in]
                    n431 = Build Array(w532, w531) -> (w536:cdb[][])
                    n432 = Build Array(w523, w522) -> (w521:dbl[][])
                    n433 = Reshape Array(w531, w542, w541) -> (→"NRB 2":cdb[][])
                    n434 = Reshape Array(w532, w542, w541) -> (→"NRB":cdb[][])
                    n435 = Build Array(w534, w534) -> (w533:dbl[][])
                    n436 = call "Convert to Dynamic Data7"("2D Array"=w521) -> ("Dynamic Data Type"=w520:dynamicdata)  [unwired: 3 in]
                    n437 = call "Convert to Dynamic Data3"("2D Array"=w536) -> ("Dynamic Data Type"=w535:dynamicdata)  [unwired: 3 in]
                    n438 = call "Convert to Dynamic Data4"("2D Array"=w533) -> ("Dynamic Data Type"=w524:dynamicdata)  [unwired: 3 in]
                    n439 = call "Build XY Graph2"("Y Input"=w524, "X Input"=w535) -> ("XY Graph"=→"NRB plot":cluster{"Y":dbl[], "Y":dbl[]}[])  [unwired: 3 in, 6 out]
                    n440 = call "Build XY Graph4"("Y Input"=w524, "X Input"=w520) -> ("XY Graph"=→"Correction":cluster{"Y":dbl[], "Y":dbl[]}[])  [unwired: 3 in, 6 out]
                  }
                  frame #4 {
                    # "REPLACE WITH NEW AGILTRON TASK!"
                    # "Toggle Agiltron switch to online DBR"
                    n441 = disable-structure shown="Disabled" {
                      frame Disabled {
                        # "ABSORBING"
                        n442 = flat-sequence {
                          frame #0 {
                            # "Third one"
                            # "Command the switch to switch to position 1\ncorresponding to the online DBR"
                            # "Hex string command \ncorrespond to online"
                            n443 = local read "Switch Comm Port"() -> (w585:refnum<visa-resource-name>)
                            n444 = VISA Write(VISA resource name=w585, write buffer="\u0001\u0012\u0000\u0002") -> ()  [unwired: 1 in, 3 out]
                          }
                        }
                        n445 = Build Array(FALSE ("Boolean")) -> (w584:bool[])
                        n446 = call-poly <vilib>:"DAQmx Write.vi"("task/channels in"=refnum<k21> "AgiltronSwitch", "data"=w584) -> ()  [unwired: 11 in, 3 out]
                      }
                      frame Enabled {
                      }
                    }
                  }
                  frame #5 {
                    # "If 'Save Data?' is true, save all relavant offline info"
                    n447 = local read "Save Data?"() -> (w587:bool)
                    n448 = case shown="True" w587 {
                      frame False {
                        # "'Save Data?' is false, do nothing"
                      }
                      frame True {
                        # "Write only one data file at this time"
                        # "Retrive Julian Date"
                        # "'Save Data?' is true, save offline data to the Data Disk"
                        n449 = local read "Lambda Off DBR Current"() -> (w609:dbl)
                        n450 = local read "Off-Line Bin Readings 2"() -> (w606:dbl[])
                        n451 = local read "Lambda Off Read (nm)"() -> (w608:dbl)
                        n452 = local read "Off-Line  Bin Readings"() -> (w614:dbl[])
                        n453 = local read "Relative Humdity (%)"() -> (w613:dbl)
                        n454 = local read "Offline Pulse Energy"() -> (w610:dbl)
                        n455 = local read "Temperature (C)"() -> (w611:dbl)
                        n456 = local read "Pressure (mb)"() -> (w612:dbl)
                        n457 = call "Julian_Date_2.vi"() -> ("Julian Date"=w607:dbl)  [unwired: 11 in]
                        n458 = Build Array (concatenate)(w607, w608, w609, w610, w611, w612, w613, w614) -> (w592:dbl[])
                        n459 = Build Array (concatenate)(w607, w608, w609, w610, w611, w612, w613, w606) -> (w589:dbl[])
                        n460 = local read "FF_Off_Ref"() -> (w594:refnum<file>)
                        n461 = local read "NF_Off_Ref"() -> (w591:refnum<file>)
                        n462 = local read "FF_Off_Ptr"() -> (w593:i64)
                        n463 = local read "NF_Off_Ptr"() -> (w590:i64)
                        n464 = Set File Position(offset (in bytes) (0)=w593, refnum=w594) -> (refnum out=w605:refnum<file>, error out=w603:errorcluster)  [unwired: 2 in]
                        n465 = Set File Position(offset (in bytes) (0)=w590, refnum=w591) -> (refnum out=w601:refnum<file>, error out=w599:errorcluster)  [unwired: 2 in]
                        n466 = Write to Binary File(file (use dialog)=w605, data=w592, error in=w603, 5:FALSE ("prepend array or string size? (T)")) -> (refnum out=w604:refnum<file>, error out=w602:errorcluster)  [unwired: 2 in, 1 out]
                        n467 = Write to Binary File(file (use dialog)=w601, data=w589, error in=w599, 5:FALSE ("prepend array or string size? (T)")) -> (refnum out=w600:refnum<file>, error out=w598:errorcluster)  [unwired: 2 in, 1 out]
                        n468 = Get File Position(4:w602, 7:w604) -> (2:w595:i64)  [unwired: 2 out]
                        n469 = Get File Position(4:w598, 7:w600) -> (2:w588:i64)  [unwired: 2 out]
                        n470 = local write "FF_Off_Ptr"(w595) -> ()
                        n471 = local write "NF_Off_Ptr"(w588) -> ()
                      }
                    }
                  }
                }
              }
              frame #4 {
                n472 = First Call?() -> (First Call?: T/F=w617:bool)
                n473 = Or(x="calculate absorption cross sections", y=w617) -> (x .or. y?=w615:bool)
                n474 = case shown="True" w615 {
                  frame False {
                  }
                  frame True {
                    # "calculate absorption cross sections from HITRAN data base"
                    n475 = local read "Off-Line Smoothed"() -> (w618:dbl[])
                    n476 = local read "Lambda On Read (nm)"() -> (w621:dbl)
                    n477 = local read "Lambda Off Set (nm)"() -> (w624:dbl)
                    n478 = local read "Temperature (C)"() -> (w622:dbl)
                    n479 = local read "Pressure (mb)"() -> (w623:dbl)
                    n480 = script code="%Importing HITRAN data\n%hitran = dlmread('C:\\Users\\H2ODial\\Desktop\\Shared Telescope WV DIAL Code\\Libraries and VIs\\824nm_841nm_H2O.csv', ',',[0 1 352 7]);\nhitran = dlmread('C:\\Users\\H2ODial\\Desktop\\Shared Telescope WV DIAL Code\\Libraries and VIs\\824nm_841nm_H2O_Spectral_Calc.csv', ',',[1 1 1209 7]);\n\n%Range vector in meters\nrange = ([75:75:size(Online,2)*75]);\n\nif lambda< 828\nlambda=828.195;\nelse\nlambda=lambda;\nend;\n\n%%\n\n%Voigt profile calculation\nWNmin = 12070.0;\nWNmax = 12076.0;\n\n%Find lines from WNmin to WNmax to calculate voigt profile\nline_indices = find(hitran(1:size(hitran,1),1)>WNmin & hitran(1:size(hitran,1),1)<WNmax);\n\nline = (hitran(line_indices, 1:size(hitran,2)));\n\n%Calculate temperature and pressure profile\nT0 = 273+15.6;\nT0 = 273+T0_C;\n\nT = T0-0.005545.*range; \n\nP0  = 1.0;\nP0  = P0_mb/1000*0.986; %pressure in mb converted to atm\n\nP = P0.*(T0./T).^-5.21986;\n\n%linewidth temperature dependence factor\nalpha = line(:,7);        \n\n%initial Lorentz linewidth from HiTRAN [cm^-1]\ngammal0 = line(:,4);     \n\n%ground state transition energy [cm^-1]\nE = line(:,6);           \n\n%initial linestrength from HiTRAN [cm^-1/(mol*cm^-2)]\nS0 = line(:,2);      \n\n%absorption line center wavenumber from HiTRAN [cm^-1]\nnu0_0 = line(:,1);    \n\nnu_on = (1/(lambda)*1e7);\n\nnu_off = (1/(lambda_off)*1e7);\n\n\nfor i = 1:size(Online,2);\n\n    %Pressure shift\n    nu0 = nu0_0-.0428.*P(i);\n    \n    %Calculate Lorentz lineweidth at temperature T [cm^-1]\n    gammal = gammal0.*(P(i)./P0).*((T0./T(i)).^alpha);\n    \n    %Calculate Doppler linewidth at temperature T [cm^-1]\n    gammad = (nu0).*((2.0.*1.38E-23.*T(i).*log(2.0))./(0.018.*3.0E8.*3.0E8./6.022E23)).^(0.5);\n    \n    y = (gammal./gammad).*((log(2.0)).^(0.5));\n    \n    x_on = ((nu_on-nu0)./gammad).*(log(2.0)).^(0.5);\n    \n    x_off = ((nu_off-nu0)./gammad).*(log(2.0)).^(0.5);\n    \n    %setting up Voigt convolution\n    stepsize = 1;\n    \n    t = [-200:1:199].*stepsize;\n    \n    t = repmat(t',1,length(x_on))';\n    \n    x_on = repmat(x_on,1,length(t));\n    \n    x_off = repmat(x_off,1,length(t));\n    \n    y = repmat(y,1,length(t));\n    \n    f_on = (exp(-t.^2.0))./(y.^2.0+(x_on-t).^2.0);\n    \n    f_off = (exp(-t.^2.0))./(y.^2.0+(x_off-t).^2.0);\n    \n    %Set the integration sum to zero to start\n    integral_on = 0.0;\n    \n    integral_off = 0.0;\n    \n    %Voigt integration\n    z_on = trapz(t(1,:),f_on,2);\n    \n    z_off =  trapz(t(1,:),f_off,2);\n    \n    integral_on = z_on;\n    \n    integral_off = z_off;\n    \n    %Calculate linestrength at temperature T\n    S = S0.*((T0./T(i)).^(1.5)).*exp(1.439.*E.*((1./T0)-(1./T(i))));\n    \n    %Calculate Doppler line-center cross section [cm^2]\n    K = (S./gammad).*(((log(2.0))./pi).^(0.5));\n    \n    %Calculate the Voigt profile\n    V_on = (y(1)/pi).*integral_on;\n    \n    V_off = (y(1)./pi).*integral_off;\n    \n    %Calculate the Voigt profile absorption cross section [cm^2]\n    sigmav_on = K.*V_on;\n    \n    sigmav_off = K.*V_off;\n    \n    %Sum contributions from all of the surrounding lines\n    sigma_on_total(i) = sum(sigmav_on);\n    \n    sigma_off_total(i) = sum(sigmav_off);\n    \nend;"("lambda"=w621, "lambda_off"=w624, "P0_mb"=w623, "T0_C"=w622, "Online"=w618) -> ("sigma_on_total"=→"sigma_on_total":dbl[], "sigma_off_total"=→"sigma_off_total":dbl[])  [unwired: 1 in, 1 out]
                  }
                }
              }
              frame #5 {
                w635 = 1
                # "normalization factor\nfrom 300 to 450m"
                # "OPTICAL DEPTH PLOT"
                # "new rainbow color bar display"
                # "Data Processing Far Channel"
                # "new rainbow color bar display"
                # "Calculating the range resolved water vapor number density and plotting"
                n481 = local read "sigma_off_total"() -> (w658:dbl[])
                n482 = local read "sigma_on_total"() -> (w655:dbl[])
                n483 = local read "On-Line  Smoothed"() -> (w633:dbl[])
                n484 = local read "Off-Line Smoothed"() -> (w632:dbl[])
                n485 = local read "Off-Line Smoothed 2"() -> (w656:dbl[])
                n486 = local read "On-Line Smoothed 2"() -> (w657:dbl[])
                n487 = script code="%Time averaging in seconds.  600 Seconds =10 minutes\ntemporal_average = 600;\n\n%Spatial averaging in bins.  2 bins = 150 meters\nspatial_average = 2;\n\n%Creating r and r+deltar vectors..this can also be acsomplished using the\n%diff command\np_oni = Online(:,1:size(Online,2)-1);\n\np_onii = Online(:,2:size(Online,2));\n\np_offi = Offline(:,1:size(Offline,2)-1);\n\np_offii = Offline(:,2:size(Offline,2));\n\nInside = (p_oni.*p_offii)./(p_onii.*p_offi);\n\ndel_cross = 1./(2.*(sigma_on_total(1:size(Online,2)-1)-sigma_off_total(1:size(Offline,2)-1)).*75*100);\n\ndel_cross(isinf(del_cross)) = 0;\n\n%Calculating Number density\nN = del_cross.*log(Inside);\n\n%Spatial smoothing of the profiles\nfilter1 = ones(1,2)./2;\n\nN_1 = N;\n\nN_1_avg = filter2(filter1,N_1);\n\nfilter1 = ones(1,10)./10;\n\nN_2 = N;\n\nN_2_avg = filter2(filter1,N_2);\n\nN_new = zeros(size(N,1),size(N,2));\n \n%Using different averaging windows for different altitudes \nN_avg=[N_1_avg(:,1:40)';N_2_avg(:,41:size(N,2))']';\n\n\nw = N_avg.*1e6.*18.015./6.022e23"("Online"=w657, "Offline"=w656, "sigma_on_total"=w655, "sigma_off_total"=w658) -> ("N_avg"=w659:cdb[], "w"=w668:cdb[])  [unwired: 1 in, 1 out]
                n488 = script code="%Time averaging in seconds.  600 Seconds = 10 minutes\ntemporal_average = 600;\n\n%Spatial averaging in bins.  2 bins = 150 meters\nspatial_average = 2;\n\n%Creating r and r+deltar vectors..this can also be acsomplished using the\n%diff command\np_oni = Online(:,1:size(Online,2)-1);\n\np_onii = Online(:,2:size(Online,2));\n\np_offi = Offline(:,1:size(Offline,2)-1);\n\np_offii = Offline(:,2:size(Offline,2));\n\nInside = (p_oni.*p_offii)./(p_onii.*p_offi);\n\ndel_cross = 1./(2.*(sigma_on_total(1:size(Online,2)-1)-sigma_off_total(1:size(Offline,2)-1)).*75*100);\n\ndel_cross(isinf(del_cross)) = 0;\n\n%Calculating Number density\nN = del_cross.*log(Inside);\n\n%Spatial smoothing of the profiles\nfilter1 = ones(1,2)./2;\n\nN_1 = N;\n\nN_1_avg = filter2(filter1,N_1);\n\nfilter1 = ones(1,10)./10;\n\nN_2 = N;\n\nN_2_avg = filter2(filter1,N_2);\n\nN_new = zeros(size(N,1),size(N,2));\n \n%Using different averaging windows for different altitudes \nN_avg=[N_1_avg(:,1:40)';N_2_avg(:,41:size(N,2))']';\n\n \nw = N_avg.*1e6.*18.015./6.022e23"("Online"=w633, "Offline"=w632, "sigma_on_total"=w655, "sigma_off_total"=w658) -> ("N_avg"=w664:cdb[], "w"=w665:cdb[])  [unwired: 1 in, 1 out]
                n489 = local read "Time Resolution Per Bin(ns)"() -> (w634:u32)
                n490 = local read "bins"() -> (w660:u32)
                n491 = local read "Altitude Array (km)"() -> (w630:dbl[])
                n492 = Build Array(w665, w668) -> (w671:cdb[][])
                n493 = To Double Precision Float(number=w634) -> (double precision float=w653:dbl)
                n494 = Reshape Array(w664, w635, w660) -> (w675:cdb[][])
                n495 = Reshape Array(w659, w635, w660) -> (w662:cdb[][])
                n496 = Multiply(x=0.15, y=w653) -> (x*y=w651:dbl)
                n497 = Build Array(w664, w659) -> (w669:cdb[][])
                n498 = Divide(x=300.0, y=w651) -> (x/y=w648:dbl)
                n499 = Divide(x=450.0, y=w651) -> (x/y=w647:dbl)
                n500 = Build Array(w630, w630) -> (w654:dbl[][])
                n501 = call "Convert to Dynamic Data5"("2D Array"=w671) -> ("Dynamic Data Type"=w670:dynamicdata)  [unwired: 3 in]
                n502 = call "Convert to Dynamic Data2"("2D Array"=w669) -> ("Dynamic Data Type"=w666:dynamicdata)  [unwired: 3 in]
                n503 = Divide(x=w675, y=1e+17) -> (x/y=→"Water Vapor Number Density":cdb[][])
                n504 = Divide(x=w662, y=1e+17) -> (x/y=→"Water Vapor Number Density 2":cdb[][])
                n505 = call "Convert to Dynamic Data6"("Array"=w630) -> ("Dynamic Data Type"=w631:dynamicdata)  [unwired: 3 in]
                n506 = To Long Integer(number=w648) -> (32bit integer=w646:i32)
                n507 = To Long Integer(number=w647) -> (32bit integer=w645:i32)
                n508 = call "Convert to Dynamic Data"("2D Array"=w654) -> ("Dynamic Data Type"=w667:dynamicdata)  [unwired: 3 in]
                n509 = call "Convert to Dynamic Data8"("2D Array"=w654) -> ("Dynamic Data Type"=w672:dynamicdata)  [unwired: 3 in]
                n510 = Decrement(x=w646) -> (x-1=w643:i32)
                n511 = Decrement(x=w645) -> (x-1=w644:i32)
                n512 = call "Build XY Graph"("Y Input"=w667, "X Input"=w666) -> ("XY Graph"=→"Water Vapor Number Density  2":cluster{"Y":dbl[], "Y":dbl[]}[])  [unwired: 3 in, 6 out]
                n513 = call "Build XY Graph3"("Y Input"=w672, "X Input"=w670) -> ("XY Graph"=→"Absolute Humidity":cluster{"Y":dbl[], "Y":dbl[]}[])  [unwired: 3 in, 6 out]
                n514 = Array Subset(array=w633, index=w643, length=w644) -> (w642:dbl[])
                n515 = Array Subset(array=w632, index=w643, length=w644) -> (w641:dbl[])
                n516 = call-poly <vilib>:"Mean.vi"("X"=w642) -> ("mean"=w640:dbl)  [unwired: 1 out]
                n517 = call-poly <vilib>:"Mean.vi"("X"=w641) -> ("mean"=w639:dbl)  [unwired: 1 out]
                n518 = Divide(x=w640, y=w639) -> (x/y=w638:dbl)
                n519 = Multiply(x=w632, y=w638) -> (x*y=w637:dbl[])
                n520 = Divide(x=w633, y=w637) -> (x/y=w636:dbl[])
                n521 = Natural Logarithm(1:w636) -> (0:w627:dbl[])
                n522 = Multiply(x=-1.0, y=w627) -> (x*y=w626:dbl[])
                n523 = call "Convert to Dynamic Data9"("Array"=w626) -> ("Dynamic Data Type"=w629:dynamicdata)  [unwired: 3 in]
                n524 = call "Build OD Plot"("Y Input"=w631, "X Input"=w629) -> ("XY Graph"=→"Optical Depth":cluster{"Y":dbl[], "Y":dbl[]}[])  [unwired: 3 in, 6 out]
              }
            }
          }
        }
        "L_Count" <- w130
      }
    }
  }
  n525 = case shown="True" w3 {
    frame False {
    }
    frame True {
      # "close data files"
      n526 = local read "NF_Off_Ref"() -> (w679:refnum<file>)
      n527 = local read "NF_On_Ref"() -> (w680:refnum<file>)
      n528 = local read "FF_Off_Ref"() -> (w681:refnum<file>)
      n529 = local read "FF_On_Ref"() -> (w682:refnum<file>)
      n530 = local read "WS_On/Off"() -> (w678:bool)
      n531 = case shown="True" w678 {
        frame False {
        }
        frame True {
          n532 = local read "WS visa"() -> (w683:refnum<visa-resource-name>)
          n533 = call "T_RH_P.vi"("VISA in"=w683, "WS_Commands"=enum16{"OpenWS", "ReadTRHP", "CloseWS"}."CloseWS") -> ()  [unwired: 11 in, 3 out]
        }
      }
      n534 = Close File(refnum=w682) -> ()  [unwired: 1 in, 2 out]
      n535 = Close File(refnum=w681) -> ()  [unwired: 1 in, 2 out]
      n536 = Close File(refnum=w680) -> ()  [unwired: 1 in, 2 out]
      n537 = Close File(refnum=w679) -> ()  [unwired: 1 in, 2 out]
    }
  }
  "FileHour" <- -1 ("FileHour")
  "DataOpen" <- FALSE
